vi "FPGA Beam Scanning V1.vi"(1 "Detectors":T1, 2 "Image Acquisition Parameters":T2={"Scan Type"=enum."Sample Scanning", "Scan Mode"=enum."XY", "Fast Axis Frequency (Hz)"=100.0, "Image Format"=128, "Line Accumulations"=1, "Frames Per Capture"=1, "Frames Accumulations"=1, "Image Dimension (um)"=[], "Number of Z Steps"=1, "Z Steps Size (um)"=1.0, "Pixel Size (nm)"=[]} {"Z Steps Size (um)" min=0.0; "Number of Z Steps" min=1; "Frames Accumulations" min=1; "Frames Per Capture" min=1; "Line Accumulations" min=1; "Image Format" items=["64 x 64"=64, "128 x 128"=128, "256 x 256"=256, "512 x 512"=512, "1024 x 1024"=1024, "2048 x 2048"=2048]}) -> ()   [LabVIEW 2016]
uses:
  <vilib>/rvi/interface/nirviReadWriteControl/nirviReadWriteControl.xnode
  <vilib>/rvi/interface/nirviMethod/nirviMethod.xnode
  <vilib>/rvi/errors/niLvFpgaMergeErrorWithErrorCode.vi
  <vilib>/rvi/interface/nirviOpenFPGA/nirviOpenFPGA.xnode
  <vilib>/vision/NI_Vision_Development_Module.lvlib
  <vilib>/rvi/interface/nirviCloseFPGA/nirviCloseFPGA.xnode
  <vilib>/vision/Image Controls.llb/IMAQ Image.ctl
  FPGA Bitfiles/MainSTEDFPGAProj_FPGATarget2_BeamScanningCamb_PyGckhW3v70.lvbitx
  FPGA Target VIs/FPGA-7852R/Beam Scanning Cambridge V1.vi
  <vilib>/FPGAPlugInAG/PCIe-7852R/niLvFpga_Open_PCIe-7852R.vi
  NiFpgaLv.dll
  <vilib>/Utility/error.llb/Error Cluster From Error Code.vi
  <vilib>/rvi/errors/niLvFpgaAdjustHostInterfaceError.vi
  <vilib>/FPGAPlugInAG/PCIe-7852R/niLvFpga_ConfigureFifo_PCIe-7852R.vi
  <vilib>/FPGAPlugInAG/PCIe-7852R/niLvFpga_StartFifo_PCIe-7852R.vi
  <vilib>/FPGAPlugInAG/PCIe-7852R/niLvFpga_ReadFifo_PCIe-7852R.vi
  <vilib>/FPGAPlugInAG/PCIe-7852R/niLvFpga_Run_PCIe-7852R.vi
  <vilib>/FPGAPlugInAG/PCIe-7852R/niLvFpga_Close_PCIe-7852R.vi
  Type Defs/Image Acquisition Parameters.ctl
  Detectors.ctl
panel:
  in  "Trigger Delay Manual (Ticks)":u16=3650
  in  "Adjust Trigger":u16=300
  # "Copyright (C) 2020 Edward S Allgeyer\n\nRedistribution and use in source and binary forms, with or without\nmodification, are permitted provided that the following conditions\nare met:\n\n1. Redistributions of source code must retain the above copyright\n   notice, this list of conditions and the following disclaimer.\n\n2. Redistributions in binary form must reproduce the above copyright\n   notice, this list of conditions and the following disclaimer in\n   the documentation and/or other materials provided with the\n   distribution.\n\n3. Neither the name of the copyright holder nor the names of its\n   contributors may be used to endorse or promote products derived\n   from this software without specific prior written permission.\n\nTHIS SOFTWARE IS PROVIDED BY THE COPYRIGHT HOLDERS AND CONTRIBUTORS\n\"AS IS\" AND ANY EXPRESS OR IMPLIED WARRANTIES, INCLUDING, BUT NOT\nLIMITED TO, THE IMPLIED WARRANTIES OF MERCHANTABILITY AND FITNESS\nFOR A PARTICULAR PURPOSE ARE DISCLAIMED. IN NO EVENT SHALL THE\nCOPYRIGHT HOLDER OR CONTRIBUTORS BE LIABLE FOR ANY DIRECT, INDIRECT,\nINCIDENTAL, SPECIAL, EXEMPLARY, OR CONSEQUENTIAL DAMAGES (INCLUDING,\nBUT NOT LIMITED TO, PROCUREMENT OF SUBSTITUTE GOODS OR SERVICES;\nLOSS OF USE, DATA, OR PROFITS; OR BUSINESS INTERRUPTION) HOWEVER\nCAUSED AND ON ANY THEORY OF LIABILITY, WHETHER IN CONTRACT, STRICT\nLIABILITY, OR TORT (INCLUDING NEGLIGENCE OR OTHERWISE) ARISING IN\nANY WAY OUT OF THE USE OF THIS SOFTWARE, EVEN IF ADVISED OF THE\nPOSSIBILITY OF SUCH DAMAGE."
  # "XY"
  # "Z"
  # "Length"
  # "Height"
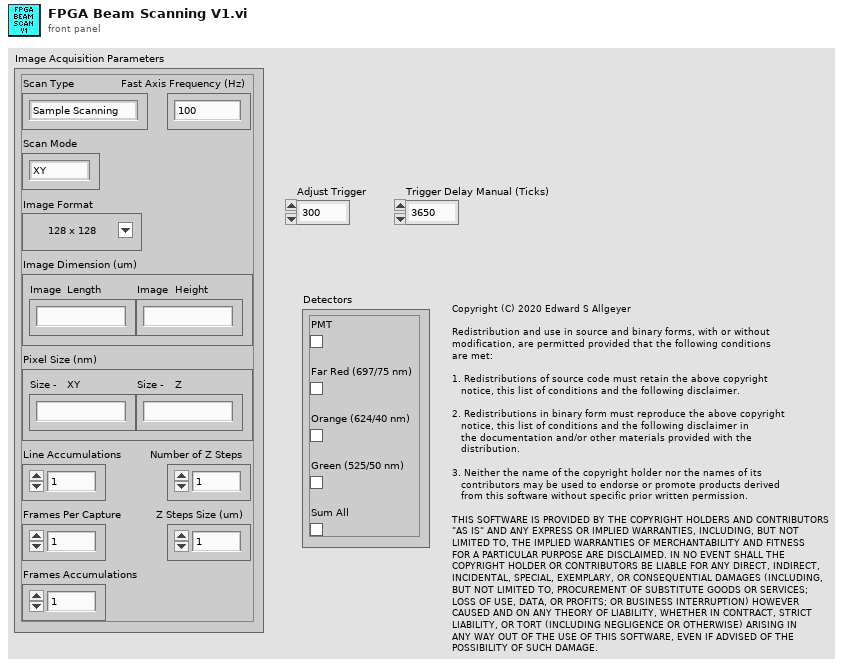
[diagram p1: front panel]
types:
  T1 = typedef "Detectors.ctl" = cluster{"PMT":bool, "Far Red (697/75 nm)":bool, "Orange (624/40 nm)":bool, "Green (525/50 nm)":bool, "Sum All":bool}
  T2 = typedef "Image Acquisition Parameters.ctl" = cluster{"Scan Type":enum16{"Sample Scanning", "Beam Scanning"}, "Scan Mode":enum16{"XY", "XZ", "YZ", "XYZ"}, "Fast Axis Frequency (Hz)":dbl, "Image Format":u16, "Line Accumulations":u16, "Frames Per Capture":u16, "Frames Accumulations":u16, "Image Dimension (um)":dbl[], "Number of Z Steps":u8, "Z Steps Size (um)":dbl, "Pixel Size (nm)":dbl[]}
  T3 = typedef "IMAQ Image.ctl" = refnum<image>
  T4 = enum16{"big-endian, network order", "native, host order", "little-endian"}
  T5 = cluster{"FPGA Sampling Period (ns)":dbl, "Counting Period (us)":dbl, "Samples Per Counting Period":i32, "Start Time (us)":dbl, "Stop Time (us)":dbl, "Normalized Scan End Position":dbl, "Normalized Scan Start Position":dbl}
  T6 = typedef "Scan Parameters.ctl" = cluster{"Fast_Ax_Amp_V":dbl, "Fast_Ax_Off_V":dbl, "Slow_Ax_Amp_V":dbl, "Slow_Ax_Off_V ":dbl, "Slow_Ax_Max_V_VperS":dbl, "Slow_Ax1_Del25ns":i32, "Slow_Ax2_Del25ns":i32, "Stage_X_Off_V":dbl, "Stage_Y_Off_V":dbl, "Stage_Z_Off_V":dbl, "Galvo1_Off_V":dbl, "Galvo2_Off_V":dbl, "Last_Scan_Mode":enum16{"XY", "XZ", "YZ", "XYZ"}, "Current_Scan_Mode":enum16{"XY", "XZ", "YZ", "XYZ"}, "Fly_Back_Lines":u16, "Linear_Ramp_End":u32, "Z_Step_I16":i16, "Z_Start_I16":i16, "Laser_States _U32":u32, "590_Voltage_I16":i16, "775_AOM_Volt_I16":i16, "Blanking OFF":bool, "Unused_Axis_I16":i16}
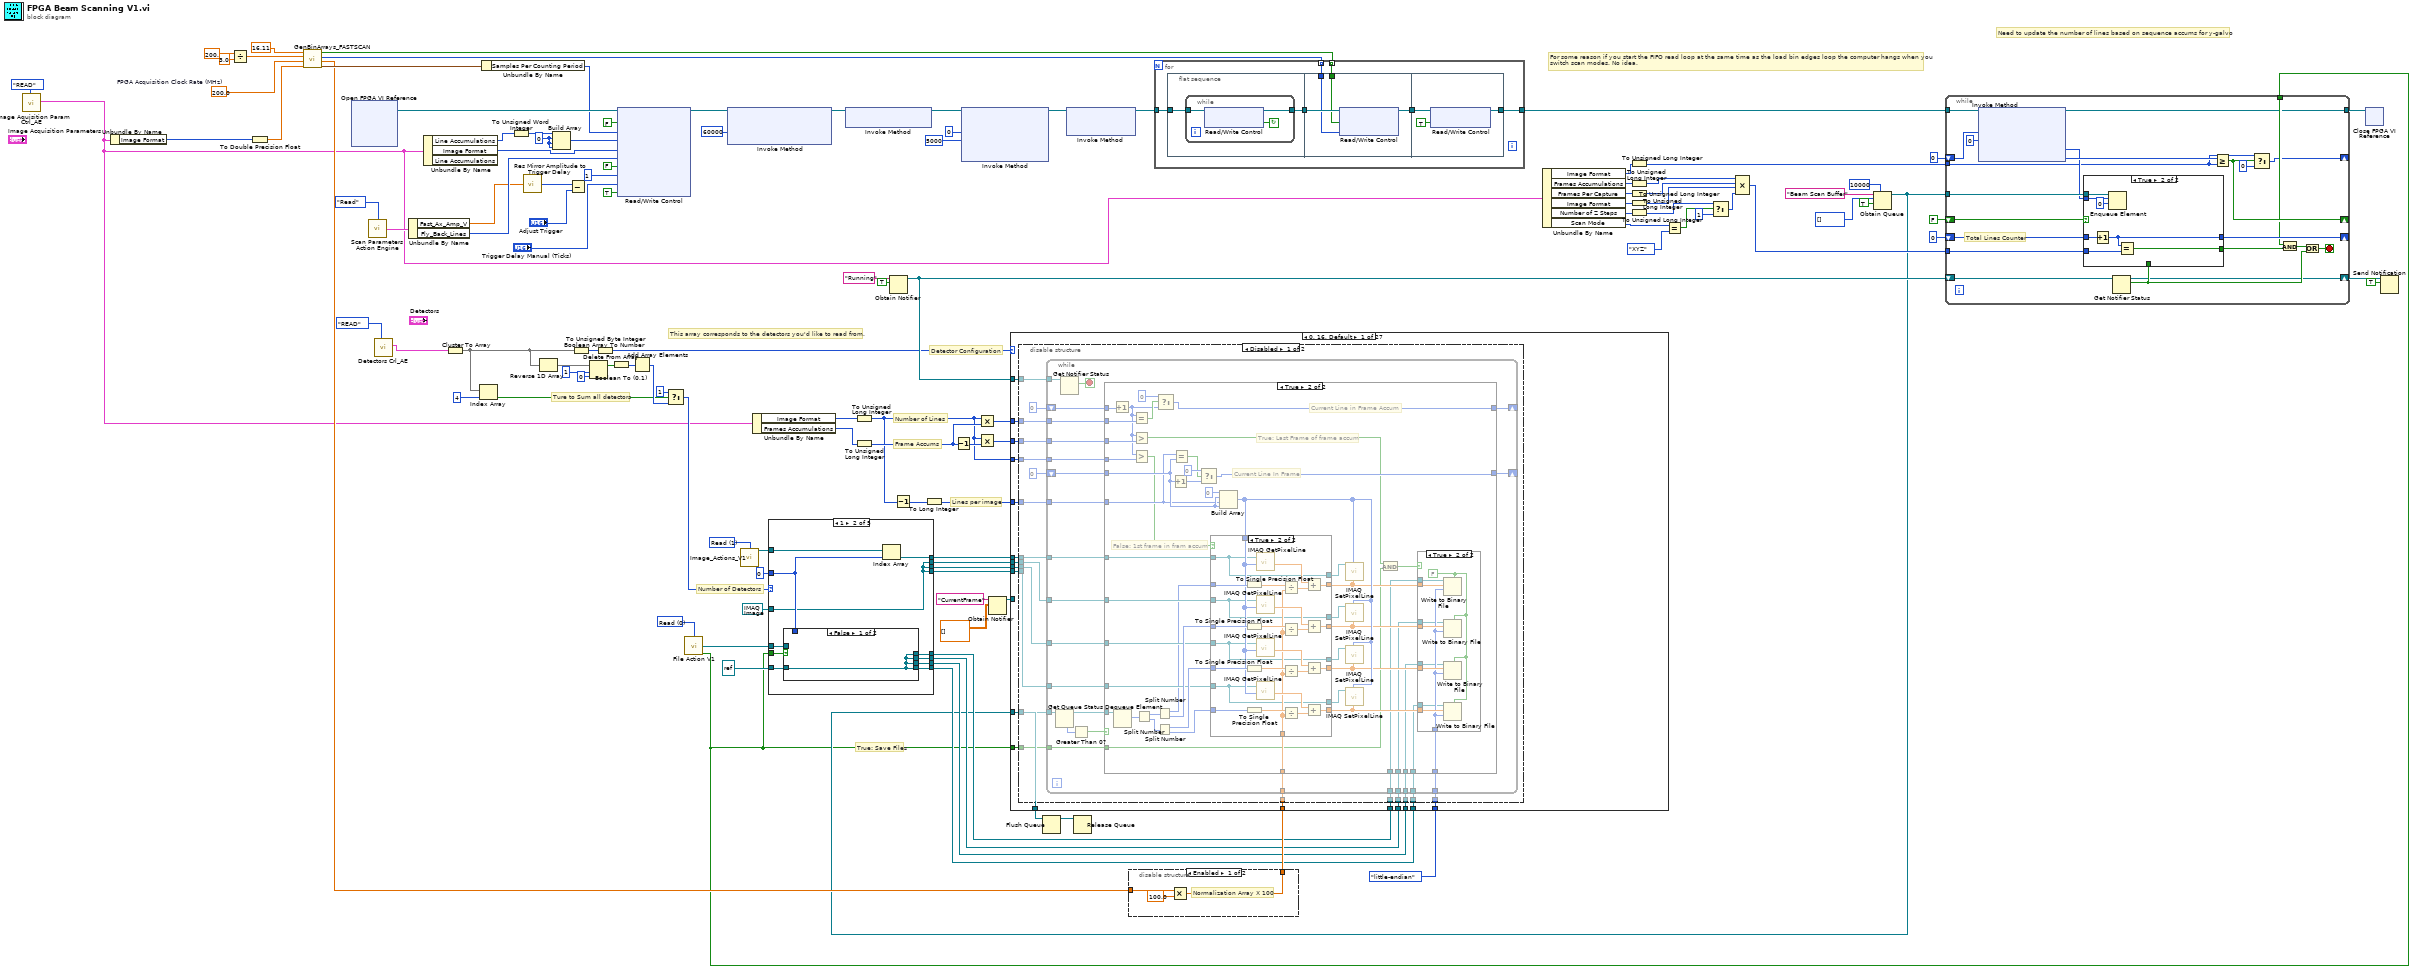
[diagram p0: block diagram]
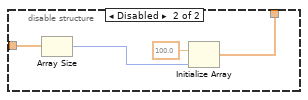
[diagram p2: hidden frame]
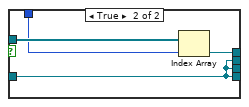
[diagram p4: hidden frame]
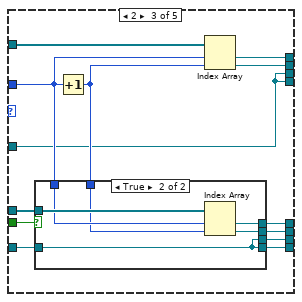
[diagram p5: hidden frame]
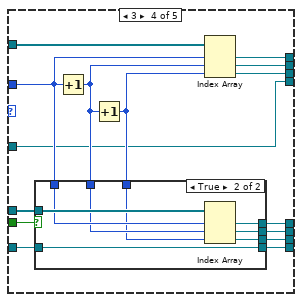
[diagram p7: hidden frame]
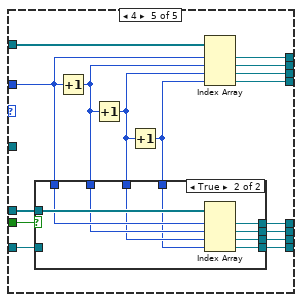
[diagram p9: hidden frame]
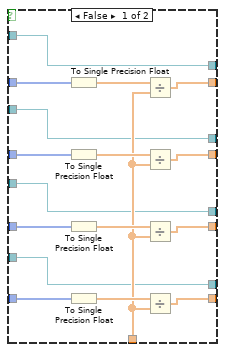
[diagram p13: hidden frame]
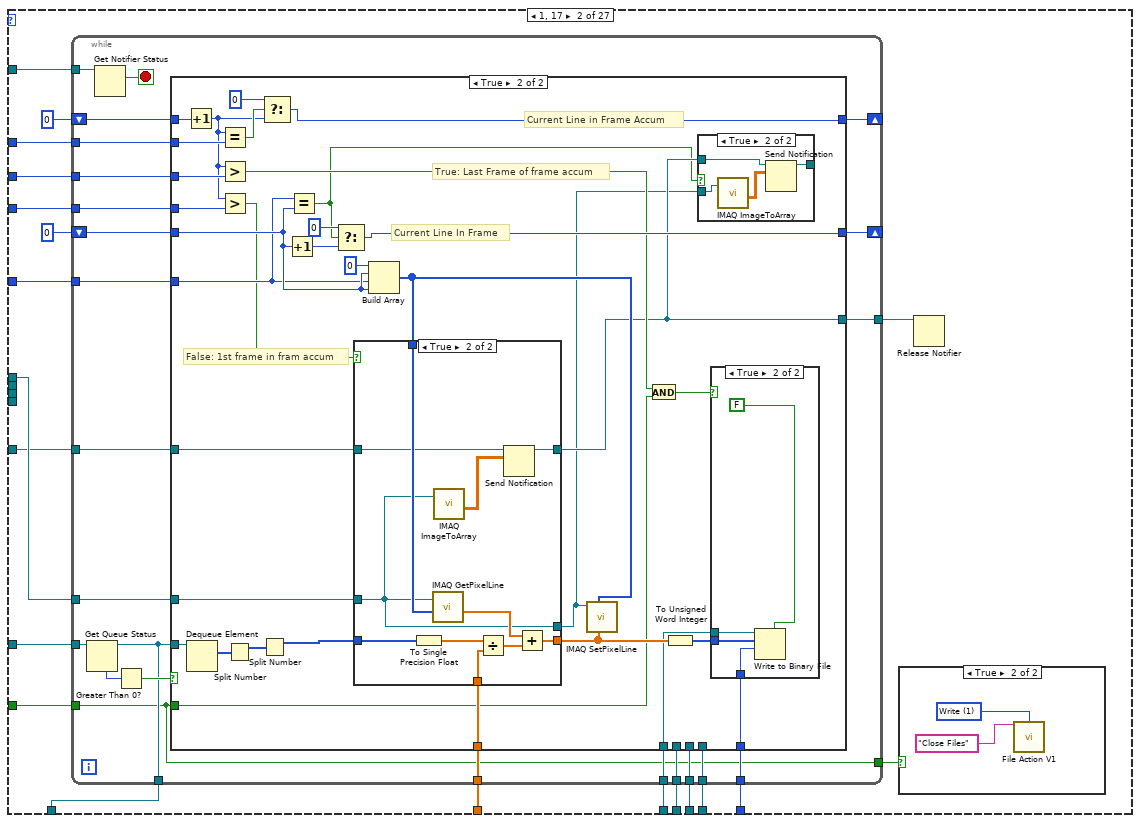
[diagram p15: hidden frame]
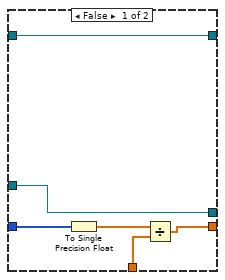
[diagram p20: hidden frame]
diagram:
  w21 = u16 0 items=["Read", "Write"] ("Mode")
  w22 = u16 0 ("element")
  w65 = u16 1 items=["Write", "Read"] ("Mode")
  w113 = 200.0  # FPGA Acquisition Clock Rate (MHz)
  # "This array corresponds to the detectors you'd like to read from."
  # "Ture to Sum all detectors"
  # "Number of Detectors"
  # "Detector Configuration"
  # "Frame Accums"
  # "Number of Lines"
  # "True: Save Files"
  # "Lines per image"
  # "For some reason if you start the FIFO read loop at the same time as the load bin edges loop the computer hangs when you\nswitch scan modes. No idea."
  # "Need to update the number of lines based on sequence accums for y-galvo"
  n1 = call "Image Aquisition Param Ctrl_AE.vi"("Action"=enum16{"READ", "WRITE"}."READ") -> ("Image Acquisition Parameters Out"=w7:T2)  [unwired: 10 in]
  n2 = Unbundle By Name(w7) -> ("Image Format"=w19:u16)
  n3 = Divide(x=200.0, y=3.0) -> (x/y=w110:dbl)
  n4 = To Double Precision Float(number=w19) -> (double precision float=w94:dbl)
  n5 = call "GenBinArrays_FASTSCAN.vi"("Pixels Per Line"=w94, "FPGA Acquisition Clock Rate (MHz)"=w113, "Collection Percent (%)"=w110, "Scan Rate (kHz)"=16.11) -> ("Reported Parameters"=w109:T5, "Normalization Array"=w43:sgl[], "Pre Binned Counts (x100)"=w16:u32[], "FPGA Bin Edges"=w17:bool[])
  n6 = xnode "Open FPGA VI Reference"() -> ("FPGA VI Reference Out"=w117:refnum<k20>)  [unwired: 2 in, 1 out]
  n7 = call "Scan Parameters Action Engine.vi"("Action"=enum16{"Read", "Write"}."Read") -> ("Scan Parameters OUT"=w27:T6)  [unwired: 14 in]
  n8 = call "Detectors Crl_AE.vi"("Action"=enum16{"READ", "WRITE"}."READ") -> ("Detectors Parameters Out"=w5:T1)  [unwired: 10 in]
  n9 = Unbundle By Name(w27) -> ("Fast_Ax_Amp_V"=w18:dbl, "Fly_Back_Lines"=w26:u16)
  n10 = Unbundle By Name(w7) -> ("Line Accumulations"=w32:u16, "Image Format"=w29:u16)  [unwired: 1 out]
  n11 = Cluster To Array(cluster=w5) -> (array=w11:bool[])
  n12 = Index Array(array=w11, index=4) -> (element=w9:bool)
  n13 = Unbundle By Name(w109) -> ("Samples Per Counting Period"=w76:i32)
  n14 = To Unsigned Word Integer(number=w32) -> (unsigned 16bit integer=w31:u16)
  n15 = call "Res Mirror Amplitude to Trigger Delay.vi"("Amplitude (V)"=w18) -> ("Trigger Delay (Ticks)"=w15:u16)
  n16 = Reverse 1D Array(array=w11) -> (reversed array=w48:bool[])
  n17 = Build Array(w31, w22, w22, w22) -> (w30:u16[])
  n18 = Subtract(x=w15, y="Adjust Trigger") -> ()  [unwired: 1 out]
  n19 = Boolean Array To Number(Boolean array=w11) -> (number=w13:u32)
  n20 = Delete From Array(array=w48, length=1, index=0) -> (array with subset deleted=w52:bool[])  [unwired: 1 out]
  n21 = To Unsigned Byte Integer(number=w13) -> (unsigned 8bit integer=w12:u8)
  n22 = Boolean To (0,1)(Boolean=w52) -> (0, 1=w51:i16[])
  n23 = xnode "Read/Write Control"("FPGA VI Reference In"=w117, "Ready For Write"=FALSE, "FPGA Samples"=w76, "Accums Per Line"=w30, "Lines Per Image"=w29, "Dead Lines"=w26, "Line Trigger"=FALSE, "Sequences"=u8 1, "Trigger Delay (Ticks)"="Trigger Delay Manual (Ticks)", "Stop Acquisition"=TRUE) -> ("FPGA VI Reference Out"=w116:refnum<k20>)  [unwired: 1 in, 1 out]
  n24 = Add Array Elements(numeric array=w51) -> (sum=w50:i16)
  n25 = Select(t=i16 1, s=w9, f=w50) -> (s? t:f=w45:i16)
  n26 = call "File Action V1.vi"("Mode"=w21) -> ("File REFs"=w62:refnum<file>[], "Files Open"=w20:bool)  [unwired: 12 in, 1 out]
  n27 = xnode "Invoke Method"("FPGA VI Reference In"=w116, "Requested Depth"=u32 60000) -> ("FPGA VI Reference Out"=w92:refnum<k20>)  [unwired: 1 in, 2 out]
  n28 = call "Image_Actions_V1.vi"("Mode"=w65) -> ("Image REFs OUT"=w64:T3[])  [unwired: 13 in, 1 out]
  n29 = Unbundle By Name(w7) -> ("Image Format"=w85:u16, "Frames Accumulations"=w84:u16)
  n30 = case shown="1" w45 {
    tunnel: [w119 w120 w136 w156 w195] -> w57
    tunnel: [w119 w120 w136 w170 w194] -> w58
    tunnel: [w119 w120 w148 w169 w193] -> w59
    tunnel: [w119 w130 w147 w168 w192] -> w60
    tunnel: 0 ("Offset") -> [_ w126 w143 w164 w188]
    tunnel: w64 -> [_ w129 w146 w167 w191]
    tunnel: T3 refnum ("New Image") -> [w119 w120 w136 w156 _]
    tunnel: w62 -> [_ w127 w144 w165 w189]
    tunnel: w20 -> [_ w128 w145 w166 w190]
    tunnel: [w118 w125 w141 w161 w184] -> w56
    tunnel: [w118 w124 w140 w160 w183] -> w55
    tunnel: [w118 w123 w139 w159 w182] -> w54
    tunnel: [w118 w122 w138 w158 w181] -> w53
    tunnel: refnum<file> refnum ("element") -> [w118 w121 w137 w157 w180]
    frame 0, Default {
    }
    frame 1 {
      n31 = case shown="False" w128 {
        tunnel: w127 -> [_ w135]
        tunnel: w126 -> [_ w134]
        tunnel: [w131 w133] -> w125
        tunnel: [w131 w132] -> w124
        tunnel: [w131 w132] -> w123
        tunnel: [w131 w132] -> w122
        tunnel: w121 -> [w131 w132]
        frame False {
        }
        frame True {
          n32 = Index Array(array=w135, index=w134) -> (element=w133:refnum<file>)
        }
      }
      n33 = Index Array(array=w129, index=w126) -> (element=w130:T3)
    }
    frame 2 {
      n34 = Increment(x=w143) -> (x+1=w142:i32)
      n35 = case shown="True" w145 {
        tunnel: w144 -> [_ w155]
        tunnel: w143 -> [_ w154]
        tunnel: w142 -> [_ w153]
        tunnel: [w149 w152] -> w141
        tunnel: [w149 w151] -> w140
        tunnel: [w149 w150] -> w139
        tunnel: [w149 w150] -> w138
        tunnel: w137 -> [w149 w150]
        frame False {
        }
        frame True {
          n36 = Index Array(array=w155, index #1=w154, index #2=w153) -> (element #1=w152:refnum<file>, element #2=w151:refnum<file>)
        }
      }
      n37 = Index Array(array=w146, index #1=w143, index #2=w142) -> (element #1=w147:T3, element #2=w148:T3)
    }
    frame 3 {
      n38 = Increment(x=w164) -> (x+1=w163:i32)
      n39 = Increment(x=w163) -> (x+1=w162:i32)
      n40 = case shown="True" w166 {
        tunnel: w165 -> [_ w179]
        tunnel: w164 -> [_ w178]
        tunnel: w163 -> [_ w177]
        tunnel: w162 -> [_ w176]
        tunnel: [w171 w175] -> w161
        tunnel: [w171 w174] -> w160
        tunnel: [w171 w173] -> w159
        tunnel: [w171 w172] -> w158
        tunnel: w157 -> [w171 w172]
        frame False {
        }
        frame True {
          n41 = Index Array(array=w179, index #1=w178, index #2=w177, index #3=w176) -> (element #1=w175:refnum<file>, element #2=w174:refnum<file>, element #3=w173:refnum<file>)
        }
      }
      n42 = Index Array(array=w167, index #1=w164, index #2=w163, index #3=w162) -> (element #1=w168:T3, element #2=w169:T3, element #3=w170:T3)
    }
    frame 4 {
      n43 = Increment(x=w188) -> (x+1=w187:i32)
      n44 = Increment(x=w187) -> (x+1=w186:i32)
      n45 = Increment(x=w186) -> (x+1=w185:i32)
      n46 = case shown="True" w190 {
        tunnel: w189 -> [_ w205]
        tunnel: w188 -> [_ w204]
        tunnel: w187 -> [_ w203]
        tunnel: w186 -> [_ w202]
        tunnel: w185 -> [_ w201]
        tunnel: [w196 w200] -> w184
        tunnel: [w196 w199] -> w183
        tunnel: [w196 w198] -> w182
        tunnel: [w196 w197] -> w181
        tunnel: w180 -> [w196 _]
        frame False {
        }
        frame True {
          n47 = Index Array(array=w205, index #1=w204, index #2=w203, index #3=w202, index #4=w201) -> (element #1=w200:refnum<file>, element #2=w199:refnum<file>, element #3=w198:refnum<file>, element #4=w197:refnum<file>)
        }
      }
      n48 = Index Array(array=w191, index #1=w188, index #2=w187, index #3=w186, index #4=w185) -> (element #1=w192:T3, element #2=w193:T3, element #3=w194:T3, element #4=w195:T3)
    }
  }
  n49 = xnode "Invoke Method"("FPGA VI Reference In"=w92) -> ("FPGA VI Reference Out"=w93:refnum<k20>)  [unwired: 1 in, 1 out]
  n50 = To Unsigned Long Integer(number=w85) -> (unsigned 32bit integer=w68:u32)
  n51 = To Unsigned Long Integer(number=w84) -> (unsigned 32bit integer=w69:u32)
  n52 = Obtain Notifier(name (unnamed)="Running", notification data type=TRUE) -> (notifier out=w42:refnum<notifier>)  [unwired: 2 in, 2 out]
  n53 = Decrement(x=w68) -> (x-1=w66:u32)
  n54 = To Long Integer(number=w66) -> (32bit integer=w74:i32)
  n55 = Decrement(x=w69) -> (x-1=w72:u32)
  n56 = xnode "Invoke Method"("FPGA VI Reference In"=w93, "Number of Elements"=u32 0, "Timeout (ms)"=5000) -> ("FPGA VI Reference Out"=w115:refnum<k20>)  [unwired: 1 in, 3 out]
  n57 = Multiply(x=w68, y=w69) -> (x*y=w70:u32)
  n58 = Multiply(x=w68, y=w72) -> (x*y=w71:u32)
  n59 = Obtain Notifier(name (unnamed)="CurrentFrame", notification data type=sgl[][] []) -> (notifier out=w2:refnum<notifier>)  [unwired: 2 in, 2 out]
  n60 = xnode "Invoke Method"("FPGA VI Reference In"=w115) -> ("FPGA VI Reference Out"=w108:refnum<k20>)  [unwired: 2 in, 1 out]
  n61 = disable-structure shown="Enabled" {
    disable-tunnel: [w208 w209] -> w83
    disable-tunnel: w43 -> [w206 w212]
    frame Enabled {
      # "Normalization Array X 100"
      n62 = Multiply(x=w206, y=sgl 100.0) -> (x*y=w208:sgl[])
    }
    frame Disabled {
      n63 = Array Size(array=w212) -> (size(s)=w211:i32)
      n64 = Initialize Array(sgl 100.0 ("element"), w211) -> (w209:sgl[])
    }
  }
  n65 = for {
    tunnel: [w216] -> w81
    tunnel: w108 -> [w215]
    tunnel: w17 -> [w214] mode=indexing
    tunnel: w16 -> [w213] mode=indexing
    n66 = flat-sequence {
      tunnel: [w220] -> w218
      tunnel: w215 -> [w219]
      tunnel: w218 -> [w227]
      tunnel: [w226] -> w217
      tunnel: w214 -> [w225]
      tunnel: w213 -> [w224]
      tunnel: w217 -> [w230]
      tunnel: [w229] -> w216
      frame #0 {
        n67 = while {
          tunnel: [w223] -> w220
          tunnel: w219 -> [w222]
          stop <- w221 continue-if-true
          n68 = xnode "Read/Write Control"("FPGA VI Reference In"=w222) -> ("FPGA VI Reference Out"=w223:refnum<k20>, "Ready For Write"=w221:bool)  [unwired: 1 in, 1 out]
        }
      }
      frame #1 {
        n69 = xnode "Read/Write Control"("FPGA VI Reference In"=w227, "BinEdge"=w225, "PreBinnedValue"=w224) -> ("FPGA VI Reference Out"=w226:refnum<k20>)  [unwired: 1 in, 1 out]
      }
      frame #2 {
        n70 = xnode "Read/Write Control"("FPGA VI Reference In"=w230, "Ready For Write"=TRUE) -> ("FPGA VI Reference Out"=w229:refnum<k20>)  [unwired: 1 in, 1 out]
      }
    }
  }
  n71 = Unbundle By Name(w7) -> ("Image Format"=w100:u16, "Frames Accumulations"=w40:u16, "Frames Per Capture"=w101:u16, "Image Format"=w41:u16, "Number of Z Steps"=w37:u8, "Scan Mode"=w38:enum16{"XY", "XZ", "YZ", "XYZ"})
  n72 = To Unsigned Long Integer(number=w100) -> (unsigned 32bit integer=w107:u32)
  n73 = To Unsigned Long Integer(number=w40) -> (unsigned 32bit integer=w36:u32)
  n74 = To Unsigned Long Integer(number=w101) -> (unsigned 32bit integer=w35:u32)
  n75 = To Unsigned Long Integer(number=w41) -> (unsigned 32bit integer=w34:u32)
  n76 = To Unsigned Long Integer(number=w37) -> (unsigned 32bit integer=w33:u32)
  n77 = Equal?(x=w38, y=enum16{"XY", "XZ", "YZ", "XYZ"}."XYZ") -> (x = y?=w88:bool)
  n78 = Select(t=w33, s=w88, f=u32 1) -> (s? t:f=w87:u32)
  n79 = Compound Arithmetic op=MULTIPLY(w36, w35, w34, w87) -> (w102:u32)
  n80 = Obtain Queue(max queue size (-1, unlimited)=10000, name (unnamed)="Beam Scan Buffer", element data type=u64[] [], create if not found? (T)=TRUE) -> (queue out=w24:refnum<queue>)  [unwired: 1 in, 2 out]
  n81 = case shown="0, 16, Default" w12 {
    tunnel: w74 -> [w247 w411 w517 w617 w726 w825 w934 w1044 w1173 w1272 w1381 w1491 w1619 w1728 w1857 w1987 w2133 w2223 w2314 w2405 w2498 w2589 w2680 w2773 w2863 w2956 w3049]
    tunnel: w20 -> [w244 w408 w514 w614 w723 w822 w931 w1041 w1170 w1269 w1378 w1488 w1616 w1725 w1854 w1984 w2130 w2220 w2311 w2402 w2495 w2586 w2677 w2770 w2860 w2953 w3046]
    tunnel: T4."little-endian" ("byte order (0:big-endian, network order)") -> [w246 w410 w516 w616 w725 w824 w933 w1043 w1172 w1271 w1380 w1490 w1618 w1727 w1856 w1986 w2132 w2222 w2313 w2404 w2497 w2588 w2679 w2772 w2862 w2955 w3048]
    tunnel: w83 -> [w245 w409 w515 w615 w724 w823 w932 w1042 w1171 w1270 w1379 w1489 w1617 w1726 w1855 w1985 w2131 w2221 w2312 w2403 w2496 w2587 w2678 w2771 w2861 w2954 w3047]
    tunnel: w42 -> [w243 w407 w513 w613 w722 w821 w930 w1040 w1169 w1268 w1377 w1487 w1615 w1724 w1853 w1983 w2129 w2219 w2310 w2401 w2494 w2585 w2676 w2769 w2859 w2952 w3045]
    tunnel: w71 -> [w242 w405 w511 w611 w720 w819 w928 w1038 w1167 w1266 w1375 w1485 w1613 w1722 w1851 w1981 w2127 w2217 w2308 w2399 w2492 w2583 w2674 w2767 w2857 w2950 w3043]
    tunnel: w70 -> [w241 w404 w510 w610 w719 w818 w927 w1037 w1166 w1265 w1374 w1484 w1612 w1721 w1850 w1980 w2126 w2216 w2307 w2398 w2491 w2582 w2673 w2766 w2856 w2949 w3042]
    tunnel: w68 -> [w240 w403 w509 w609 w718 w817 w926 w1036 w1165 w1264 w1373 w1483 w1611 w1720 w1849 w1979 w2125 w2215 w2306 w2397 w2490 w2581 w2672 w2765 w2855 w2948 w3041]
    tunnel: w24 -> [w239 w402 w508 w602 w717 w816 w925 w1035 w1164 w1263 w1372 w1482 w1610 w1719 w1848 w1978 w2124 w2214 w2305 w2396 w2489 w2580 w2671 w2764 w2854 w2947 w3040]
    tunnel: w60 -> [w234 w397 w503 w604 w712 w811 w920 w1030 w1159 w1258 w1367 w1477 w1605 w1714 w1843 w1973 w2119 w2209 w2300 w2391 w2484 w2575 w2666 w2759 w2849 w2942 w3035]
    tunnel: w59 -> [w233 _ _ w603 _ w810 w919 w1029 _ w1257 w1366 w1476 w1604 w1713 w1842 w1972 _ _ _ _ _ _ _ _ _ _ _]
    tunnel: w58 -> [w232 _ _ _ _ _ _ w1028 _ _ _ w1475 _ w1712 w1841 w1971 _ _ _ _ _ _ _ _ _ _ _]
    tunnel: w57 -> [w231 _ _ _ _ _ _ _ _ _ _ _ _ _ _ w1970 _ _ _ _ _ _ _ _ _ _ _]
    tunnel: [w239 w396 w508 w601 w717 w816 w925 w1035 w1164 w1263 w1372 w1482 w1610 w1719 w1848 w1978 w2124 w2214 w2305 w2396 w2489 w2580 w2671 w2764 w2854 w2947 w3040] -> w23
    tunnel: w56 -> [w238 w401 w507 w608 w716 w815 w924 w1034 w1163 w1262 w1371 w1481 w1609 w1718 w1847 w1977 w2123 w2213 w2304 w2395 w2488 w2579 w2670 w2763 w2853 w2946 w3039]
    tunnel: w55 -> [w237 w400 w506 w607 w715 w814 w923 w1033 w1162 w1261 w1370 w1480 w1608 w1717 w1846 w1976 w2122 w2212 w2303 w2394 w2487 w2578 w2669 w2762 w2852 w2945 w3038]
    tunnel: w54 -> [w236 w399 w505 w606 w714 w813 w922 w1032 w1161 w1260 w1369 w1479 w1607 w1716 w1845 w1975 w2121 w2211 w2302 w2393 w2486 w2577 w2668 w2761 w2851 w2944 w3037]
    tunnel: w53 -> [w235 w398 w504 w605 w713 w812 w921 w1031 w1160 w1259 w1368 w1478 w1606 w1715 w1844 w1974 w2120 w2210 w2301 w2392 w2485 w2576 w2667 w2760 w2850 w2943 w3036]
    tunnel: w2 -> [_ w394 w502 _ w711 _ _ _ w1158 _ _ _ _ _ _ _ _ _ _ _ _ _ _ _ _ _ _]
    frame 0, 16, Default {
      n82 = disable-structure shown="Disabled" {
        disable-tunnel: w247 -> [w265 _]
        disable-tunnel: w246 -> [w264 _]
        disable-tunnel: w245 -> [w263 _]
        disable-tunnel: w244 -> [w262 _]
        disable-tunnel: w243 -> [w261 _]
        disable-tunnel: w242 -> [w259 _]
        disable-tunnel: w241 -> [w258 _]
        disable-tunnel: w240 -> [w257 _]
        disable-tunnel: w239 -> [w256 _]
        disable-tunnel: w238 -> [w255 _]
        disable-tunnel: w237 -> [w254 _]
        disable-tunnel: w236 -> [w253 _]
        disable-tunnel: w235 -> [w252 _]
        disable-tunnel: w234 -> [w251 _]
        disable-tunnel: w233 -> [w250 _]
        disable-tunnel: w232 -> [w249 _]
        disable-tunnel: w231 -> [w248 _]
        frame Disabled {
          n83 = while {
            shift-right: [w289] -> _
            shift-left: 0 -> [w290]
            tunnel: w265 -> [w291]
            tunnel: w264 -> [w288]
            tunnel: w263 -> [w287]
            tunnel: w262 -> [w286]
            tunnel: w261 -> [w282]
            shift-right: [w279] -> _
            shift-left: u32 0 -> [w280]
            tunnel: w259 -> [w278]
            tunnel: w258 -> [w277]
            tunnel: w257 -> [w276]
            tunnel: w256 -> [w275]
            tunnel: w251 -> [w274]
            tunnel: w250 -> [w273]
            tunnel: w249 -> [w272]
            tunnel: w248 -> [w271]
            tunnel: w255 -> [w270]
            tunnel: w254 -> [w269]
            tunnel: w253 -> [w268]
            tunnel: w252 -> [w267]
            stop <- w281 stop-if-true
            n84 = Get Queue Status(queue=w275) -> (queue out=w283:refnum<queue>, # elements in queue=w285:i32)  [unwired: 2 in, 6 out]
            n85 = Get Notifier Status(notifier=w282) -> (current notification=w281:bool)  [unwired: 1 in, 4 out]
            n86 = Greater Than 0?(x=w285) -> (x > 0?=w284:bool)
            n87 = case shown="True" w284 {
              tunnel: w291 -> [_ w328]
              tunnel: w290 -> [w293 w329]
              tunnel: [w293 w327] -> w289
              tunnel: w288 -> [_ w321]
              tunnel: w287 -> [_ w320]
              tunnel: w286 -> [_ w310]
              tunnel: w283 -> [_ w319]
              tunnel: w280 -> [w292 w316]
              tunnel: [w292 w315] -> w279
              tunnel: w278 -> [_ w314]
              tunnel: w277 -> [_ w313]
              tunnel: w276 -> [_ w308]
              tunnel: w274 -> [_ w306]
              tunnel: w273 -> [_ w305]
              tunnel: w272 -> [_ w304]
              tunnel: w271 -> [_ w303]
              tunnel: w270 -> [_ w297]
              tunnel: w269 -> [_ w296]
              tunnel: w268 -> [_ w295]
              tunnel: w267 -> [_ w294]
              frame False {
              }
              frame True {
                # "False: 1st frame in fram accum"
                # "True: Last Frame of frame accum"
                # "Current Line in Frame Accum"
                # "Current Line In Frame"
                n88 = Increment(x=w316) -> (x+1=w309:u32)
                n89 = Dequeue Element(queue=w319) -> (element=w338:u64[])  [unwired: 2 in, 3 out]
                n90 = Equal?(x=w309, y=w313) -> (x = y?=w318:bool)
                n91 = Greater?(x=w309, y=w314) -> (0:w311:bool)
                n92 = Greater?(x=w309, y=w308) -> (0:w307:bool)
                n93 = Split Number(x=w338) -> (hi(x)=w339:u32[], lo(x)=w337:u32[])
                n94 = Split Number(x=w339) -> (hi(x)=w298:u16[], lo(x)=w336:u16[])
                n95 = Split Number(x=w337) -> (hi(x)=w335:u16[], lo(x)=w334:u16[])
                n96 = Select(t=u32 0, s=w318, f=w309) -> (s? t:f=w315:u32)
                n97 = Increment(x=w329) -> (x+1=w331:i32)
                n98 = Equal?(x=w328, y=w329) -> (x = y?=w330:bool)
                n99 = Select(t=0, s=w330, f=w331) -> (s? t:f=w327:i32)
                n100 = Build Array(0, w329, w328, w329) -> (w326:i32[])
                n101 = case shown="True" w307 {
                  tunnel: w298 -> [w365 w392]
                  tunnel: w336 -> [w360 w391]
                  tunnel: w335 -> [w359 w390]
                  tunnel: w334 -> [w358 w389]
                  tunnel: [w356 w381] -> w323
                  tunnel: [w357 w380] -> w324
                  tunnel: [w364 w379] -> w325
                  tunnel: [w355 w378] -> w322
                  tunnel: w326 -> [_ w373]
                  tunnel: w320 -> [w354 w371]
                  tunnel: w306 -> [w353 w368]
                  tunnel: w305 -> [w352 w369]
                  tunnel: w304 -> [w351 w370]
                  tunnel: w303 -> [w350 w367]
                  tunnel: [w351 w370] -> w300
                  tunnel: [w352 w369] -> w301
                  tunnel: [w353 w368] -> w302
                  tunnel: [w350 w367] -> w299
                  frame False {
                    n102 = To Single Precision Float(number=w365) -> (single precision float=w366:sgl[])
                    n103 = To Single Precision Float(number=w360) -> (single precision float=w363:sgl[])
                    n104 = To Single Precision Float(number=w359) -> (single precision float=w362:sgl[])
                    n105 = To Single Precision Float(number=w358) -> (single precision float=w361:sgl[])
                    n106 = Divide(x=w366, y=w354) -> (x/y=w364:sgl[])
                    n107 = Divide(x=w363, y=w354) -> (x/y=w357:sgl[])
                    n108 = Divide(x=w362, y=w354) -> (x/y=w356:sgl[])
                    n109 = Divide(x=w361, y=w354) -> (x/y=w355:sgl[])
                  }
                  frame True {
                    n110 = To Single Precision Float(number=w392) -> (single precision float=w372:sgl[])
                    n111 = To Single Precision Float(number=w391) -> (single precision float=w388:sgl[])
                    n112 = To Single Precision Float(number=w390) -> (single precision float=w387:sgl[])
                    n113 = To Single Precision Float(number=w389) -> (single precision float=w386:sgl[])
                    n114 = call "IMAQ GetPixelLine"("Line Coordinates"=w373, "Image"=w368) -> ("Pixels Line (Float)"=w377:sgl[])  [unwired: 2 in, 4 out]
                    n115 = call "IMAQ GetPixelLine"("Line Coordinates"=w373, "Image"=w369) -> ("Pixels Line (Float)"=w376:sgl[])  [unwired: 2 in, 4 out]
                    n116 = call "IMAQ GetPixelLine"("Line Coordinates"=w373, "Image"=w370) -> ("Pixels Line (Float)"=w375:sgl[])  [unwired: 2 in, 4 out]
                    n117 = call "IMAQ GetPixelLine"("Line Coordinates"=w373, "Image"=w367) -> ("Pixels Line (Float)"=w374:sgl[])  [unwired: 2 in, 4 out]
                    n118 = Divide(x=w372, y=w371) -> (x/y=w385:sgl[])
                    n119 = Divide(x=w388, y=w371) -> (x/y=w384:sgl[])
                    n120 = Divide(x=w387, y=w371) -> (x/y=w383:sgl[])
                    n121 = Divide(x=w386, y=w371) -> (x/y=w382:sgl[])
                    n122 = Add(x=w377, y=w385) -> (x+y=w379:sgl[])
                    n123 = Add(x=w376, y=w384) -> (x+y=w380:sgl[])
                    n124 = Add(x=w375, y=w383) -> (x+y=w381:sgl[])
                    n125 = Add(x=w374, y=w382) -> (x+y=w378:sgl[])
                  }
                }
                n126 = call "IMAQ SetPixelLine"("Pixels Line (Float)"=w325, "Line Coordinates"=w326, "Image"=w302) -> ()  [unwired: 7 in, 2 out]
                n127 = call "IMAQ SetPixelLine"("Pixels Line (Float)"=w324, "Line Coordinates"=w326, "Image"=w301) -> ()  [unwired: 7 in, 2 out]
                n128 = call "IMAQ SetPixelLine"("Pixels Line (Float)"=w323, "Line Coordinates"=w326, "Image"=w300) -> ()  [unwired: 7 in, 2 out]
                n129 = call "IMAQ SetPixelLine"("Pixels Line (Float)"=w322, "Line Coordinates"=w326, "Image"=w299) -> ()  [unwired: 7 in, 2 out]
                n130 = And(x=w311, y=w310) -> (x .and. y?=w312:bool)
                n131 = case shown="True" w312 {
                  tunnel: w325 -> [_ w349]
                  tunnel: w324 -> [_ w348]
                  tunnel: w323 -> [_ w347]
                  tunnel: w322 -> [_ w346]
                  tunnel: w321 -> [_ w344]
                  tunnel: w297 -> [_ w343]
                  tunnel: w296 -> [_ w342]
                  tunnel: w295 -> [_ w341]
                  tunnel: w294 -> [_ w340]
                  frame False {
                  }
                  frame True {
                    w345 = FALSE ("prepend array or string size? (T)")
                    n132 = Write to Binary File(file (use dialog)=w343, data=w349, 5:w345, 9:w344) -> ()  [unwired: 2 in, 3 out]
                    n133 = Write to Binary File(file (use dialog)=w342, data=w348, 5:w345, 9:w344) -> ()  [unwired: 2 in, 3 out]
                    n134 = Write to Binary File(file (use dialog)=w341, data=w347, 5:w345, 9:w344) -> ()  [unwired: 2 in, 3 out]
                    n135 = Write to Binary File(file (use dialog)=w340, data=w346, 5:w345, 9:w344) -> ()  [unwired: 2 in, 3 out]
                  }
                }
              }
            }
          }
        }
        frame Enabled {
        }
      }
    }
    frame 1, 17 {
      n136 = while {
        shift-right: [w436] -> _
        shift-left: 0 -> [w437]
        tunnel: w411 -> [w438]
        tunnel: w410 -> [w435]
        tunnel: w409 -> [w434]
        tunnel: w408 -> [w417]
        tunnel: w407 -> [w431]
        shift-right: [w428] -> _
        shift-left: u32 0 -> [w429]
        tunnel: w405 -> [w427]
        tunnel: w404 -> [w426]
        tunnel: w403 -> [w425]
        tunnel: w402 -> [w424]
        tunnel: w397 -> [w423]
        tunnel: w401 -> [w422]
        tunnel: w400 -> [w421]
        tunnel: w399 -> [w420]
        tunnel: w398 -> [w419]
        tunnel: [w418] -> w396
        tunnel: [w417] -> w395
        tunnel: w394 -> [w416]
        tunnel: [w415] -> w393
        stop <- w430 stop-if-true
        n137 = Get Queue Status(queue=w424) -> (queue out=w418:refnum<queue>, # elements in queue=w433:i32)  [unwired: 2 in, 6 out]
        n138 = Get Notifier Status(notifier=w431) -> (current notification=w430:bool)  [unwired: 1 in, 4 out]
        n139 = Greater Than 0?(x=w433) -> (x > 0?=w432:bool)
        n140 = case shown="True" w432 {
          tunnel: w438 -> [_ w468]
          tunnel: w437 -> [w441 w469]
          tunnel: [w441 w467] -> w436
          tunnel: w435 -> [_ w464]
          tunnel: w434 -> [_ w463]
          tunnel: w417 -> [_ w447]
          tunnel: w418 -> [_ w462]
          tunnel: w429 -> [w440 w459]
          tunnel: [w440 w458] -> w428
          tunnel: w427 -> [_ w457]
          tunnel: w426 -> [_ w456]
          tunnel: w425 -> [_ w452]
          tunnel: w423 -> [_ w450]
          tunnel: w422 -> [_ w449]
          tunnel: w421 -> [_ _]
          tunnel: w420 -> [_ _]
          tunnel: w419 -> [_ _]
          tunnel: w416 -> [w439 w446]
          tunnel: [w439 w445] -> w415
          frame False {
          }
          frame True {
            # "False: 1st frame in fram accum"
            # "True: Last Frame of frame accum"
            # "Current Line in Frame Accum"
            # "Current Line In Frame"
            n141 = Increment(x=w459) -> (x+1=w453:u32)
            n142 = Dequeue Element(queue=w462) -> (element=w473:u64[])  [unwired: 2 in, 3 out]
            n143 = Equal?(x=w453, y=w456) -> (x = y?=w461:bool)
            n144 = Greater?(x=w453, y=w457) -> (0:w454:bool)
            n145 = Greater?(x=w453, y=w452) -> (0:w451:bool)
            n146 = Split Number(x=w473) -> (hi(x)=w474:u32[])  [unwired: 1 out]
            n147 = Split Number(x=w474) -> (hi(x)=w448:u16[])  [unwired: 1 out]
            n148 = Select(t=u32 0, s=w461, f=w453) -> (s? t:f=w458:u32)
            n149 = Increment(x=w469) -> (x+1=w470:i32)
            n150 = Equal?(x=w468, y=w469) -> (x = y?=w443:bool)
            n151 = Select(t=0, s=w443, f=w470) -> (s? t:f=w467:i32)
            n152 = Build Array(0, w469, w468, w469) -> (w466:i32[])
            n153 = case shown="True" w451 {
              tunnel: w448 -> [w488 w500]
              tunnel: [w487 w497] -> w465
              tunnel: w466 -> [_ w495]
              tunnel: w463 -> [w486 w494]
              tunnel: w450 -> [w485 w493]
              tunnel: [w485 w493] -> w444
              tunnel: w446 -> [w484 w492]
              tunnel: [w484 w490] -> w445
              frame False {
                n154 = To Single Precision Float(number=w488) -> (single precision float=w489:sgl[])
                n155 = Divide(x=w489, y=w486) -> (x/y=w487:sgl[])
              }
              frame True {
                n156 = To Single Precision Float(number=w500) -> (single precision float=w499:sgl[])
                n157 = call "IMAQ GetPixelLine"("Line Coordinates"=w495, "Image"=w493) -> ("Pixels Line (Float)"=w496:sgl[])  [unwired: 2 in, 4 out]
                n158 = call "IMAQ ImageToArray"("Image"=w493) -> ("Image Pixels (Float)"=w491:sgl[][])  [unwired: 3 in, 4 out]
                n159 = Divide(x=w499, y=w494) -> (x/y=w498:sgl[])
                n160 = Send Notification(notification=w491, notifier=w492) -> (notifier out=w490:refnum<notifier>)  [unwired: 1 in, 1 out]
                n161 = Add(x=w496, y=w498) -> (x+y=w497:sgl[])
              }
            }
            n162 = call "IMAQ SetPixelLine"("Pixels Line (Float)"=w465, "Line Coordinates"=w466, "Image"=w444) -> ()  [unwired: 7 in, 2 out]
            n163 = And(x=w454, y=w447) -> (x .and. y?=w455:bool)
            n164 = To Unsigned Word Integer(number=w465) -> (unsigned 16bit integer=w442:u16[])
            n165 = case shown="True" w443 {
              tunnel: w444 -> [_ w478]
              tunnel: w445 -> [w475 w477]
              tunnel: [w475 w476] -> _
              frame False {
              }
              frame True {
                n166 = call "IMAQ ImageToArray"("Image"=w478) -> ("Image Pixels (Float)"=w479:sgl[][])  [unwired: 3 in, 4 out]
                n167 = Send Notification(notification=w479, notifier=w477) -> (notifier out=w476:refnum<notifier>)  [unwired: 1 in, 1 out]
              }
            }
            n168 = case shown="True" w455 {
              tunnel: w442 -> [_ w483]
              tunnel: w464 -> [_ w481]
              tunnel: w449 -> [_ w480]
              frame False {
              }
              frame True {
                n169 = Write to Binary File(file (use dialog)=w480, data=w483, 5:FALSE ("prepend array or string size? (T)"), 9:w481) -> ()  [unwired: 2 in, 3 out]
              }
            }
          }
        }
      }
      n170 = case shown="True" w395 {
        frame False {
        }
        frame True {
          w414 = u16 1 items=["Read", "Write"] ("Mode")
          n171 = call "File Action V1.vi"("Action"="Close Files", "Mode"=w414) -> ()  [unwired: 11 in, 3 out]
        }
      }
      n172 = Release Notifier(notifier=w393) -> ()  [unwired: 2 in, 3 out]
    }
    frame 2, 18 {
      n173 = while {
        shift-right: [w540] -> _
        shift-left: 0 -> [w541]
        tunnel: w517 -> [w542]
        tunnel: w516 -> [w539]
        tunnel: w515 -> [w538]
        tunnel: w514 -> [w537]
        tunnel: w513 -> [w533]
        shift-right: [w530] -> _
        shift-left: u32 0 -> [w531]
        tunnel: w511 -> [w529]
        tunnel: w510 -> [w528]
        tunnel: w509 -> [w527]
        tunnel: w508 -> [w526]
        tunnel: w503 -> [w525]
        tunnel: w507 -> [w524]
        tunnel: w506 -> [w523]
        tunnel: w505 -> [w522]
        tunnel: w504 -> [w521]
        tunnel: w502 -> [w520]
        tunnel: [w519] -> w501
        stop <- w532 stop-if-true
        n174 = Get Queue Status(queue=w526) -> (queue out=w534:refnum<queue>, # elements in queue=w536:i32)  [unwired: 2 in, 6 out]
        n175 = Get Notifier Status(notifier=w533) -> (current notification=w532:bool)  [unwired: 1 in, 4 out]
        n176 = Greater Than 0?(x=w536) -> (x > 0?=w535:bool)
        n177 = case shown="True" w535 {
          tunnel: w542 -> [_ w572]
          tunnel: w541 -> [w545 w573]
          tunnel: [w545 w571] -> w540
          tunnel: w539 -> [_ w568]
          tunnel: w538 -> [_ w567]
          tunnel: w537 -> [_ w557]
          tunnel: w534 -> [_ w566]
          tunnel: w531 -> [w544 w563]
          tunnel: [w544 w562] -> w530
          tunnel: w529 -> [_ w561]
          tunnel: w528 -> [_ w560]
          tunnel: w527 -> [_ w555]
          tunnel: w525 -> [_ w553]
          tunnel: w524 -> [_ w552]
          tunnel: w523 -> [_ _]
          tunnel: w522 -> [_ _]
          tunnel: w521 -> [_ _]
          tunnel: w520 -> [w543 w549]
          tunnel: [w543 w548] -> w519
          frame False {
          }
          frame True {
            # "False: 1st frame in fram accum"
            # "True: Last Frame of frame accum"
            # "Current Line in Frame Accum"
            # "Current Line In Frame"
            n178 = Increment(x=w563) -> (x+1=w556:u32)
            n179 = Dequeue Element(queue=w566) -> (element=w577:u64[])  [unwired: 2 in, 3 out]
            n180 = Equal?(x=w556, y=w560) -> (x = y?=w565:bool)
            n181 = Greater?(x=w556, y=w561) -> (0:w558:bool)
            n182 = Greater?(x=w556, y=w555) -> (0:w554:bool)
            n183 = Split Number(x=w577) -> (hi(x)=w578:u32[])  [unwired: 1 out]
            n184 = Split Number(x=w578) -> (lo(x)=w551:u16[])  [unwired: 1 out]
            n185 = Select(t=u32 0, s=w565, f=w556) -> (s? t:f=w562:u32)
            n186 = Increment(x=w573) -> (x+1=w574:i32)
            n187 = Equal?(x=w572, y=w573) -> (x = y?=w547:bool)
            n188 = Select(t=0, s=w547, f=w574) -> (s? t:f=w571:i32)
            n189 = Build Array(0, w573, w572, w573) -> (w570:i32[])
            n190 = case shown="False" w554 {
              tunnel: w551 -> [w591 w600]
              tunnel: [w590 w597] -> w569
              tunnel: w570 -> [_ w595]
              tunnel: w567 -> [w589 w594]
              tunnel: w553 -> [w588 w593]
              tunnel: [w588 w593] -> w550
              frame False {
                n191 = To Single Precision Float(number=w591) -> (single precision float=w592:sgl[])
                n192 = Divide(x=w592, y=w589) -> (x/y=w590:sgl[])
              }
              frame True {
                n193 = To Single Precision Float(number=w600) -> (single precision float=w599:sgl[])
                n194 = call "IMAQ GetPixelLine"("Line Coordinates"=w595, "Image"=w593) -> ("Pixels Line (Float)"=w596:sgl[])  [unwired: 2 in, 4 out]
                n195 = Divide(x=w599, y=w594) -> (x/y=w598:sgl[])
                n196 = Add(x=w596, y=w598) -> (x+y=w597:sgl[])
              }
            }
            n197 = call "IMAQ SetPixelLine"("Pixels Line (Float)"=w569, "Line Coordinates"=w570, "Image"=w550) -> ()  [unwired: 7 in, 2 out]
            n198 = And(x=w558, y=w557) -> (x .and. y?=w559:bool)
            n199 = To Unsigned Word Integer(number=w569) -> (unsigned 16bit integer=w546:u16[])
            n200 = case shown="True" w547 {
              tunnel: w550 -> [_ w582]
              tunnel: w549 -> [w579 w581]
              tunnel: [w579 w580] -> w548
              frame False {
              }
              frame True {
                n201 = call "IMAQ ImageToArray"("Image"=w582) -> ("Image Pixels (Float)"=w583:sgl[][])  [unwired: 3 in, 4 out]
                n202 = Send Notification(notification=w583, notifier=w581) -> (notifier out=w580:refnum<notifier>)  [unwired: 1 in, 1 out]
              }
            }
            n203 = case shown="True" w559 {
              tunnel: w546 -> [_ w587]
              tunnel: w568 -> [_ w585]
              tunnel: w552 -> [_ w584]
              frame False {
              }
              frame True {
                n204 = Write to Binary File(file (use dialog)=w584, data=w587, 5:FALSE ("prepend array or string size? (T)"), 9:w585) -> ()  [unwired: 2 in, 3 out]
              }
            }
          }
        }
      }
      n205 = Release Notifier(notifier=w501) -> ()  [unwired: 2 in, 3 out]
    }
    frame 3 {
      n206 = while {
        shift-right: [w639] -> _
        shift-left: 0 -> [w640]
        tunnel: w617 -> [w641]
        tunnel: w616 -> [w638]
        tunnel: w615 -> [w637]
        tunnel: w614 -> [w636]
        tunnel: w613 -> [w633]
        shift-right: [w630] -> _
        shift-left: u32 0 -> [w631]
        tunnel: w611 -> [w629]
        tunnel: w610 -> [w628]
        tunnel: w609 -> [w627]
        tunnel: w602 -> [w626]
        tunnel: w604 -> [w625]
        tunnel: w603 -> [w624]
        tunnel: w608 -> [w623]
        tunnel: w607 -> [w622]
        tunnel: w606 -> [w621]
        tunnel: w605 -> [w620]
        tunnel: [w619] -> w601
        stop <- w632 stop-if-true
        n207 = Get Queue Status(queue=w626) -> (queue out=w619:refnum<queue>, # elements in queue=w635:i32)  [unwired: 2 in, 6 out]
        n208 = Get Notifier Status(notifier=w633) -> (current notification=w632:bool)  [unwired: 1 in, 4 out]
        n209 = Greater Than 0?(x=w635) -> (x > 0?=w634:bool)
        n210 = case shown="True" w634 {
          tunnel: w641 -> [_ w673]
          tunnel: w640 -> [w643 w674]
          tunnel: [w643 w672] -> w639
          tunnel: w638 -> [_ w668]
          tunnel: w637 -> [_ w667]
          tunnel: w636 -> [_ w657]
          tunnel: w619 -> [_ w666]
          tunnel: w631 -> [w642 w663]
          tunnel: [w642 w662] -> w630
          tunnel: w629 -> [_ w661]
          tunnel: w628 -> [_ w660]
          tunnel: w627 -> [_ w655]
          tunnel: w625 -> [_ w653]
          tunnel: w624 -> [_ w652]
          tunnel: w623 -> [_ w649]
          tunnel: w622 -> [_ w648]
          tunnel: w621 -> [_ _]
          tunnel: w620 -> [_ _]
          frame False {
          }
          frame True {
            # "False: 1st frame in fram accum"
            # "True: Last Frame of frame accum"
            # "Current Line in Frame Accum"
            # "Current Line In Frame"
            n211 = Increment(x=w663) -> (x+1=w656:u32)
            n212 = Dequeue Element(queue=w666) -> (element=w679:u64[])  [unwired: 2 in, 3 out]
            n213 = Equal?(x=w656, y=w660) -> (x = y?=w665:bool)
            n214 = Greater?(x=w656, y=w661) -> (0:w658:bool)
            n215 = Greater?(x=w656, y=w655) -> (0:w654:bool)
            n216 = Split Number(x=w679) -> (hi(x)=w680:u32[])  [unwired: 1 out]
            n217 = Split Number(x=w680) -> (hi(x)=w647:u16[], lo(x)=w646:u16[])
            n218 = Select(t=u32 0, s=w665, f=w656) -> (s? t:f=w662:u32)
            n219 = Increment(x=w674) -> (x+1=w676:i32)
            n220 = Equal?(x=w673, y=w674) -> (x = y?=w675:bool)
            n221 = Select(t=0, s=w675, f=w676) -> (s? t:f=w672:i32)
            n222 = Build Array(0, w674, w673, w674) -> (w671:i32[])
            n223 = case shown="True" w654 {
              tunnel: w647 -> [w693 w709]
              tunnel: w646 -> [w692 w708]
              tunnel: [w690 w703] -> w669
              tunnel: [w691 w702] -> w670
              tunnel: w671 -> [_ w699]
              tunnel: w667 -> [w689 w698]
              tunnel: w653 -> [w688 w696]
              tunnel: w652 -> [w687 w697]
              tunnel: [w687 w697] -> w650
              tunnel: [w688 w696] -> w651
              frame False {
                n224 = To Single Precision Float(number=w693) -> (single precision float=w695:sgl[])
                n225 = To Single Precision Float(number=w692) -> (single precision float=w694:sgl[])
                n226 = Divide(x=w695, y=w689) -> (x/y=w691:sgl[])
                n227 = Divide(x=w694, y=w689) -> (x/y=w690:sgl[])
              }
              frame True {
                n228 = To Single Precision Float(number=w709) -> (single precision float=w707:sgl[])
                n229 = To Single Precision Float(number=w708) -> (single precision float=w706:sgl[])
                n230 = call "IMAQ GetPixelLine"("Line Coordinates"=w699, "Image"=w696) -> ("Pixels Line (Float)"=w701:sgl[])  [unwired: 2 in, 4 out]
                n231 = call "IMAQ GetPixelLine"("Line Coordinates"=w699, "Image"=w697) -> ("Pixels Line (Float)"=w700:sgl[])  [unwired: 2 in, 4 out]
                n232 = Divide(x=w707, y=w698) -> (x/y=w705:sgl[])
                n233 = Divide(x=w706, y=w698) -> (x/y=w704:sgl[])
                n234 = Add(x=w701, y=w705) -> (x+y=w702:sgl[])
                n235 = Add(x=w700, y=w704) -> (x+y=w703:sgl[])
              }
            }
            n236 = call "IMAQ SetPixelLine"("Pixels Line (Float)"=w670, "Line Coordinates"=w671, "Image"=w651) -> ()  [unwired: 7 in, 2 out]
            n237 = call "IMAQ SetPixelLine"("Pixels Line (Float)"=w669, "Line Coordinates"=w671, "Image"=w650) -> ()  [unwired: 7 in, 2 out]
            n238 = To Unsigned Word Integer(number=w669) -> (unsigned 16bit integer=w645:u16[])
            n239 = To Unsigned Word Integer(number=w670) -> (unsigned 16bit integer=w644:u16[])
            n240 = And(x=w658, y=w657) -> (x .and. y?=w659:bool)
            n241 = case shown="True" w659 {
              tunnel: w644 -> [_ w686]
              tunnel: w645 -> [_ w685]
              tunnel: w668 -> [_ w683]
              tunnel: w649 -> [_ w682]
              tunnel: w648 -> [_ w681]
              frame False {
              }
              frame True {
                w684 = FALSE ("prepend array or string size? (T)")
                n242 = Write to Binary File(file (use dialog)=w682, data=w686, 5:w684, 9:w683) -> ()  [unwired: 2 in, 3 out]
                n243 = Write to Binary File(file (use dialog)=w681, data=w685, 5:w684, 9:w683) -> ()  [unwired: 2 in, 3 out]
              }
            }
          }
        }
      }
    }
    frame 4, 20 {
      n244 = while {
        shift-right: [w749] -> _
        shift-left: 0 -> [w750]
        tunnel: w726 -> [w751]
        tunnel: w725 -> [w748]
        tunnel: w724 -> [w747]
        tunnel: w723 -> [w746]
        tunnel: w722 -> [w742]
        shift-right: [w739] -> _
        shift-left: u32 0 -> [w740]
        tunnel: w720 -> [w738]
        tunnel: w719 -> [w737]
        tunnel: w718 -> [w736]
        tunnel: w717 -> [w735]
        tunnel: w712 -> [w734]
        tunnel: w716 -> [w733]
        tunnel: w715 -> [w732]
        tunnel: w714 -> [w731]
        tunnel: w713 -> [w730]
        tunnel: w711 -> [w729]
        tunnel: [w728] -> w710
        stop <- w741 stop-if-true
        n245 = Get Queue Status(queue=w735) -> (queue out=w743:refnum<queue>, # elements in queue=w745:i32)  [unwired: 2 in, 6 out]
        n246 = Get Notifier Status(notifier=w742) -> (current notification=w741:bool)  [unwired: 1 in, 4 out]
        n247 = Greater Than 0?(x=w745) -> (x > 0?=w744:bool)
        n248 = case shown="True" w744 {
          tunnel: w751 -> [_ w781]
          tunnel: w750 -> [w754 w782]
          tunnel: [w754 w780] -> w749
          tunnel: w748 -> [_ w777]
          tunnel: w747 -> [_ w776]
          tunnel: w746 -> [_ w766]
          tunnel: w743 -> [_ w775]
          tunnel: w740 -> [w753 w772]
          tunnel: [w753 w771] -> w739
          tunnel: w738 -> [_ w770]
          tunnel: w737 -> [_ w769]
          tunnel: w736 -> [_ w764]
          tunnel: w734 -> [_ w762]
          tunnel: w733 -> [_ w761]
          tunnel: w732 -> [_ _]
          tunnel: w731 -> [_ _]
          tunnel: w730 -> [_ _]
          tunnel: w729 -> [w752 w757]
          tunnel: [w752 w756] -> w728
          frame False {
          }
          frame True {
            # "False: 1st frame in fram accum"
            # "True: Last Frame of frame accum"
            # "Current Line in Frame Accum"
            # "Current Line In Frame"
            n249 = Increment(x=w772) -> (x+1=w765:u32)
            n250 = Dequeue Element(queue=w775) -> (element=w787:u64[])  [unwired: 2 in, 3 out]
            n251 = Equal?(x=w765, y=w769) -> (x = y?=w774:bool)
            n252 = Greater?(x=w765, y=w770) -> (0:w767:bool)
            n253 = Greater?(x=w765, y=w764) -> (0:w763:bool)
            n254 = Split Number(x=w787) -> (lo(x)=w786:u32[])  [unwired: 1 out]
            n255 = Split Number(x=w786) -> (hi(x)=w760:u16[])  [unwired: 1 out]
            n256 = Select(t=u32 0, s=w774, f=w765) -> (s? t:f=w771:u32)
            n257 = Increment(x=w782) -> (x+1=w783:i32)
            n258 = Equal?(x=w781, y=w782) -> (x = y?=w758:bool)
            n259 = Select(t=0, s=w758, f=w783) -> (s? t:f=w780:i32)
            n260 = Build Array(0, w782, w781, w782) -> (w779:i32[])
            n261 = case shown="True" w763 {
              tunnel: w760 -> [w800 w809]
              tunnel: [w799 w806] -> w778
              tunnel: w779 -> [_ w804]
              tunnel: w776 -> [w798 w803]
              tunnel: w762 -> [w797 w802]
              tunnel: [w797 w802] -> w759
              frame False {
                n262 = To Single Precision Float(number=w800) -> (single precision float=w801:sgl[])
                n263 = Divide(x=w801, y=w798) -> (x/y=w799:sgl[])
              }
              frame True {
                n264 = To Single Precision Float(number=w809) -> (single precision float=w808:sgl[])
                n265 = call "IMAQ GetPixelLine"("Line Coordinates"=w804, "Image"=w802) -> ("Pixels Line (Float)"=w805:sgl[])  [unwired: 2 in, 4 out]
                n266 = Divide(x=w808, y=w803) -> (x/y=w807:sgl[])
                n267 = Add(x=w805, y=w807) -> (x+y=w806:sgl[])
              }
            }
            n268 = call "IMAQ SetPixelLine"("Pixels Line (Float)"=w778, "Line Coordinates"=w779, "Image"=w759) -> ()  [unwired: 7 in, 2 out]
            n269 = And(x=w767, y=w766) -> (x .and. y?=w768:bool)
            n270 = To Unsigned Word Integer(number=w778) -> (unsigned 16bit integer=w755:u16[])
            n271 = case shown="False" w758 {
              tunnel: w759 -> [_ w791]
              tunnel: w757 -> [w788 w790]
              tunnel: [w788 w789] -> w756
              frame False {
              }
              frame True {
                n272 = call "IMAQ ImageToArray"("Image"=w791) -> ("Image Pixels (Float)"=w792:sgl[][])  [unwired: 3 in, 4 out]
                n273 = Send Notification(notification=w792, notifier=w790) -> (notifier out=w789:refnum<notifier>)  [unwired: 1 in, 1 out]
              }
            }
            n274 = case shown="True" w768 {
              tunnel: w755 -> [_ w796]
              tunnel: w777 -> [_ w794]
              tunnel: w761 -> [_ w793]
              frame False {
              }
              frame True {
                n275 = Write to Binary File(file (use dialog)=w793, data=w796, 5:FALSE ("prepend array or string size? (T)"), 9:w794) -> ()  [unwired: 2 in, 3 out]
              }
            }
          }
        }
      }
      n276 = Release Notifier(notifier=w710) -> ()  [unwired: 2 in, 3 out]
    }
    frame 5 {
      n277 = while {
        shift-right: [w847] -> _
        shift-left: 0 -> [w848]
        tunnel: w825 -> [w849]
        tunnel: w824 -> [w846]
        tunnel: w823 -> [w845]
        tunnel: w822 -> [w844]
        tunnel: w821 -> [w840]
        shift-right: [w837] -> _
        shift-left: u32 0 -> [w838]
        tunnel: w819 -> [w836]
        tunnel: w818 -> [w835]
        tunnel: w817 -> [w834]
        tunnel: w816 -> [w833]
        tunnel: w811 -> [w832]
        tunnel: w810 -> [w831]
        tunnel: w815 -> [w830]
        tunnel: w814 -> [w829]
        tunnel: w813 -> [w828]
        tunnel: w812 -> [w827]
        stop <- w839 stop-if-true
        n278 = Get Queue Status(queue=w833) -> (queue out=w841:refnum<queue>, # elements in queue=w843:i32)  [unwired: 2 in, 6 out]
        n279 = Get Notifier Status(notifier=w840) -> (current notification=w839:bool)  [unwired: 1 in, 4 out]
        n280 = Greater Than 0?(x=w843) -> (x > 0?=w842:bool)
        n281 = case shown="True" w842 {
          tunnel: w849 -> [_ w880]
          tunnel: w848 -> [w851 w881]
          tunnel: [w851 w879] -> w847
          tunnel: w846 -> [_ w875]
          tunnel: w845 -> [_ w874]
          tunnel: w844 -> [_ w864]
          tunnel: w841 -> [_ w873]
          tunnel: w838 -> [w850 w870]
          tunnel: [w850 w869] -> w837
          tunnel: w836 -> [_ w868]
          tunnel: w835 -> [_ w867]
          tunnel: w834 -> [_ w862]
          tunnel: w832 -> [_ w860]
          tunnel: w831 -> [_ w859]
          tunnel: w830 -> [_ w855]
          tunnel: w829 -> [_ w854]
          tunnel: w828 -> [_ _]
          tunnel: w827 -> [_ _]
          frame False {
          }
          frame True {
            # "False: 1st frame in fram accum"
            # "True: Last Frame of frame accum"
            # "Current Line in Frame Accum"
            # "Current Line In Frame"
            n282 = Increment(x=w870) -> (x+1=w863:u32)
            n283 = Dequeue Element(queue=w873) -> (element=w888:u64[])  [unwired: 2 in, 3 out]
            n284 = Equal?(x=w863, y=w867) -> (x = y?=w872:bool)
            n285 = Greater?(x=w863, y=w868) -> (0:w865:bool)
            n286 = Greater?(x=w863, y=w862) -> (0:w861:bool)
            n287 = Split Number(x=w888) -> (hi(x)=w889:u32[], lo(x)=w887:u32[])
            n288 = Split Number(x=w889) -> (hi(x)=w856:u16[])  [unwired: 1 out]
            n289 = Split Number(x=w887) -> (hi(x)=w886:u16[])  [unwired: 1 out]
            n290 = Select(t=u32 0, s=w872, f=w863) -> (s? t:f=w869:u32)
            n291 = Increment(x=w881) -> (x+1=w883:i32)
            n292 = Equal?(x=w880, y=w881) -> (x = y?=w882:bool)
            n293 = Select(t=0, s=w882, f=w883) -> (s? t:f=w879:i32)
            n294 = Build Array(0, w881, w880, w881) -> (w878:i32[])
            n295 = case shown="False" w861 {
              tunnel: w856 -> [w903 w918]
              tunnel: w886 -> [w900 w917]
              tunnel: [w899 w913] -> w876
              tunnel: [w902 w912] -> w877
              tunnel: w878 -> [_ w909]
              tunnel: w874 -> [w898 w907]
              tunnel: w860 -> [w897 w905]
              tunnel: w859 -> [w896 w906]
              tunnel: [w896 w906] -> w857
              tunnel: [w897 w905] -> w858
              frame False {
                n296 = To Single Precision Float(number=w903) -> (single precision float=w904:sgl[])
                n297 = To Single Precision Float(number=w900) -> (single precision float=w901:sgl[])
                n298 = Divide(x=w904, y=w898) -> (x/y=w902:sgl[])
                n299 = Divide(x=w901, y=w898) -> (x/y=w899:sgl[])
              }
              frame True {
                n300 = To Single Precision Float(number=w918) -> (single precision float=w908:sgl[])
                n301 = To Single Precision Float(number=w917) -> (single precision float=w916:sgl[])
                n302 = call "IMAQ GetPixelLine"("Line Coordinates"=w909, "Image"=w905) -> ("Pixels Line (Float)"=w911:sgl[])  [unwired: 2 in, 4 out]
                n303 = call "IMAQ GetPixelLine"("Line Coordinates"=w909, "Image"=w906) -> ("Pixels Line (Float)"=w910:sgl[])  [unwired: 2 in, 4 out]
                n304 = Divide(x=w908, y=w907) -> (x/y=w915:sgl[])
                n305 = Divide(x=w916, y=w907) -> (x/y=w914:sgl[])
                n306 = Add(x=w911, y=w915) -> (x+y=w912:sgl[])
                n307 = Add(x=w910, y=w914) -> (x+y=w913:sgl[])
              }
            }
            n308 = call "IMAQ SetPixelLine"("Pixels Line (Float)"=w877, "Line Coordinates"=w878, "Image"=w858) -> ()  [unwired: 7 in, 2 out]
            n309 = call "IMAQ SetPixelLine"("Pixels Line (Float)"=w876, "Line Coordinates"=w878, "Image"=w857) -> ()  [unwired: 7 in, 2 out]
            n310 = To Unsigned Word Integer(number=w876) -> (unsigned 16bit integer=w852:u16[])
            n311 = And(x=w865, y=w864) -> (x .and. y?=w866:bool)
            n312 = To Unsigned Word Integer(number=w877) -> (unsigned 16bit integer=w853:u16[])
            n313 = case shown="True" w866 {
              tunnel: w853 -> [_ w895]
              tunnel: w852 -> [_ w894]
              tunnel: w875 -> [_ w892]
              tunnel: w855 -> [_ w891]
              tunnel: w854 -> [_ w890]
              frame False {
              }
              frame True {
                w893 = FALSE ("prepend array or string size? (T)")
                n314 = Write to Binary File(file (use dialog)=w891, data=w895, 5:w893, 9:w892) -> ()  [unwired: 2 in, 3 out]
                n315 = Write to Binary File(file (use dialog)=w890, data=w894, 5:w893, 9:w892) -> ()  [unwired: 2 in, 3 out]
              }
            }
          }
        }
      }
    }
    frame 6 {
      n316 = while {
        shift-right: [w956] -> _
        shift-left: 0 -> [w957]
        tunnel: w934 -> [w958]
        tunnel: w933 -> [w955]
        tunnel: w932 -> [w954]
        tunnel: w931 -> [w953]
        tunnel: w930 -> [w949]
        shift-right: [w946] -> _
        shift-left: u32 0 -> [w947]
        tunnel: w928 -> [w945]
        tunnel: w927 -> [w944]
        tunnel: w926 -> [w943]
        tunnel: w925 -> [w942]
        tunnel: w920 -> [w941]
        tunnel: w919 -> [w940]
        tunnel: w924 -> [w939]
        tunnel: w923 -> [w938]
        tunnel: w922 -> [w937]
        tunnel: w921 -> [w936]
        stop <- w948 stop-if-true
        n317 = Get Queue Status(queue=w942) -> (queue out=w950:refnum<queue>, # elements in queue=w952:i32)  [unwired: 2 in, 6 out]
        n318 = Get Notifier Status(notifier=w949) -> (current notification=w948:bool)  [unwired: 1 in, 4 out]
        n319 = Greater Than 0?(x=w952) -> (x > 0?=w951:bool)
        n320 = case shown="True" w951 {
          tunnel: w958 -> [_ w988]
          tunnel: w957 -> [w960 w989]
          tunnel: [w960 w987] -> w956
          tunnel: w955 -> [_ w984]
          tunnel: w954 -> [_ w983]
          tunnel: w953 -> [_ w973]
          tunnel: w950 -> [_ w982]
          tunnel: w947 -> [w959 w979]
          tunnel: [w959 w978] -> w946
          tunnel: w945 -> [_ w977]
          tunnel: w944 -> [_ w976]
          tunnel: w943 -> [_ w971]
          tunnel: w941 -> [_ w969]
          tunnel: w940 -> [_ w968]
          tunnel: w939 -> [_ w965]
          tunnel: w938 -> [_ w964]
          tunnel: w937 -> [_ _]
          tunnel: w936 -> [_ _]
          frame False {
          }
          frame True {
            # "False: 1st frame in fram accum"
            # "True: Last Frame of frame accum"
            # "Current Line in Frame Accum"
            # "Current Line In Frame"
            n321 = Increment(x=w979) -> (x+1=w972:u32)
            n322 = Dequeue Element(queue=w982) -> (element=w997:u64[])  [unwired: 2 in, 3 out]
            n323 = Equal?(x=w972, y=w976) -> (x = y?=w981:bool)
            n324 = Greater?(x=w972, y=w977) -> (0:w974:bool)
            n325 = Greater?(x=w972, y=w971) -> (0:w970:bool)
            n326 = Split Number(x=w997) -> (hi(x)=w998:u32[], lo(x)=w996:u32[])
            n327 = Split Number(x=w998) -> (lo(x)=w995:u16[])  [unwired: 1 out]
            n328 = Split Number(x=w996) -> (hi(x)=w994:u16[])  [unwired: 1 out]
            n329 = Select(t=u32 0, s=w981, f=w972) -> (s? t:f=w978:u32)
            n330 = Increment(x=w989) -> (x+1=w991:i32)
            n331 = Equal?(x=w988, y=w989) -> (x = y?=w990:bool)
            n332 = Select(t=0, s=w990, f=w991) -> (s? t:f=w987:i32)
            n333 = Build Array(0, w989, w988, w989) -> (w986:i32[])
            n334 = case shown="False" w970 {
              tunnel: w995 -> [w1011 w1027]
              tunnel: w994 -> [w1010 w1026]
              tunnel: [w1008 w1021] -> w962
              tunnel: [w1009 w1020] -> w985
              tunnel: w986 -> [_ w1017]
              tunnel: w983 -> [w1007 w1016]
              tunnel: w969 -> [w1006 w1014]
              tunnel: w968 -> [w1005 w1015]
              tunnel: [w1005 w1015] -> w966
              tunnel: [w1006 w1014] -> w967
              frame False {
                n335 = To Single Precision Float(number=w1011) -> (single precision float=w1013:sgl[])
                n336 = To Single Precision Float(number=w1010) -> (single precision float=w1012:sgl[])
                n337 = Divide(x=w1013, y=w1007) -> (x/y=w1009:sgl[])
                n338 = Divide(x=w1012, y=w1007) -> (x/y=w1008:sgl[])
              }
              frame True {
                n339 = To Single Precision Float(number=w1027) -> (single precision float=w1025:sgl[])
                n340 = To Single Precision Float(number=w1026) -> (single precision float=w1024:sgl[])
                n341 = call "IMAQ GetPixelLine"("Line Coordinates"=w1017, "Image"=w1014) -> ("Pixels Line (Float)"=w1019:sgl[])  [unwired: 2 in, 4 out]
                n342 = call "IMAQ GetPixelLine"("Line Coordinates"=w1017, "Image"=w1015) -> ("Pixels Line (Float)"=w1018:sgl[])  [unwired: 2 in, 4 out]
                n343 = Divide(x=w1025, y=w1016) -> (x/y=w1023:sgl[])
                n344 = Divide(x=w1024, y=w1016) -> (x/y=w1022:sgl[])
                n345 = Add(x=w1019, y=w1023) -> (x+y=w1020:sgl[])
                n346 = Add(x=w1018, y=w1022) -> (x+y=w1021:sgl[])
              }
            }
            n347 = call "IMAQ SetPixelLine"("Pixels Line (Float)"=w985, "Line Coordinates"=w986, "Image"=w967) -> ()  [unwired: 7 in, 2 out]
            n348 = call "IMAQ SetPixelLine"("Pixels Line (Float)"=w962, "Line Coordinates"=w986, "Image"=w966) -> ()  [unwired: 7 in, 2 out]
            n349 = To Unsigned Word Integer(number=w962) -> (unsigned 16bit integer=w961:u16[])
            n350 = And(x=w974, y=w973) -> (x .and. y?=w975:bool)
            n351 = To Unsigned Word Integer(number=w985) -> (unsigned 16bit integer=w963:u16[])
            n352 = case shown="True" w975 {
              tunnel: w963 -> [_ w1004]
              tunnel: w961 -> [_ w1003]
              tunnel: w984 -> [_ w1001]
              tunnel: w965 -> [_ w1000]
              tunnel: w964 -> [_ w999]
              frame False {
              }
              frame True {
                w1002 = FALSE ("prepend array or string size? (T)")
                n353 = Write to Binary File(file (use dialog)=w1000, data=w1004, 5:w1002, 9:w1001) -> ()  [unwired: 2 in, 3 out]
                n354 = Write to Binary File(file (use dialog)=w999, data=w1003, 5:w1002, 9:w1001) -> ()  [unwired: 2 in, 3 out]
              }
            }
          }
        }
      }
    }
    frame 7 {
      n355 = while {
        shift-right: [w1067] -> _
        shift-left: 0 -> [w1068]
        tunnel: w1044 -> [w1069]
        tunnel: w1043 -> [w1066]
        tunnel: w1042 -> [w1065]
        tunnel: w1041 -> [w1064]
        tunnel: w1040 -> [w1060]
        shift-right: [w1057] -> _
        shift-left: u32 0 -> [w1058]
        tunnel: w1038 -> [w1056]
        tunnel: w1037 -> [w1055]
        tunnel: w1036 -> [w1054]
        tunnel: w1035 -> [w1053]
        tunnel: w1030 -> [w1052]
        tunnel: w1029 -> [w1051]
        tunnel: w1028 -> [w1050]
        tunnel: w1034 -> [w1049]
        tunnel: w1033 -> [w1048]
        tunnel: w1032 -> [w1047]
        tunnel: w1031 -> [w1046]
        stop <- w1059 stop-if-true
        n356 = Get Queue Status(queue=w1053) -> (queue out=w1061:refnum<queue>, # elements in queue=w1063:i32)  [unwired: 2 in, 6 out]
        n357 = Get Notifier Status(notifier=w1060) -> (current notification=w1059:bool)  [unwired: 1 in, 4 out]
        n358 = Greater Than 0?(x=w1063) -> (x > 0?=w1062:bool)
        n359 = case shown="True" w1062 {
          tunnel: w1069 -> [_ w1105]
          tunnel: w1068 -> [w1071 w1106]
          tunnel: [w1071 w1104] -> w1067
          tunnel: w1066 -> [_ w1099]
          tunnel: w1065 -> [_ w1098]
          tunnel: w1064 -> [_ w1088]
          tunnel: w1061 -> [_ w1097]
          tunnel: w1058 -> [w1070 w1094]
          tunnel: [w1070 w1093] -> w1057
          tunnel: w1056 -> [_ w1092]
          tunnel: w1055 -> [_ w1091]
          tunnel: w1054 -> [_ w1086]
          tunnel: w1052 -> [_ w1084]
          tunnel: w1051 -> [_ w1083]
          tunnel: w1050 -> [_ w1082]
          tunnel: w1049 -> [_ w1077]
          tunnel: w1048 -> [_ w1076]
          tunnel: w1047 -> [_ w1075]
          tunnel: w1046 -> [_ _]
          frame False {
          }
          frame True {
            # "False: 1st frame in fram accum"
            # "True: Last Frame of frame accum"
            # "Current Line in Frame Accum"
            # "Current Line In Frame"
            n360 = Increment(x=w1094) -> (x+1=w1087:u32)
            n361 = Dequeue Element(queue=w1097) -> (element=w1114:u64[])  [unwired: 2 in, 3 out]
            n362 = Equal?(x=w1087, y=w1091) -> (x = y?=w1096:bool)
            n363 = Greater?(x=w1087, y=w1092) -> (0:w1089:bool)
            n364 = Greater?(x=w1087, y=w1086) -> (0:w1085:bool)
            n365 = Split Number(x=w1114) -> (hi(x)=w1115:u32[], lo(x)=w1113:u32[])
            n366 = Split Number(x=w1115) -> (hi(x)=w1078:u16[], lo(x)=w1112:u16[])
            n367 = Split Number(x=w1113) -> (hi(x)=w1111:u16[])  [unwired: 1 out]
            n368 = Select(t=u32 0, s=w1096, f=w1087) -> (s? t:f=w1093:u32)
            n369 = Increment(x=w1106) -> (x+1=w1108:i32)
            n370 = Equal?(x=w1105, y=w1106) -> (x = y?=w1107:bool)
            n371 = Select(t=0, s=w1107, f=w1108) -> (s? t:f=w1104:i32)
            n372 = Build Array(0, w1106, w1105, w1106) -> (w1103:i32[])
            n373 = case shown="False" w1085 {
              tunnel: w1078 -> [w1135 w1156]
              tunnel: w1112 -> [w1131 w1155]
              tunnel: w1111 -> [w1130 w1154]
              tunnel: [w1128 w1148] -> w1100
              tunnel: [w1129 w1147] -> w1101
              tunnel: [w1134 w1146] -> w1102
              tunnel: w1103 -> [_ w1142]
              tunnel: w1098 -> [w1127 w1140]
              tunnel: w1084 -> [w1126 w1137]
              tunnel: w1083 -> [w1125 w1138]
              tunnel: w1082 -> [w1124 w1139]
              tunnel: [w1124 w1139] -> w1079
              tunnel: [w1125 w1138] -> w1080
              tunnel: [w1126 w1137] -> w1081
              frame False {
                n374 = To Single Precision Float(number=w1135) -> (single precision float=w1136:sgl[])
                n375 = To Single Precision Float(number=w1131) -> (single precision float=w1133:sgl[])
                n376 = To Single Precision Float(number=w1130) -> (single precision float=w1132:sgl[])
                n377 = Divide(x=w1136, y=w1127) -> (x/y=w1134:sgl[])
                n378 = Divide(x=w1133, y=w1127) -> (x/y=w1129:sgl[])
                n379 = Divide(x=w1132, y=w1127) -> (x/y=w1128:sgl[])
              }
              frame True {
                n380 = To Single Precision Float(number=w1156) -> (single precision float=w1141:sgl[])
                n381 = To Single Precision Float(number=w1155) -> (single precision float=w1153:sgl[])
                n382 = To Single Precision Float(number=w1154) -> (single precision float=w1152:sgl[])
                n383 = call "IMAQ GetPixelLine"("Line Coordinates"=w1142, "Image"=w1137) -> ("Pixels Line (Float)"=w1145:sgl[])  [unwired: 2 in, 4 out]
                n384 = call "IMAQ GetPixelLine"("Line Coordinates"=w1142, "Image"=w1138) -> ("Pixels Line (Float)"=w1144:sgl[])  [unwired: 2 in, 4 out]
                n385 = call "IMAQ GetPixelLine"("Line Coordinates"=w1142, "Image"=w1139) -> ("Pixels Line (Float)"=w1143:sgl[])  [unwired: 2 in, 4 out]
                n386 = Divide(x=w1141, y=w1140) -> (x/y=w1151:sgl[])
                n387 = Divide(x=w1153, y=w1140) -> (x/y=w1150:sgl[])
                n388 = Divide(x=w1152, y=w1140) -> (x/y=w1149:sgl[])
                n389 = Add(x=w1145, y=w1151) -> (x+y=w1146:sgl[])
                n390 = Add(x=w1144, y=w1150) -> (x+y=w1147:sgl[])
                n391 = Add(x=w1143, y=w1149) -> (x+y=w1148:sgl[])
              }
            }
            n392 = call "IMAQ SetPixelLine"("Pixels Line (Float)"=w1102, "Line Coordinates"=w1103, "Image"=w1081) -> ()  [unwired: 7 in, 2 out]
            n393 = call "IMAQ SetPixelLine"("Pixels Line (Float)"=w1101, "Line Coordinates"=w1103, "Image"=w1080) -> ()  [unwired: 7 in, 2 out]
            n394 = call "IMAQ SetPixelLine"("Pixels Line (Float)"=w1100, "Line Coordinates"=w1103, "Image"=w1079) -> ()  [unwired: 7 in, 2 out]
            n395 = To Unsigned Word Integer(number=w1100) -> (unsigned 16bit integer=w1072:u16[])
            n396 = And(x=w1089, y=w1088) -> (x .and. y?=w1090:bool)
            n397 = To Unsigned Word Integer(number=w1102) -> (unsigned 16bit integer=w1074:u16[])
            n398 = To Unsigned Word Integer(number=w1101) -> (unsigned 16bit integer=w1073:u16[])
            n399 = case shown="True" w1090 {
              tunnel: w1074 -> [_ w1123]
              tunnel: w1073 -> [_ w1122]
              tunnel: w1072 -> [_ w1121]
              tunnel: w1099 -> [_ w1119]
              tunnel: w1077 -> [_ w1118]
              tunnel: w1076 -> [_ w1117]
              tunnel: w1075 -> [_ w1116]
              frame False {
              }
              frame True {
                w1120 = FALSE ("prepend array or string size? (T)")
                n400 = Write to Binary File(file (use dialog)=w1118, data=w1123, 5:w1120, 9:w1119) -> ()  [unwired: 2 in, 3 out]
                n401 = Write to Binary File(file (use dialog)=w1117, data=w1122, 5:w1120, 9:w1119) -> ()  [unwired: 2 in, 3 out]
                n402 = Write to Binary File(file (use dialog)=w1116, data=w1121, 5:w1120, 9:w1119) -> ()  [unwired: 2 in, 3 out]
              }
            }
          }
        }
      }
    }
    frame 8, 24 {
      n403 = while {
        shift-right: [w1196] -> _
        shift-left: 0 -> [w1197]
        tunnel: w1173 -> [w1198]
        tunnel: w1172 -> [w1195]
        tunnel: w1171 -> [w1194]
        tunnel: w1170 -> [w1193]
        tunnel: w1169 -> [w1189]
        shift-right: [w1186] -> _
        shift-left: u32 0 -> [w1187]
        tunnel: w1167 -> [w1185]
        tunnel: w1166 -> [w1184]
        tunnel: w1165 -> [w1183]
        tunnel: w1164 -> [w1182]
        tunnel: w1159 -> [w1181]
        tunnel: w1163 -> [w1180]
        tunnel: w1162 -> [w1179]
        tunnel: w1161 -> [w1178]
        tunnel: w1160 -> [w1177]
        tunnel: w1158 -> [w1176]
        tunnel: [w1175] -> w1157
        stop <- w1188 stop-if-true
        n404 = Get Queue Status(queue=w1182) -> (queue out=w1190:refnum<queue>, # elements in queue=w1192:i32)  [unwired: 2 in, 6 out]
        n405 = Get Notifier Status(notifier=w1189) -> (current notification=w1188:bool)  [unwired: 1 in, 4 out]
        n406 = Greater Than 0?(x=w1192) -> (x > 0?=w1191:bool)
        n407 = case shown="True" w1191 {
          tunnel: w1198 -> [_ w1227]
          tunnel: w1197 -> [w1201 w1228]
          tunnel: [w1201 w1226] -> w1196
          tunnel: w1195 -> [_ w1223]
          tunnel: w1194 -> [_ w1222]
          tunnel: w1193 -> [_ w1212]
          tunnel: w1190 -> [_ w1221]
          tunnel: w1187 -> [w1200 w1218]
          tunnel: [w1200 w1217] -> w1186
          tunnel: w1185 -> [_ w1216]
          tunnel: w1184 -> [_ w1215]
          tunnel: w1183 -> [_ w1210]
          tunnel: w1181 -> [_ w1208]
          tunnel: w1180 -> [_ w1207]
          tunnel: w1179 -> [_ _]
          tunnel: w1178 -> [_ _]
          tunnel: w1177 -> [_ _]
          tunnel: w1176 -> [w1199 w1204]
          tunnel: [w1199 w1203] -> w1175
          frame False {
          }
          frame True {
            # "False: 1st frame in fram accum"
            # "True: Last Frame of frame accum"
            # "Current Line in Frame Accum"
            # "Current Line In Frame"
            n408 = Increment(x=w1218) -> (x+1=w1211:u32)
            n409 = Dequeue Element(queue=w1221) -> (element=w1234:u64[])  [unwired: 2 in, 3 out]
            n410 = Equal?(x=w1211, y=w1215) -> (x = y?=w1220:bool)
            n411 = Greater?(x=w1211, y=w1216) -> (0:w1213:bool)
            n412 = Greater?(x=w1211, y=w1210) -> (0:w1209:bool)
            n413 = Split Number(x=w1234) -> (lo(x)=w1233:u32[])  [unwired: 1 out]
            n414 = Split Number(x=w1233) -> (lo(x)=w1232:u16[])  [unwired: 1 out]
            n415 = Select(t=u32 0, s=w1220, f=w1211) -> (s? t:f=w1217:u32)
            n416 = Increment(x=w1228) -> (x+1=w1229:i32)
            n417 = Equal?(x=w1227, y=w1228) -> (x = y?=w1205:bool)
            n418 = Select(t=0, s=w1205, f=w1229) -> (s? t:f=w1226:i32)
            n419 = Build Array(0, w1228, w1227, w1228) -> (w1225:i32[])
            n420 = case shown="False" w1209 {
              tunnel: w1232 -> [w1247 w1256]
              tunnel: [w1246 w1253] -> w1224
              tunnel: w1225 -> [_ w1251]
              tunnel: w1222 -> [w1245 w1250]
              tunnel: w1208 -> [w1244 w1249]
              tunnel: [w1244 w1249] -> w1206
              frame False {
                n421 = To Single Precision Float(number=w1247) -> (single precision float=w1248:sgl[])
                n422 = Divide(x=w1248, y=w1245) -> (x/y=w1246:sgl[])
              }
              frame True {
                n423 = To Single Precision Float(number=w1256) -> (single precision float=w1255:sgl[])
                n424 = call "IMAQ GetPixelLine"("Line Coordinates"=w1251, "Image"=w1249) -> ("Pixels Line (Float)"=w1252:sgl[])  [unwired: 2 in, 4 out]
                n425 = Divide(x=w1255, y=w1250) -> (x/y=w1254:sgl[])
                n426 = Add(x=w1252, y=w1254) -> (x+y=w1253:sgl[])
              }
            }
            n427 = call "IMAQ SetPixelLine"("Pixels Line (Float)"=w1224, "Line Coordinates"=w1225, "Image"=w1206) -> ()  [unwired: 7 in, 2 out]
            n428 = To Unsigned Word Integer(number=w1224) -> (unsigned 16bit integer=w1202:u16[])
            n429 = And(x=w1213, y=w1212) -> (x .and. y?=w1214:bool)
            n430 = case shown="False" w1205 {
              tunnel: w1206 -> [_ w1238]
              tunnel: w1204 -> [w1235 w1237]
              tunnel: [w1235 w1236] -> w1203
              frame False {
              }
              frame True {
                n431 = call "IMAQ ImageToArray"("Image"=w1238) -> ("Image Pixels (Float)"=w1239:sgl[][])  [unwired: 3 in, 4 out]
                n432 = Send Notification(notification=w1239, notifier=w1237) -> (notifier out=w1236:refnum<notifier>)  [unwired: 1 in, 1 out]
              }
            }
            n433 = case shown="True" w1214 {
              tunnel: w1202 -> [_ w1243]
              tunnel: w1223 -> [_ w1241]
              tunnel: w1207 -> [_ w1240]
              frame False {
              }
              frame True {
                n434 = Write to Binary File(file (use dialog)=w1240, data=w1243, 5:FALSE ("prepend array or string size? (T)"), 9:w1241) -> ()  [unwired: 2 in, 3 out]
              }
            }
          }
        }
      }
      n435 = Release Notifier(notifier=w1157) -> ()  [unwired: 2 in, 3 out]
    }
    frame 9 {
      n436 = while {
        shift-right: [w1294] -> _
        shift-left: 0 -> [w1295]
        tunnel: w1272 -> [w1296]
        tunnel: w1271 -> [w1293]
        tunnel: w1270 -> [w1292]
        tunnel: w1269 -> [w1291]
        tunnel: w1268 -> [w1287]
        shift-right: [w1284] -> _
        shift-left: u32 0 -> [w1285]
        tunnel: w1266 -> [w1283]
        tunnel: w1265 -> [w1282]
        tunnel: w1264 -> [w1281]
        tunnel: w1263 -> [w1280]
        tunnel: w1258 -> [w1279]
        tunnel: w1257 -> [w1278]
        tunnel: w1262 -> [w1277]
        tunnel: w1261 -> [w1276]
        tunnel: w1260 -> [w1275]
        tunnel: w1259 -> [w1274]
        stop <- w1286 stop-if-true
        n437 = Get Queue Status(queue=w1280) -> (queue out=w1288:refnum<queue>, # elements in queue=w1290:i32)  [unwired: 2 in, 6 out]
        n438 = Get Notifier Status(notifier=w1287) -> (current notification=w1286:bool)  [unwired: 1 in, 4 out]
        n439 = Greater Than 0?(x=w1290) -> (x > 0?=w1289:bool)
        n440 = case shown="True" w1289 {
          tunnel: w1296 -> [_ w1327]
          tunnel: w1295 -> [w1298 w1328]
          tunnel: [w1298 w1326] -> w1294
          tunnel: w1293 -> [_ w1324]
          tunnel: w1292 -> [_ w1323]
          tunnel: w1291 -> [_ w1313]
          tunnel: w1288 -> [_ w1322]
          tunnel: w1285 -> [w1297 w1319]
          tunnel: [w1297 w1318] -> w1284
          tunnel: w1283 -> [_ w1317]
          tunnel: w1282 -> [_ w1316]
          tunnel: w1281 -> [_ w1311]
          tunnel: w1279 -> [_ w1309]
          tunnel: w1278 -> [_ w1308]
          tunnel: w1277 -> [_ w1304]
          tunnel: w1276 -> [_ w1303]
          tunnel: w1275 -> [_ _]
          tunnel: w1274 -> [_ _]
          frame False {
          }
          frame True {
            # "False: 1st frame in fram accum"
            # "True: Last Frame of frame accum"
            # "Current Line in Frame Accum"
            # "Current Line In Frame"
            n441 = Increment(x=w1319) -> (x+1=w1312:u32)
            n442 = Dequeue Element(queue=w1322) -> (element=w1335:u64[])  [unwired: 2 in, 3 out]
            n443 = Equal?(x=w1312, y=w1316) -> (x = y?=w1321:bool)
            n444 = Greater?(x=w1312, y=w1317) -> (0:w1314:bool)
            n445 = Greater?(x=w1312, y=w1311) -> (0:w1310:bool)
            n446 = Split Number(x=w1335) -> (hi(x)=w1336:u32[], lo(x)=w1334:u32[])
            n447 = Split Number(x=w1336) -> (hi(x)=w1305:u16[])  [unwired: 1 out]
            n448 = Split Number(x=w1334) -> (lo(x)=w1333:u16[])  [unwired: 1 out]
            n449 = Select(t=u32 0, s=w1321, f=w1312) -> (s? t:f=w1318:u32)
            n450 = Increment(x=w1328) -> (x+1=w1330:i32)
            n451 = Equal?(x=w1327, y=w1328) -> (x = y?=w1329:bool)
            n452 = Select(t=0, s=w1329, f=w1330) -> (s? t:f=w1326:i32)
            n453 = Build Array(0, w1328, w1327, w1328) -> (w1325:i32[])
            n454 = case shown="True" w1310 {
              tunnel: w1305 -> [w1350 w1365]
              tunnel: w1333 -> [w1347 w1364]
              tunnel: [w1349 w1360] -> w1302
              tunnel: [w1346 w1359] -> w1301
              tunnel: w1325 -> [_ w1356]
              tunnel: w1323 -> [w1345 w1354]
              tunnel: w1309 -> [w1344 w1353]
              tunnel: w1308 -> [w1343 w1352]
              tunnel: [w1344 w1353] -> w1307
              tunnel: [w1343 w1352] -> w1306
              frame False {
                n455 = To Single Precision Float(number=w1350) -> (single precision float=w1351:sgl[])
                n456 = To Single Precision Float(number=w1347) -> (single precision float=w1348:sgl[])
                n457 = Divide(x=w1351, y=w1345) -> (x/y=w1349:sgl[])
                n458 = Divide(x=w1348, y=w1345) -> (x/y=w1346:sgl[])
              }
              frame True {
                n459 = To Single Precision Float(number=w1365) -> (single precision float=w1355:sgl[])
                n460 = To Single Precision Float(number=w1364) -> (single precision float=w1363:sgl[])
                n461 = call "IMAQ GetPixelLine"("Line Coordinates"=w1356, "Image"=w1353) -> ("Pixels Line (Float)"=w1358:sgl[])  [unwired: 2 in, 4 out]
                n462 = call "IMAQ GetPixelLine"("Line Coordinates"=w1356, "Image"=w1352) -> ("Pixels Line (Float)"=w1357:sgl[])  [unwired: 2 in, 4 out]
                n463 = Divide(x=w1355, y=w1354) -> (x/y=w1362:sgl[])
                n464 = Divide(x=w1363, y=w1354) -> (x/y=w1361:sgl[])
                n465 = Add(x=w1358, y=w1362) -> (x+y=w1360:sgl[])
                n466 = Add(x=w1357, y=w1361) -> (x+y=w1359:sgl[])
              }
            }
            n467 = call "IMAQ SetPixelLine"("Pixels Line (Float)"=w1302, "Line Coordinates"=w1325, "Image"=w1307) -> ()  [unwired: 7 in, 2 out]
            n468 = call "IMAQ SetPixelLine"("Pixels Line (Float)"=w1301, "Line Coordinates"=w1325, "Image"=w1306) -> ()  [unwired: 7 in, 2 out]
            n469 = To Unsigned Word Integer(number=w1301) -> (unsigned 16bit integer=w1300:u16[])
            n470 = And(x=w1314, y=w1313) -> (x .and. y?=w1315:bool)
            n471 = To Unsigned Word Integer(number=w1302) -> (unsigned 16bit integer=w1299:u16[])
            n472 = case shown="True" w1315 {
              tunnel: w1299 -> [_ w1342]
              tunnel: w1300 -> [_ w1341]
              tunnel: w1324 -> [_ w1339]
              tunnel: w1304 -> [_ w1338]
              tunnel: w1303 -> [_ w1337]
              frame False {
              }
              frame True {
                w1340 = FALSE ("prepend array or string size? (T)")
                n473 = Write to Binary File(file (use dialog)=w1338, data=w1342, 5:w1340, 9:w1339) -> ()  [unwired: 2 in, 3 out]
                n474 = Write to Binary File(file (use dialog)=w1337, data=w1341, 5:w1340, 9:w1339) -> ()  [unwired: 2 in, 3 out]
              }
            }
          }
        }
      }
    }
    frame 10 {
      n475 = while {
        shift-right: [w1403] -> _
        shift-left: 0 -> [w1404]
        tunnel: w1381 -> [w1405]
        tunnel: w1380 -> [w1402]
        tunnel: w1379 -> [w1401]
        tunnel: w1378 -> [w1400]
        tunnel: w1377 -> [w1396]
        shift-right: [w1393] -> _
        shift-left: u32 0 -> [w1394]
        tunnel: w1375 -> [w1392]
        tunnel: w1374 -> [w1391]
        tunnel: w1373 -> [w1390]
        tunnel: w1372 -> [w1389]
        tunnel: w1367 -> [w1388]
        tunnel: w1366 -> [w1387]
        tunnel: w1371 -> [w1386]
        tunnel: w1370 -> [w1385]
        tunnel: w1369 -> [w1384]
        tunnel: w1368 -> [w1383]
        stop <- w1395 stop-if-true
        n476 = Get Queue Status(queue=w1389) -> (queue out=w1397:refnum<queue>, # elements in queue=w1399:i32)  [unwired: 2 in, 6 out]
        n477 = Get Notifier Status(notifier=w1396) -> (current notification=w1395:bool)  [unwired: 1 in, 4 out]
        n478 = Greater Than 0?(x=w1399) -> (x > 0?=w1398:bool)
        n479 = case shown="True" w1398 {
          tunnel: w1405 -> [_ w1435]
          tunnel: w1404 -> [w1407 w1436]
          tunnel: [w1407 w1434] -> w1403
          tunnel: w1402 -> [_ w1432]
          tunnel: w1401 -> [_ w1431]
          tunnel: w1400 -> [_ w1421]
          tunnel: w1397 -> [_ w1430]
          tunnel: w1394 -> [w1406 w1427]
          tunnel: [w1406 w1426] -> w1393
          tunnel: w1392 -> [_ w1425]
          tunnel: w1391 -> [_ w1424]
          tunnel: w1390 -> [_ w1419]
          tunnel: w1388 -> [_ w1417]
          tunnel: w1387 -> [_ w1416]
          tunnel: w1386 -> [_ w1413]
          tunnel: w1385 -> [_ w1412]
          tunnel: w1384 -> [_ _]
          tunnel: w1383 -> [_ _]
          frame False {
          }
          frame True {
            # "False: 1st frame in fram accum"
            # "True: Last Frame of frame accum"
            # "Current Line in Frame Accum"
            # "Current Line In Frame"
            n480 = Increment(x=w1427) -> (x+1=w1420:u32)
            n481 = Dequeue Element(queue=w1430) -> (element=w1444:u64[])  [unwired: 2 in, 3 out]
            n482 = Equal?(x=w1420, y=w1424) -> (x = y?=w1429:bool)
            n483 = Greater?(x=w1420, y=w1425) -> (0:w1422:bool)
            n484 = Greater?(x=w1420, y=w1419) -> (0:w1418:bool)
            n485 = Split Number(x=w1444) -> (hi(x)=w1445:u32[], lo(x)=w1443:u32[])
            n486 = Split Number(x=w1445) -> (lo(x)=w1442:u16[])  [unwired: 1 out]
            n487 = Split Number(x=w1443) -> (lo(x)=w1441:u16[])  [unwired: 1 out]
            n488 = Select(t=u32 0, s=w1429, f=w1420) -> (s? t:f=w1426:u32)
            n489 = Increment(x=w1436) -> (x+1=w1438:i32)
            n490 = Equal?(x=w1435, y=w1436) -> (x = y?=w1437:bool)
            n491 = Select(t=0, s=w1437, f=w1438) -> (s? t:f=w1434:i32)
            n492 = Build Array(0, w1436, w1435, w1436) -> (w1433:i32[])
            n493 = case shown="True" w1418 {
              tunnel: w1442 -> [w1458 w1474]
              tunnel: w1441 -> [w1457 w1473]
              tunnel: [w1456 w1468] -> w1409
              tunnel: [w1455 w1467] -> w1411
              tunnel: w1433 -> [_ w1464]
              tunnel: w1431 -> [w1454 w1463]
              tunnel: w1417 -> [w1453 w1462]
              tunnel: w1416 -> [w1452 w1461]
              tunnel: [w1453 w1462] -> w1415
              tunnel: [w1452 w1461] -> w1414
              frame False {
                n494 = To Single Precision Float(number=w1458) -> (single precision float=w1460:sgl[])
                n495 = To Single Precision Float(number=w1457) -> (single precision float=w1459:sgl[])
                n496 = Divide(x=w1460, y=w1454) -> (x/y=w1456:sgl[])
                n497 = Divide(x=w1459, y=w1454) -> (x/y=w1455:sgl[])
              }
              frame True {
                n498 = To Single Precision Float(number=w1474) -> (single precision float=w1472:sgl[])
                n499 = To Single Precision Float(number=w1473) -> (single precision float=w1471:sgl[])
                n500 = call "IMAQ GetPixelLine"("Line Coordinates"=w1464, "Image"=w1462) -> ("Pixels Line (Float)"=w1466:sgl[])  [unwired: 2 in, 4 out]
                n501 = call "IMAQ GetPixelLine"("Line Coordinates"=w1464, "Image"=w1461) -> ("Pixels Line (Float)"=w1465:sgl[])  [unwired: 2 in, 4 out]
                n502 = Divide(x=w1472, y=w1463) -> (x/y=w1470:sgl[])
                n503 = Divide(x=w1471, y=w1463) -> (x/y=w1469:sgl[])
                n504 = Add(x=w1466, y=w1470) -> (x+y=w1468:sgl[])
                n505 = Add(x=w1465, y=w1469) -> (x+y=w1467:sgl[])
              }
            }
            n506 = call "IMAQ SetPixelLine"("Pixels Line (Float)"=w1409, "Line Coordinates"=w1433, "Image"=w1415) -> ()  [unwired: 7 in, 2 out]
            n507 = call "IMAQ SetPixelLine"("Pixels Line (Float)"=w1411, "Line Coordinates"=w1433, "Image"=w1414) -> ()  [unwired: 7 in, 2 out]
            n508 = To Unsigned Word Integer(number=w1411) -> (unsigned 16bit integer=w1410:u16[])
            n509 = And(x=w1422, y=w1421) -> (x .and. y?=w1423:bool)
            n510 = To Unsigned Word Integer(number=w1409) -> (unsigned 16bit integer=w1408:u16[])
            n511 = case shown="True" w1423 {
              tunnel: w1408 -> [_ w1451]
              tunnel: w1410 -> [_ w1450]
              tunnel: w1432 -> [_ w1448]
              tunnel: w1413 -> [_ w1447]
              tunnel: w1412 -> [_ w1446]
              frame False {
              }
              frame True {
                w1449 = FALSE ("prepend array or string size? (T)")
                n512 = Write to Binary File(file (use dialog)=w1447, data=w1451, 5:w1449, 9:w1448) -> ()  [unwired: 2 in, 3 out]
                n513 = Write to Binary File(file (use dialog)=w1446, data=w1450, 5:w1449, 9:w1448) -> ()  [unwired: 2 in, 3 out]
              }
            }
          }
        }
      }
    }
    frame 11 {
      n514 = while {
        shift-right: [w1514] -> _
        shift-left: 0 -> [w1515]
        tunnel: w1491 -> [w1516]
        tunnel: w1490 -> [w1513]
        tunnel: w1489 -> [w1512]
        tunnel: w1488 -> [w1511]
        tunnel: w1487 -> [w1507]
        shift-right: [w1504] -> _
        shift-left: u32 0 -> [w1505]
        tunnel: w1485 -> [w1503]
        tunnel: w1484 -> [w1502]
        tunnel: w1483 -> [w1501]
        tunnel: w1482 -> [w1500]
        tunnel: w1477 -> [w1499]
        tunnel: w1476 -> [w1498]
        tunnel: w1475 -> [w1497]
        tunnel: w1481 -> [w1496]
        tunnel: w1480 -> [w1495]
        tunnel: w1479 -> [w1494]
        tunnel: w1478 -> [w1493]
        stop <- w1506 stop-if-true
        n515 = Get Queue Status(queue=w1500) -> (queue out=w1508:refnum<queue>, # elements in queue=w1510:i32)  [unwired: 2 in, 6 out]
        n516 = Get Notifier Status(notifier=w1507) -> (current notification=w1506:bool)  [unwired: 1 in, 4 out]
        n517 = Greater Than 0?(x=w1510) -> (x > 0?=w1509:bool)
        n518 = case shown="True" w1509 {
          tunnel: w1516 -> [_ w1552]
          tunnel: w1515 -> [w1518 w1553]
          tunnel: [w1518 w1551] -> w1514
          tunnel: w1513 -> [_ w1546]
          tunnel: w1512 -> [_ w1545]
          tunnel: w1511 -> [_ w1535]
          tunnel: w1508 -> [_ w1544]
          tunnel: w1505 -> [w1517 w1541]
          tunnel: [w1517 w1540] -> w1504
          tunnel: w1503 -> [_ w1539]
          tunnel: w1502 -> [_ w1538]
          tunnel: w1501 -> [_ w1533]
          tunnel: w1499 -> [_ w1531]
          tunnel: w1498 -> [_ w1530]
          tunnel: w1497 -> [_ w1529]
          tunnel: w1496 -> [_ w1524]
          tunnel: w1495 -> [_ w1523]
          tunnel: w1494 -> [_ w1522]
          tunnel: w1493 -> [_ _]
          frame False {
          }
          frame True {
            # "False: 1st frame in fram accum"
            # "True: Last Frame of frame accum"
            # "Current Line in Frame Accum"
            # "Current Line In Frame"
            n519 = Increment(x=w1541) -> (x+1=w1534:u32)
            n520 = Dequeue Element(queue=w1544) -> (element=w1561:u64[])  [unwired: 2 in, 3 out]
            n521 = Equal?(x=w1534, y=w1538) -> (x = y?=w1543:bool)
            n522 = Greater?(x=w1534, y=w1539) -> (0:w1536:bool)
            n523 = Greater?(x=w1534, y=w1533) -> (0:w1532:bool)
            n524 = Split Number(x=w1561) -> (hi(x)=w1562:u32[], lo(x)=w1560:u32[])
            n525 = Split Number(x=w1562) -> (hi(x)=w1525:u16[], lo(x)=w1559:u16[])
            n526 = Split Number(x=w1560) -> (lo(x)=w1558:u16[])  [unwired: 1 out]
            n527 = Select(t=u32 0, s=w1543, f=w1534) -> (s? t:f=w1540:u32)
            n528 = Increment(x=w1553) -> (x+1=w1555:i32)
            n529 = Equal?(x=w1552, y=w1553) -> (x = y?=w1554:bool)
            n530 = Select(t=0, s=w1554, f=w1555) -> (s? t:f=w1551:i32)
            n531 = Build Array(0, w1553, w1552, w1553) -> (w1550:i32[])
            n532 = case shown="False" w1532 {
              tunnel: w1525 -> [w1582 w1603]
              tunnel: w1559 -> [w1578 w1602]
              tunnel: w1558 -> [w1577 w1601]
              tunnel: [w1576 w1595] -> w1548
              tunnel: [w1581 w1594] -> w1549
              tunnel: [w1575 w1593] -> w1547
              tunnel: w1550 -> [_ w1589]
              tunnel: w1545 -> [w1574 w1587]
              tunnel: w1531 -> [w1573 w1585]
              tunnel: w1530 -> [w1572 w1586]
              tunnel: w1529 -> [w1571 w1584]
              tunnel: [w1572 w1586] -> w1527
              tunnel: [w1573 w1585] -> w1528
              tunnel: [w1571 w1584] -> w1526
              frame False {
                n533 = To Single Precision Float(number=w1582) -> (single precision float=w1583:sgl[])
                n534 = To Single Precision Float(number=w1578) -> (single precision float=w1580:sgl[])
                n535 = To Single Precision Float(number=w1577) -> (single precision float=w1579:sgl[])
                n536 = Divide(x=w1583, y=w1574) -> (x/y=w1581:sgl[])
                n537 = Divide(x=w1580, y=w1574) -> (x/y=w1576:sgl[])
                n538 = Divide(x=w1579, y=w1574) -> (x/y=w1575:sgl[])
              }
              frame True {
                n539 = To Single Precision Float(number=w1603) -> (single precision float=w1588:sgl[])
                n540 = To Single Precision Float(number=w1602) -> (single precision float=w1600:sgl[])
                n541 = To Single Precision Float(number=w1601) -> (single precision float=w1599:sgl[])
                n542 = call "IMAQ GetPixelLine"("Line Coordinates"=w1589, "Image"=w1585) -> ("Pixels Line (Float)"=w1592:sgl[])  [unwired: 2 in, 4 out]
                n543 = call "IMAQ GetPixelLine"("Line Coordinates"=w1589, "Image"=w1586) -> ("Pixels Line (Float)"=w1591:sgl[])  [unwired: 2 in, 4 out]
                n544 = call "IMAQ GetPixelLine"("Line Coordinates"=w1589, "Image"=w1584) -> ("Pixels Line (Float)"=w1590:sgl[])  [unwired: 2 in, 4 out]
                n545 = Divide(x=w1588, y=w1587) -> (x/y=w1598:sgl[])
                n546 = Divide(x=w1600, y=w1587) -> (x/y=w1597:sgl[])
                n547 = Divide(x=w1599, y=w1587) -> (x/y=w1596:sgl[])
                n548 = Add(x=w1592, y=w1598) -> (x+y=w1594:sgl[])
                n549 = Add(x=w1591, y=w1597) -> (x+y=w1595:sgl[])
                n550 = Add(x=w1590, y=w1596) -> (x+y=w1593:sgl[])
              }
            }
            n551 = call "IMAQ SetPixelLine"("Pixels Line (Float)"=w1549, "Line Coordinates"=w1550, "Image"=w1528) -> ()  [unwired: 7 in, 2 out]
            n552 = call "IMAQ SetPixelLine"("Pixels Line (Float)"=w1548, "Line Coordinates"=w1550, "Image"=w1527) -> ()  [unwired: 7 in, 2 out]
            n553 = call "IMAQ SetPixelLine"("Pixels Line (Float)"=w1547, "Line Coordinates"=w1550, "Image"=w1526) -> ()  [unwired: 7 in, 2 out]
            n554 = To Unsigned Word Integer(number=w1548) -> (unsigned 16bit integer=w1520:u16[])
            n555 = To Unsigned Word Integer(number=w1547) -> (unsigned 16bit integer=w1519:u16[])
            n556 = And(x=w1536, y=w1535) -> (x .and. y?=w1537:bool)
            n557 = To Unsigned Word Integer(number=w1549) -> (unsigned 16bit integer=w1521:u16[])
            n558 = case shown="True" w1537 {
              tunnel: w1521 -> [_ w1570]
              tunnel: w1520 -> [_ w1569]
              tunnel: w1519 -> [_ w1568]
              tunnel: w1546 -> [_ w1566]
              tunnel: w1524 -> [_ w1565]
              tunnel: w1523 -> [_ w1564]
              tunnel: w1522 -> [_ w1563]
              frame False {
              }
              frame True {
                w1567 = FALSE ("prepend array or string size? (T)")
                n559 = Write to Binary File(file (use dialog)=w1565, data=w1570, 5:w1567, 9:w1566) -> ()  [unwired: 2 in, 3 out]
                n560 = Write to Binary File(file (use dialog)=w1564, data=w1569, 5:w1567, 9:w1566) -> ()  [unwired: 2 in, 3 out]
                n561 = Write to Binary File(file (use dialog)=w1563, data=w1568, 5:w1567, 9:w1566) -> ()  [unwired: 2 in, 3 out]
              }
            }
          }
        }
      }
    }
    frame 12 {
      n562 = while {
        shift-right: [w1641] -> _
        shift-left: 0 -> [w1642]
        tunnel: w1619 -> [w1643]
        tunnel: w1618 -> [w1640]
        tunnel: w1617 -> [w1639]
        tunnel: w1616 -> [w1638]
        tunnel: w1615 -> [w1634]
        shift-right: [w1631] -> _
        shift-left: u32 0 -> [w1632]
        tunnel: w1613 -> [w1630]
        tunnel: w1612 -> [w1629]
        tunnel: w1611 -> [w1628]
        tunnel: w1610 -> [w1627]
        tunnel: w1605 -> [w1626]
        tunnel: w1604 -> [w1625]
        tunnel: w1609 -> [w1624]
        tunnel: w1608 -> [w1623]
        tunnel: w1607 -> [w1622]
        tunnel: w1606 -> [w1621]
        stop <- w1633 stop-if-true
        n563 = Get Queue Status(queue=w1627) -> (queue out=w1635:refnum<queue>, # elements in queue=w1637:i32)  [unwired: 2 in, 6 out]
        n564 = Get Notifier Status(notifier=w1634) -> (current notification=w1633:bool)  [unwired: 1 in, 4 out]
        n565 = Greater Than 0?(x=w1637) -> (x > 0?=w1636:bool)
        n566 = case shown="True" w1636 {
          tunnel: w1643 -> [_ w1674]
          tunnel: w1642 -> [w1645 w1675]
          tunnel: [w1645 w1673] -> w1641
          tunnel: w1640 -> [_ w1669]
          tunnel: w1639 -> [_ w1668]
          tunnel: w1638 -> [_ w1658]
          tunnel: w1635 -> [_ w1667]
          tunnel: w1632 -> [w1644 w1664]
          tunnel: [w1644 w1663] -> w1631
          tunnel: w1630 -> [_ w1662]
          tunnel: w1629 -> [_ w1661]
          tunnel: w1628 -> [_ w1656]
          tunnel: w1626 -> [_ w1654]
          tunnel: w1625 -> [_ w1653]
          tunnel: w1624 -> [_ w1650]
          tunnel: w1623 -> [_ w1649]
          tunnel: w1622 -> [_ _]
          tunnel: w1621 -> [_ _]
          frame False {
          }
          frame True {
            # "False: 1st frame in fram accum"
            # "True: Last Frame of frame accum"
            # "Current Line in Frame Accum"
            # "Current Line In Frame"
            n567 = Increment(x=w1664) -> (x+1=w1657:u32)
            n568 = Dequeue Element(queue=w1667) -> (element=w1682:u64[])  [unwired: 2 in, 3 out]
            n569 = Equal?(x=w1657, y=w1661) -> (x = y?=w1666:bool)
            n570 = Greater?(x=w1657, y=w1662) -> (0:w1659:bool)
            n571 = Greater?(x=w1657, y=w1656) -> (0:w1655:bool)
            n572 = Split Number(x=w1682) -> (lo(x)=w1681:u32[])  [unwired: 1 out]
            n573 = Split Number(x=w1681) -> (hi(x)=w1648:u16[], lo(x)=w1680:u16[])
            n574 = Select(t=u32 0, s=w1666, f=w1657) -> (s? t:f=w1663:u32)
            n575 = Increment(x=w1675) -> (x+1=w1677:i32)
            n576 = Equal?(x=w1674, y=w1675) -> (x = y?=w1676:bool)
            n577 = Select(t=0, s=w1676, f=w1677) -> (s? t:f=w1673:i32)
            n578 = Build Array(0, w1675, w1674, w1675) -> (w1672:i32[])
            n579 = case shown="True" w1655 {
              tunnel: w1648 -> [w1696 w1711]
              tunnel: w1680 -> [w1693 w1710]
              tunnel: [w1695 w1706] -> w1671
              tunnel: [w1692 w1705] -> w1670
              tunnel: w1672 -> [_ w1702]
              tunnel: w1668 -> [w1691 w1700]
              tunnel: w1654 -> [w1690 w1699]
              tunnel: w1653 -> [w1689 w1698]
              tunnel: [w1690 w1699] -> w1652
              tunnel: [w1689 w1698] -> w1651
              frame False {
                n580 = To Single Precision Float(number=w1696) -> (single precision float=w1697:sgl[])
                n581 = To Single Precision Float(number=w1693) -> (single precision float=w1694:sgl[])
                n582 = Divide(x=w1697, y=w1691) -> (x/y=w1695:sgl[])
                n583 = Divide(x=w1694, y=w1691) -> (x/y=w1692:sgl[])
              }
              frame True {
                n584 = To Single Precision Float(number=w1711) -> (single precision float=w1701:sgl[])
                n585 = To Single Precision Float(number=w1710) -> (single precision float=w1709:sgl[])
                n586 = call "IMAQ GetPixelLine"("Line Coordinates"=w1702, "Image"=w1699) -> ("Pixels Line (Float)"=w1704:sgl[])  [unwired: 2 in, 4 out]
                n587 = call "IMAQ GetPixelLine"("Line Coordinates"=w1702, "Image"=w1698) -> ("Pixels Line (Float)"=w1703:sgl[])  [unwired: 2 in, 4 out]
                n588 = Divide(x=w1701, y=w1700) -> (x/y=w1708:sgl[])
                n589 = Divide(x=w1709, y=w1700) -> (x/y=w1707:sgl[])
                n590 = Add(x=w1704, y=w1708) -> (x+y=w1706:sgl[])
                n591 = Add(x=w1703, y=w1707) -> (x+y=w1705:sgl[])
              }
            }
            n592 = call "IMAQ SetPixelLine"("Pixels Line (Float)"=w1671, "Line Coordinates"=w1672, "Image"=w1652) -> ()  [unwired: 7 in, 2 out]
            n593 = call "IMAQ SetPixelLine"("Pixels Line (Float)"=w1670, "Line Coordinates"=w1672, "Image"=w1651) -> ()  [unwired: 7 in, 2 out]
            n594 = To Unsigned Word Integer(number=w1670) -> (unsigned 16bit integer=w1646:u16[])
            n595 = And(x=w1659, y=w1658) -> (x .and. y?=w1660:bool)
            n596 = To Unsigned Word Integer(number=w1671) -> (unsigned 16bit integer=w1647:u16[])
            n597 = case shown="True" w1660 {
              tunnel: w1647 -> [_ w1688]
              tunnel: w1646 -> [_ w1687]
              tunnel: w1669 -> [_ w1685]
              tunnel: w1650 -> [_ w1684]
              tunnel: w1649 -> [_ w1683]
              frame False {
              }
              frame True {
                w1686 = FALSE ("prepend array or string size? (T)")
                n598 = Write to Binary File(file (use dialog)=w1684, data=w1688, 5:w1686, 9:w1685) -> ()  [unwired: 2 in, 3 out]
                n599 = Write to Binary File(file (use dialog)=w1683, data=w1687, 5:w1686, 9:w1685) -> ()  [unwired: 2 in, 3 out]
              }
            }
          }
        }
      }
    }
    frame 13 {
      n600 = while {
        shift-right: [w1751] -> _
        shift-left: 0 -> [w1752]
        tunnel: w1728 -> [w1753]
        tunnel: w1727 -> [w1750]
        tunnel: w1726 -> [w1749]
        tunnel: w1725 -> [w1748]
        tunnel: w1724 -> [w1744]
        shift-right: [w1741] -> _
        shift-left: u32 0 -> [w1742]
        tunnel: w1722 -> [w1740]
        tunnel: w1721 -> [w1739]
        tunnel: w1720 -> [w1738]
        tunnel: w1719 -> [w1737]
        tunnel: w1714 -> [w1736]
        tunnel: w1713 -> [w1735]
        tunnel: w1712 -> [w1734]
        tunnel: w1718 -> [w1733]
        tunnel: w1717 -> [w1732]
        tunnel: w1716 -> [w1731]
        tunnel: w1715 -> [w1730]
        stop <- w1743 stop-if-true
        n601 = Get Queue Status(queue=w1737) -> (queue out=w1745:refnum<queue>, # elements in queue=w1747:i32)  [unwired: 2 in, 6 out]
        n602 = Get Notifier Status(notifier=w1744) -> (current notification=w1743:bool)  [unwired: 1 in, 4 out]
        n603 = Greater Than 0?(x=w1747) -> (x > 0?=w1746:bool)
        n604 = case shown="True" w1746 {
          tunnel: w1753 -> [_ w1789]
          tunnel: w1752 -> [w1755 w1790]
          tunnel: [w1755 w1788] -> w1751
          tunnel: w1750 -> [_ w1783]
          tunnel: w1749 -> [_ w1782]
          tunnel: w1748 -> [_ w1772]
          tunnel: w1745 -> [_ w1781]
          tunnel: w1742 -> [w1754 w1778]
          tunnel: [w1754 w1777] -> w1741
          tunnel: w1740 -> [_ w1776]
          tunnel: w1739 -> [_ w1775]
          tunnel: w1738 -> [_ w1770]
          tunnel: w1736 -> [_ w1768]
          tunnel: w1735 -> [_ w1767]
          tunnel: w1734 -> [_ w1766]
          tunnel: w1733 -> [_ w1761]
          tunnel: w1732 -> [_ w1760]
          tunnel: w1731 -> [_ w1759]
          tunnel: w1730 -> [_ _]
          frame False {
          }
          frame True {
            # "False: 1st frame in fram accum"
            # "True: Last Frame of frame accum"
            # "Current Line in Frame Accum"
            # "Current Line In Frame"
            n605 = Increment(x=w1778) -> (x+1=w1771:u32)
            n606 = Dequeue Element(queue=w1781) -> (element=w1798:u64[])  [unwired: 2 in, 3 out]
            n607 = Equal?(x=w1771, y=w1775) -> (x = y?=w1780:bool)
            n608 = Greater?(x=w1771, y=w1776) -> (0:w1773:bool)
            n609 = Greater?(x=w1771, y=w1770) -> (0:w1769:bool)
            n610 = Split Number(x=w1798) -> (hi(x)=w1799:u32[], lo(x)=w1797:u32[])
            n611 = Split Number(x=w1799) -> (hi(x)=w1762:u16[])  [unwired: 1 out]
            n612 = Split Number(x=w1797) -> (hi(x)=w1796:u16[], lo(x)=w1795:u16[])
            n613 = Select(t=u32 0, s=w1780, f=w1771) -> (s? t:f=w1777:u32)
            n614 = Increment(x=w1790) -> (x+1=w1792:i32)
            n615 = Equal?(x=w1789, y=w1790) -> (x = y?=w1791:bool)
            n616 = Select(t=0, s=w1791, f=w1792) -> (s? t:f=w1788:i32)
            n617 = Build Array(0, w1790, w1789, w1790) -> (w1787:i32[])
            n618 = case shown="True" w1769 {
              tunnel: w1762 -> [w1819 w1840]
              tunnel: w1796 -> [w1815 w1839]
              tunnel: w1795 -> [w1814 w1838]
              tunnel: [w1813 w1832] -> w1785
              tunnel: [w1818 w1831] -> w1786
              tunnel: [w1812 w1830] -> w1784
              tunnel: w1787 -> [_ w1826]
              tunnel: w1782 -> [w1811 w1824]
              tunnel: w1768 -> [w1810 w1822]
              tunnel: w1767 -> [w1809 w1823]
              tunnel: w1766 -> [w1808 w1821]
              tunnel: [w1809 w1823] -> w1764
              tunnel: [w1810 w1822] -> w1765
              tunnel: [w1808 w1821] -> w1763
              frame False {
                n619 = To Single Precision Float(number=w1819) -> (single precision float=w1820:sgl[])
                n620 = To Single Precision Float(number=w1815) -> (single precision float=w1817:sgl[])
                n621 = To Single Precision Float(number=w1814) -> (single precision float=w1816:sgl[])
                n622 = Divide(x=w1820, y=w1811) -> (x/y=w1818:sgl[])
                n623 = Divide(x=w1817, y=w1811) -> (x/y=w1813:sgl[])
                n624 = Divide(x=w1816, y=w1811) -> (x/y=w1812:sgl[])
              }
              frame True {
                n625 = To Single Precision Float(number=w1840) -> (single precision float=w1825:sgl[])
                n626 = To Single Precision Float(number=w1839) -> (single precision float=w1837:sgl[])
                n627 = To Single Precision Float(number=w1838) -> (single precision float=w1836:sgl[])
                n628 = call "IMAQ GetPixelLine"("Line Coordinates"=w1826, "Image"=w1822) -> ("Pixels Line (Float)"=w1829:sgl[])  [unwired: 2 in, 4 out]
                n629 = call "IMAQ GetPixelLine"("Line Coordinates"=w1826, "Image"=w1823) -> ("Pixels Line (Float)"=w1828:sgl[])  [unwired: 2 in, 4 out]
                n630 = call "IMAQ GetPixelLine"("Line Coordinates"=w1826, "Image"=w1821) -> ("Pixels Line (Float)"=w1827:sgl[])  [unwired: 2 in, 4 out]
                n631 = Divide(x=w1825, y=w1824) -> (x/y=w1835:sgl[])
                n632 = Divide(x=w1837, y=w1824) -> (x/y=w1834:sgl[])
                n633 = Divide(x=w1836, y=w1824) -> (x/y=w1833:sgl[])
                n634 = Add(x=w1829, y=w1835) -> (x+y=w1831:sgl[])
                n635 = Add(x=w1828, y=w1834) -> (x+y=w1832:sgl[])
                n636 = Add(x=w1827, y=w1833) -> (x+y=w1830:sgl[])
              }
            }
            n637 = call "IMAQ SetPixelLine"("Pixels Line (Float)"=w1786, "Line Coordinates"=w1787, "Image"=w1765) -> ()  [unwired: 7 in, 2 out]
            n638 = call "IMAQ SetPixelLine"("Pixels Line (Float)"=w1785, "Line Coordinates"=w1787, "Image"=w1764) -> ()  [unwired: 7 in, 2 out]
            n639 = call "IMAQ SetPixelLine"("Pixels Line (Float)"=w1784, "Line Coordinates"=w1787, "Image"=w1763) -> ()  [unwired: 7 in, 2 out]
            n640 = To Unsigned Word Integer(number=w1784) -> (unsigned 16bit integer=w1756:u16[])
            n641 = To Unsigned Word Integer(number=w1785) -> (unsigned 16bit integer=w1757:u16[])
            n642 = And(x=w1773, y=w1772) -> (x .and. y?=w1774:bool)
            n643 = To Unsigned Word Integer(number=w1786) -> (unsigned 16bit integer=w1758:u16[])
            n644 = case shown="True" w1774 {
              tunnel: w1758 -> [_ w1807]
              tunnel: w1757 -> [_ w1806]
              tunnel: w1756 -> [_ w1805]
              tunnel: w1783 -> [_ w1803]
              tunnel: w1761 -> [_ w1802]
              tunnel: w1760 -> [_ w1801]
              tunnel: w1759 -> [_ w1800]
              frame False {
              }
              frame True {
                w1804 = FALSE ("prepend array or string size? (T)")
                n645 = Write to Binary File(file (use dialog)=w1802, data=w1807, 5:w1804, 9:w1803) -> ()  [unwired: 2 in, 3 out]
                n646 = Write to Binary File(file (use dialog)=w1801, data=w1806, 5:w1804, 9:w1803) -> ()  [unwired: 2 in, 3 out]
                n647 = Write to Binary File(file (use dialog)=w1800, data=w1805, 5:w1804, 9:w1803) -> ()  [unwired: 2 in, 3 out]
              }
            }
          }
        }
      }
    }
    frame 14 {
      n648 = while {
        shift-right: [w1880] -> _
        shift-left: 0 -> [w1881]
        tunnel: w1857 -> [w1882]
        tunnel: w1856 -> [w1879]
        tunnel: w1855 -> [w1878]
        tunnel: w1854 -> [w1877]
        tunnel: w1853 -> [w1873]
        shift-right: [w1870] -> _
        shift-left: u32 0 -> [w1871]
        tunnel: w1851 -> [w1869]
        tunnel: w1850 -> [w1868]
        tunnel: w1849 -> [w1867]
        tunnel: w1848 -> [w1866]
        tunnel: w1843 -> [w1861]
        tunnel: w1842 -> [w1860]
        tunnel: w1841 -> [w1859]
        tunnel: w1847 -> [w1865]
        tunnel: w1846 -> [w1864]
        tunnel: w1845 -> [w1863]
        tunnel: w1844 -> [w1862]
        stop <- w1872 stop-if-true
        n649 = Get Queue Status(queue=w1866) -> (queue out=w1874:refnum<queue>, # elements in queue=w1876:i32)  [unwired: 2 in, 6 out]
        n650 = Get Notifier Status(notifier=w1873) -> (current notification=w1872:bool)  [unwired: 1 in, 4 out]
        n651 = Greater Than 0?(x=w1876) -> (x > 0?=w1875:bool)
        n652 = case shown="True" w1875 {
          tunnel: w1882 -> [_ w1917]
          tunnel: w1881 -> [w1884 w1918]
          tunnel: [w1884 w1916] -> w1880
          tunnel: w1879 -> [_ w1911]
          tunnel: w1878 -> [_ w1910]
          tunnel: w1877 -> [_ w1900]
          tunnel: w1874 -> [_ w1909]
          tunnel: w1871 -> [w1883 w1906]
          tunnel: [w1883 w1905] -> w1870
          tunnel: w1869 -> [_ w1904]
          tunnel: w1868 -> [_ w1903]
          tunnel: w1867 -> [_ w1898]
          tunnel: w1861 -> [_ w1896]
          tunnel: w1860 -> [_ w1895]
          tunnel: w1859 -> [_ w1894]
          tunnel: w1865 -> [_ w1890]
          tunnel: w1864 -> [_ w1889]
          tunnel: w1863 -> [_ w1888]
          tunnel: w1862 -> [_ _]
          frame False {
          }
          frame True {
            # "False: 1st frame in fram accum"
            # "True: Last Frame of frame accum"
            # "Current Line in Frame Accum"
            # "Current Line In Frame"
            n653 = Increment(x=w1906) -> (x+1=w1899:u32)
            n654 = Dequeue Element(queue=w1909) -> (element=w1927:u64[])  [unwired: 2 in, 3 out]
            n655 = Equal?(x=w1899, y=w1903) -> (x = y?=w1908:bool)
            n656 = Greater?(x=w1899, y=w1904) -> (0:w1901:bool)
            n657 = Greater?(x=w1899, y=w1898) -> (0:w1897:bool)
            n658 = Split Number(x=w1927) -> (hi(x)=w1928:u32[], lo(x)=w1926:u32[])
            n659 = Split Number(x=w1928) -> (lo(x)=w1925:u16[])  [unwired: 1 out]
            n660 = Split Number(x=w1926) -> (hi(x)=w1924:u16[], lo(x)=w1923:u16[])
            n661 = Select(t=u32 0, s=w1908, f=w1899) -> (s? t:f=w1905:u32)
            n662 = Increment(x=w1918) -> (x+1=w1920:i32)
            n663 = Equal?(x=w1917, y=w1918) -> (x = y?=w1919:bool)
            n664 = Select(t=0, s=w1919, f=w1920) -> (s? t:f=w1916:i32)
            n665 = Build Array(0, w1918, w1917, w1918) -> (w1915:i32[])
            n666 = case shown="True" w1897 {
              tunnel: w1925 -> [w1946 w1969]
              tunnel: w1924 -> [w1945 w1968]
              tunnel: w1923 -> [w1944 w1967]
              tunnel: [w1942 w1960] -> w1913
              tunnel: [w1943 w1959] -> w1914
              tunnel: [w1941 w1958] -> w1912
              tunnel: w1915 -> [_ w1954]
              tunnel: w1910 -> [w1940 w1953]
              tunnel: w1896 -> [w1939 w1951]
              tunnel: w1895 -> [w1938 w1952]
              tunnel: w1894 -> [w1937 w1950]
              tunnel: [w1938 w1952] -> w1892
              tunnel: [w1939 w1951] -> w1893
              tunnel: [w1937 w1950] -> w1891
              frame False {
                n667 = To Single Precision Float(number=w1946) -> (single precision float=w1949:sgl[])
                n668 = To Single Precision Float(number=w1945) -> (single precision float=w1948:sgl[])
                n669 = To Single Precision Float(number=w1944) -> (single precision float=w1947:sgl[])
                n670 = Divide(x=w1949, y=w1940) -> (x/y=w1943:sgl[])
                n671 = Divide(x=w1948, y=w1940) -> (x/y=w1942:sgl[])
                n672 = Divide(x=w1947, y=w1940) -> (x/y=w1941:sgl[])
              }
              frame True {
                n673 = To Single Precision Float(number=w1969) -> (single precision float=w1966:sgl[])
                n674 = To Single Precision Float(number=w1968) -> (single precision float=w1965:sgl[])
                n675 = To Single Precision Float(number=w1967) -> (single precision float=w1964:sgl[])
                n676 = call "IMAQ GetPixelLine"("Line Coordinates"=w1954, "Image"=w1951) -> ("Pixels Line (Float)"=w1957:sgl[])  [unwired: 2 in, 4 out]
                n677 = call "IMAQ GetPixelLine"("Line Coordinates"=w1954, "Image"=w1952) -> ("Pixels Line (Float)"=w1956:sgl[])  [unwired: 2 in, 4 out]
                n678 = call "IMAQ GetPixelLine"("Line Coordinates"=w1954, "Image"=w1950) -> ("Pixels Line (Float)"=w1955:sgl[])  [unwired: 2 in, 4 out]
                n679 = Divide(x=w1966, y=w1953) -> (x/y=w1963:sgl[])
                n680 = Divide(x=w1965, y=w1953) -> (x/y=w1962:sgl[])
                n681 = Divide(x=w1964, y=w1953) -> (x/y=w1961:sgl[])
                n682 = Add(x=w1957, y=w1963) -> (x+y=w1959:sgl[])
                n683 = Add(x=w1956, y=w1962) -> (x+y=w1960:sgl[])
                n684 = Add(x=w1955, y=w1961) -> (x+y=w1958:sgl[])
              }
            }
            n685 = call "IMAQ SetPixelLine"("Pixels Line (Float)"=w1914, "Line Coordinates"=w1915, "Image"=w1893) -> ()  [unwired: 7 in, 2 out]
            n686 = call "IMAQ SetPixelLine"("Pixels Line (Float)"=w1913, "Line Coordinates"=w1915, "Image"=w1892) -> ()  [unwired: 7 in, 2 out]
            n687 = call "IMAQ SetPixelLine"("Pixels Line (Float)"=w1912, "Line Coordinates"=w1915, "Image"=w1891) -> ()  [unwired: 7 in, 2 out]
            n688 = To Unsigned Word Integer(number=w1912) -> (unsigned 16bit integer=w1885:u16[])
            n689 = To Unsigned Word Integer(number=w1913) -> (unsigned 16bit integer=w1886:u16[])
            n690 = To Unsigned Word Integer(number=w1914) -> (unsigned 16bit integer=w1887:u16[])
            n691 = And(x=w1901, y=w1900) -> (x .and. y?=w1902:bool)
            n692 = case shown="True" w1902 {
              tunnel: w1887 -> [_ w1936]
              tunnel: w1886 -> [_ w1935]
              tunnel: w1885 -> [_ w1934]
              tunnel: w1911 -> [_ w1932]
              tunnel: w1890 -> [_ w1931]
              tunnel: w1889 -> [_ w1930]
              tunnel: w1888 -> [_ w1929]
              frame False {
              }
              frame True {
                w1933 = FALSE ("prepend array or string size? (T)")
                n693 = Write to Binary File(file (use dialog)=w1931, data=w1936, 5:w1933, 9:w1932) -> ()  [unwired: 2 in, 3 out]
                n694 = Write to Binary File(file (use dialog)=w1930, data=w1935, 5:w1933, 9:w1932) -> ()  [unwired: 2 in, 3 out]
                n695 = Write to Binary File(file (use dialog)=w1929, data=w1934, 5:w1933, 9:w1932) -> ()  [unwired: 2 in, 3 out]
              }
            }
          }
        }
      }
    }
    frame 15 {
      n696 = while {
        shift-right: [w2011] -> _
        shift-left: 0 -> [w2012]
        tunnel: w1987 -> [w2013]
        tunnel: w1986 -> [w2010]
        tunnel: w1985 -> [w2009]
        tunnel: w1984 -> [w2008]
        tunnel: w1983 -> [w2004]
        shift-right: [w2001] -> _
        shift-left: u32 0 -> [w2002]
        tunnel: w1981 -> [w2000]
        tunnel: w1980 -> [w1999]
        tunnel: w1979 -> [w1998]
        tunnel: w1978 -> [w1997]
        tunnel: w1973 -> [w1996]
        tunnel: w1972 -> [w1995]
        tunnel: w1971 -> [w1994]
        tunnel: w1970 -> [w1993]
        tunnel: w1977 -> [w1992]
        tunnel: w1976 -> [w1991]
        tunnel: w1975 -> [w1990]
        tunnel: w1974 -> [w1989]
        stop <- w2003 stop-if-true
        n697 = Get Queue Status(queue=w1997) -> (queue out=w2005:refnum<queue>, # elements in queue=w2007:i32)  [unwired: 2 in, 6 out]
        n698 = Get Notifier Status(notifier=w2004) -> (current notification=w2003:bool)  [unwired: 1 in, 4 out]
        n699 = Greater Than 0?(x=w2007) -> (x > 0?=w2006:bool)
        n700 = case shown="True" w2006 {
          tunnel: w2013 -> [_ w2054]
          tunnel: w2012 -> [w2015 w2055]
          tunnel: [w2015 w2053] -> w2011
          tunnel: w2010 -> [_ w2047]
          tunnel: w2009 -> [_ w2046]
          tunnel: w2008 -> [_ w2036]
          tunnel: w2005 -> [_ w2045]
          tunnel: w2002 -> [w2014 w2042]
          tunnel: [w2014 w2041] -> w2001
          tunnel: w2000 -> [_ w2040]
          tunnel: w1999 -> [_ w2039]
          tunnel: w1998 -> [_ w2034]
          tunnel: w1996 -> [_ w2032]
          tunnel: w1995 -> [_ w2031]
          tunnel: w1994 -> [_ w2030]
          tunnel: w1993 -> [_ w2029]
          tunnel: w1992 -> [_ w2023]
          tunnel: w1991 -> [_ w2022]
          tunnel: w1990 -> [_ w2021]
          tunnel: w1989 -> [_ w2020]
          frame False {
          }
          frame True {
            # "False: 1st frame in fram accum"
            # "True: Last Frame of frame accum"
            # "Current Line in Frame Accum"
            # "Current Line In Frame"
            n701 = Increment(x=w2042) -> (x+1=w2035:u32)
            n702 = Dequeue Element(queue=w2045) -> (element=w2064:u64[])  [unwired: 2 in, 3 out]
            n703 = Equal?(x=w2035, y=w2039) -> (x = y?=w2044:bool)
            n704 = Greater?(x=w2035, y=w2040) -> (0:w2037:bool)
            n705 = Greater?(x=w2035, y=w2034) -> (0:w2033:bool)
            n706 = Split Number(x=w2064) -> (hi(x)=w2065:u32[], lo(x)=w2063:u32[])
            n707 = Split Number(x=w2065) -> (hi(x)=w2024:u16[], lo(x)=w2062:u16[])
            n708 = Split Number(x=w2063) -> (hi(x)=w2061:u16[], lo(x)=w2060:u16[])
            n709 = Select(t=u32 0, s=w2044, f=w2035) -> (s? t:f=w2041:u32)
            n710 = Increment(x=w2055) -> (x+1=w2057:i32)
            n711 = Equal?(x=w2054, y=w2055) -> (x = y?=w2056:bool)
            n712 = Select(t=0, s=w2056, f=w2057) -> (s? t:f=w2053:i32)
            n713 = Build Array(0, w2055, w2054, w2055) -> (w2052:i32[])
            n714 = case shown="True" w2033 {
              tunnel: w2024 -> [w2091 w2118]
              tunnel: w2062 -> [w2086 w2117]
              tunnel: w2061 -> [w2085 w2116]
              tunnel: w2060 -> [w2084 w2115]
              tunnel: [w2082 w2107] -> w2049
              tunnel: [w2083 w2106] -> w2050
              tunnel: [w2090 w2105] -> w2051
              tunnel: [w2081 w2104] -> w2048
              tunnel: w2052 -> [_ w2099]
              tunnel: w2046 -> [w2080 w2097]
              tunnel: w2032 -> [w2079 w2094]
              tunnel: w2031 -> [w2078 w2095]
              tunnel: w2030 -> [w2077 w2096]
              tunnel: w2029 -> [w2076 w2093]
              tunnel: [w2077 w2096] -> w2026
              tunnel: [w2078 w2095] -> w2027
              tunnel: [w2079 w2094] -> w2028
              tunnel: [w2076 w2093] -> w2025
              frame False {
                n715 = To Single Precision Float(number=w2091) -> (single precision float=w2092:sgl[])
                n716 = To Single Precision Float(number=w2086) -> (single precision float=w2089:sgl[])
                n717 = To Single Precision Float(number=w2085) -> (single precision float=w2088:sgl[])
                n718 = To Single Precision Float(number=w2084) -> (single precision float=w2087:sgl[])
                n719 = Divide(x=w2092, y=w2080) -> (x/y=w2090:sgl[])
                n720 = Divide(x=w2089, y=w2080) -> (x/y=w2083:sgl[])
                n721 = Divide(x=w2088, y=w2080) -> (x/y=w2082:sgl[])
                n722 = Divide(x=w2087, y=w2080) -> (x/y=w2081:sgl[])
              }
              frame True {
                n723 = To Single Precision Float(number=w2118) -> (single precision float=w2098:sgl[])
                n724 = To Single Precision Float(number=w2117) -> (single precision float=w2114:sgl[])
                n725 = To Single Precision Float(number=w2116) -> (single precision float=w2113:sgl[])
                n726 = To Single Precision Float(number=w2115) -> (single precision float=w2112:sgl[])
                n727 = call "IMAQ GetPixelLine"("Line Coordinates"=w2099, "Image"=w2094) -> ("Pixels Line (Float)"=w2103:sgl[])  [unwired: 2 in, 4 out]
                n728 = call "IMAQ GetPixelLine"("Line Coordinates"=w2099, "Image"=w2095) -> ("Pixels Line (Float)"=w2102:sgl[])  [unwired: 2 in, 4 out]
                n729 = call "IMAQ GetPixelLine"("Line Coordinates"=w2099, "Image"=w2096) -> ("Pixels Line (Float)"=w2101:sgl[])  [unwired: 2 in, 4 out]
                n730 = call "IMAQ GetPixelLine"("Line Coordinates"=w2099, "Image"=w2093) -> ("Pixels Line (Float)"=w2100:sgl[])  [unwired: 2 in, 4 out]
                n731 = Divide(x=w2098, y=w2097) -> (x/y=w2111:sgl[])
                n732 = Divide(x=w2114, y=w2097) -> (x/y=w2110:sgl[])
                n733 = Divide(x=w2113, y=w2097) -> (x/y=w2109:sgl[])
                n734 = Divide(x=w2112, y=w2097) -> (x/y=w2108:sgl[])
                n735 = Add(x=w2103, y=w2111) -> (x+y=w2105:sgl[])
                n736 = Add(x=w2102, y=w2110) -> (x+y=w2106:sgl[])
                n737 = Add(x=w2101, y=w2109) -> (x+y=w2107:sgl[])
                n738 = Add(x=w2100, y=w2108) -> (x+y=w2104:sgl[])
              }
            }
            n739 = call "IMAQ SetPixelLine"("Pixels Line (Float)"=w2051, "Line Coordinates"=w2052, "Image"=w2028) -> ()  [unwired: 7 in, 2 out]
            n740 = call "IMAQ SetPixelLine"("Pixels Line (Float)"=w2050, "Line Coordinates"=w2052, "Image"=w2027) -> ()  [unwired: 7 in, 2 out]
            n741 = call "IMAQ SetPixelLine"("Pixels Line (Float)"=w2049, "Line Coordinates"=w2052, "Image"=w2026) -> ()  [unwired: 7 in, 2 out]
            n742 = call "IMAQ SetPixelLine"("Pixels Line (Float)"=w2048, "Line Coordinates"=w2052, "Image"=w2025) -> ()  [unwired: 7 in, 2 out]
            n743 = To Unsigned Word Integer(number=w2048) -> (unsigned 16bit integer=w2016:u16[])
            n744 = To Unsigned Word Integer(number=w2049) -> (unsigned 16bit integer=w2017:u16[])
            n745 = And(x=w2037, y=w2036) -> (x .and. y?=w2038:bool)
            n746 = To Unsigned Word Integer(number=w2051) -> (unsigned 16bit integer=w2019:u16[])
            n747 = To Unsigned Word Integer(number=w2050) -> (unsigned 16bit integer=w2018:u16[])
            n748 = case shown="True" w2038 {
              tunnel: w2019 -> [_ w2075]
              tunnel: w2018 -> [_ w2074]
              tunnel: w2017 -> [_ w2073]
              tunnel: w2016 -> [_ w2072]
              tunnel: w2047 -> [_ w2070]
              tunnel: w2023 -> [_ w2069]
              tunnel: w2022 -> [_ w2068]
              tunnel: w2021 -> [_ w2067]
              tunnel: w2020 -> [_ w2066]
              frame False {
              }
              frame True {
                w2071 = FALSE ("prepend array or string size? (T)")
                n749 = Write to Binary File(file (use dialog)=w2069, data=w2075, 5:w2071, 9:w2070) -> ()  [unwired: 2 in, 3 out]
                n750 = Write to Binary File(file (use dialog)=w2068, data=w2074, 5:w2071, 9:w2070) -> ()  [unwired: 2 in, 3 out]
                n751 = Write to Binary File(file (use dialog)=w2067, data=w2073, 5:w2071, 9:w2070) -> ()  [unwired: 2 in, 3 out]
                n752 = Write to Binary File(file (use dialog)=w2066, data=w2072, 5:w2071, 9:w2070) -> ()  [unwired: 2 in, 3 out]
              }
            }
          }
        }
      }
    }
    frame 19 {
      n753 = while {
        shift-right: [w2154] -> _
        shift-left: 0 -> [w2155]
        tunnel: w2133 -> [w2156]
        tunnel: w2132 -> [w2153]
        tunnel: w2131 -> [w2152]
        tunnel: w2130 -> [w2151]
        tunnel: w2129 -> [w2147]
        shift-right: [w2144] -> _
        shift-left: u32 0 -> [w2145]
        tunnel: w2127 -> [w2143]
        tunnel: w2126 -> [w2142]
        tunnel: w2125 -> [w2141]
        tunnel: w2124 -> [w2140]
        tunnel: w2119 -> [w2139]
        tunnel: w2123 -> [w2138]
        tunnel: w2122 -> [w2137]
        tunnel: w2121 -> [w2136]
        tunnel: w2120 -> [w2135]
        stop <- w2146 stop-if-true
        n754 = Get Queue Status(queue=w2140) -> (queue out=w2148:refnum<queue>, # elements in queue=w2150:i32)  [unwired: 2 in, 6 out]
        n755 = Get Notifier Status(notifier=w2147) -> (current notification=w2146:bool)  [unwired: 1 in, 4 out]
        n756 = Greater Than 0?(x=w2150) -> (x > 0?=w2149:bool)
        n757 = case shown="True" w2149 {
          tunnel: w2156 -> [_ w2186]
          tunnel: w2155 -> [w2158 w2187]
          tunnel: [w2158 w2185] -> w2154
          tunnel: w2153 -> [_ w2182]
          tunnel: w2152 -> [_ w2181]
          tunnel: w2151 -> [_ w2171]
          tunnel: w2148 -> [_ w2180]
          tunnel: w2145 -> [w2157 w2177]
          tunnel: [w2157 w2176] -> w2144
          tunnel: w2143 -> [_ w2175]
          tunnel: w2142 -> [_ w2174]
          tunnel: w2141 -> [_ w2169]
          tunnel: w2139 -> [_ w2167]
          tunnel: w2138 -> [_ w2165]
          tunnel: w2137 -> [_ _]
          tunnel: w2136 -> [_ _]
          tunnel: w2135 -> [_ _]
          frame False {
          }
          frame True {
            # "True: Last Frame of frame accum"
            # "Current Line in Frame Accum"
            # "Current Line In Frame"
            n758 = Increment(x=w2177) -> (x+1=w2170:u32)
            n759 = Dequeue Element(queue=w2180) -> (element=w2192:u64[])  [unwired: 2 in, 3 out]
            n760 = Equal?(x=w2170, y=w2174) -> (x = y?=w2179:bool)
            n761 = Greater?(x=w2170, y=w2175) -> (0:w2172:bool)
            n762 = Greater?(x=w2170, y=w2169) -> (0:w2168:bool)
            n763 = Split Number(x=w2192) -> (hi(x)=w2193:u32[])  [unwired: 1 out]
            n764 = Split Number(x=w2193) -> (hi(x)=w2164:u16[], lo(x)=w2163:u16[])
            n765 = Select(t=u32 0, s=w2179, f=w2170) -> (s? t:f=w2176:u32)
            n766 = Increment(x=w2187) -> (x+1=w2189:i32)
            n767 = Equal?(x=w2186, y=w2187) -> (x = y?=w2188:bool)
            n768 = To Single Precision Float(number=w2164) -> (single precision float=w2162:sgl[])
            n769 = To Single Precision Float(number=w2163) -> (single precision float=w2161:sgl[])
            n770 = Select(t=0, s=w2188, f=w2189) -> (s? t:f=w2185:i32)
            n771 = Add(x=w2162, y=w2161) -> (x+y=w2160:sgl[])
            n772 = Build Array(0, w2187, w2186, w2187) -> (w2184:i32[])
            n773 = case shown="False" w2168 {
              tunnel: [w2201 w2207] -> w2183
              tunnel: w2184 -> [_ w2205]
              tunnel: w2181 -> [w2200 w2204]
              tunnel: w2167 -> [w2199 w2203]
              tunnel: [w2199 w2203] -> w2166
              tunnel: w2160 -> [w2198 w2202]
              frame False {
                n774 = Divide(x=w2198, y=w2200) -> (x/y=w2201:sgl[])
              }
              frame True {
                n775 = call "IMAQ GetPixelLine"("Line Coordinates"=w2205, "Image"=w2203) -> ("Pixels Line (Float)"=w2206:sgl[])  [unwired: 2 in, 4 out]
                n776 = Divide(x=w2202, y=w2204) -> (x/y=w2208:sgl[])
                n777 = Add(x=w2206, y=w2208) -> (x+y=w2207:sgl[])
              }
            }
            n778 = call "IMAQ SetPixelLine"("Pixels Line (Float)"=w2183, "Line Coordinates"=w2184, "Image"=w2166) -> ()  [unwired: 7 in, 2 out]
            n779 = To Unsigned Word Integer(number=w2183) -> (unsigned 16bit integer=w2159:u16[])
            n780 = And(x=w2172, y=w2171) -> (x .and. y?=w2173:bool)
            n781 = case shown="True" w2173 {
              tunnel: w2159 -> [_ w2197]
              tunnel: w2182 -> [_ w2195]
              tunnel: w2165 -> [_ w2194]
              frame False {
              }
              frame True {
                n782 = Write to Binary File(file (use dialog)=w2194, data=w2197, 5:FALSE ("prepend array or string size? (T)"), 9:w2195) -> ()  [unwired: 2 in, 3 out]
              }
            }
          }
        }
      }
    }
    frame 21 {
      n783 = while {
        shift-right: [w2244] -> _
        shift-left: 0 -> [w2245]
        tunnel: w2223 -> [w2246]
        tunnel: w2222 -> [w2243]
        tunnel: w2221 -> [w2242]
        tunnel: w2220 -> [w2241]
        tunnel: w2219 -> [w2237]
        shift-right: [w2234] -> _
        shift-left: u32 0 -> [w2235]
        tunnel: w2217 -> [w2233]
        tunnel: w2216 -> [w2232]
        tunnel: w2215 -> [w2231]
        tunnel: w2214 -> [w2230]
        tunnel: w2209 -> [w2229]
        tunnel: w2213 -> [w2228]
        tunnel: w2212 -> [w2227]
        tunnel: w2211 -> [w2226]
        tunnel: w2210 -> [w2225]
        stop <- w2236 stop-if-true
        n784 = Get Queue Status(queue=w2230) -> (queue out=w2238:refnum<queue>, # elements in queue=w2240:i32)  [unwired: 2 in, 6 out]
        n785 = Get Notifier Status(notifier=w2237) -> (current notification=w2236:bool)  [unwired: 1 in, 4 out]
        n786 = Greater Than 0?(x=w2240) -> (x > 0?=w2239:bool)
        n787 = case shown="True" w2239 {
          tunnel: w2246 -> [_ w2276]
          tunnel: w2245 -> [w2248 w2277]
          tunnel: [w2248 w2275] -> w2244
          tunnel: w2243 -> [_ w2272]
          tunnel: w2242 -> [_ w2271]
          tunnel: w2241 -> [_ w2261]
          tunnel: w2238 -> [_ w2270]
          tunnel: w2235 -> [w2247 w2267]
          tunnel: [w2247 w2266] -> w2234
          tunnel: w2233 -> [_ w2265]
          tunnel: w2232 -> [_ w2264]
          tunnel: w2231 -> [_ w2259]
          tunnel: w2229 -> [_ w2257]
          tunnel: w2228 -> [_ w2255]
          tunnel: w2227 -> [_ _]
          tunnel: w2226 -> [_ _]
          tunnel: w2225 -> [_ _]
          frame False {
          }
          frame True {
            # "True: Last Frame of frame accum"
            # "Current Line in Frame Accum"
            # "Current Line In Frame"
            n788 = Increment(x=w2267) -> (x+1=w2260:u32)
            n789 = Dequeue Element(queue=w2270) -> (element=w2283:u64[])  [unwired: 2 in, 3 out]
            n790 = Equal?(x=w2260, y=w2264) -> (x = y?=w2269:bool)
            n791 = Greater?(x=w2260, y=w2265) -> (0:w2262:bool)
            n792 = Greater?(x=w2260, y=w2259) -> (0:w2258:bool)
            n793 = Split Number(x=w2283) -> (hi(x)=w2284:u32[], lo(x)=w2282:u32[])
            n794 = Split Number(x=w2284) -> (hi(x)=w2254:u16[])  [unwired: 1 out]
            n795 = Split Number(x=w2282) -> (hi(x)=w2250:u16[])  [unwired: 1 out]
            n796 = Select(t=u32 0, s=w2269, f=w2260) -> (s? t:f=w2266:u32)
            n797 = Increment(x=w2277) -> (x+1=w2279:i32)
            n798 = Equal?(x=w2276, y=w2277) -> (x = y?=w2278:bool)
            n799 = To Single Precision Float(number=w2254) -> (single precision float=w2253:sgl[])
            n800 = To Single Precision Float(number=w2250) -> (single precision float=w2252:sgl[])
            n801 = Select(t=0, s=w2278, f=w2279) -> (s? t:f=w2275:i32)
            n802 = Add(x=w2253, y=w2252) -> (x+y=w2251:sgl[])
            n803 = Build Array(0, w2277, w2276, w2277) -> (w2274:i32[])
            n804 = case shown="False" w2258 {
              tunnel: [w2292 w2298] -> w2273
              tunnel: w2274 -> [_ w2296]
              tunnel: w2271 -> [w2291 w2295]
              tunnel: w2257 -> [w2290 w2294]
              tunnel: [w2290 w2294] -> w2256
              tunnel: w2251 -> [w2289 w2293]
              frame False {
                n805 = Divide(x=w2289, y=w2291) -> (x/y=w2292:sgl[])
              }
              frame True {
                n806 = call "IMAQ GetPixelLine"("Line Coordinates"=w2296, "Image"=w2294) -> ("Pixels Line (Float)"=w2297:sgl[])  [unwired: 2 in, 4 out]
                n807 = Divide(x=w2293, y=w2295) -> (x/y=w2299:sgl[])
                n808 = Add(x=w2297, y=w2299) -> (x+y=w2298:sgl[])
              }
            }
            n809 = call "IMAQ SetPixelLine"("Pixels Line (Float)"=w2273, "Line Coordinates"=w2274, "Image"=w2256) -> ()  [unwired: 7 in, 2 out]
            n810 = To Unsigned Word Integer(number=w2273) -> (unsigned 16bit integer=w2249:u16[])
            n811 = And(x=w2262, y=w2261) -> (x .and. y?=w2263:bool)
            n812 = case shown="True" w2263 {
              tunnel: w2249 -> [_ w2288]
              tunnel: w2272 -> [_ w2286]
              tunnel: w2255 -> [_ w2285]
              frame False {
              }
              frame True {
                n813 = Write to Binary File(file (use dialog)=w2285, data=w2288, 5:FALSE ("prepend array or string size? (T)"), 9:w2286) -> ()  [unwired: 2 in, 3 out]
              }
            }
          }
        }
      }
    }
    frame 22 {
      n814 = while {
        shift-right: [w2335] -> _
        shift-left: 0 -> [w2336]
        tunnel: w2314 -> [w2337]
        tunnel: w2313 -> [w2334]
        tunnel: w2312 -> [w2333]
        tunnel: w2311 -> [w2332]
        tunnel: w2310 -> [w2328]
        shift-right: [w2325] -> _
        shift-left: u32 0 -> [w2326]
        tunnel: w2308 -> [w2324]
        tunnel: w2307 -> [w2323]
        tunnel: w2306 -> [w2322]
        tunnel: w2305 -> [w2321]
        tunnel: w2300 -> [w2320]
        tunnel: w2304 -> [w2319]
        tunnel: w2303 -> [w2318]
        tunnel: w2302 -> [w2317]
        tunnel: w2301 -> [w2316]
        stop <- w2327 stop-if-true
        n815 = Get Queue Status(queue=w2321) -> (queue out=w2329:refnum<queue>, # elements in queue=w2331:i32)  [unwired: 2 in, 6 out]
        n816 = Get Notifier Status(notifier=w2328) -> (current notification=w2327:bool)  [unwired: 1 in, 4 out]
        n817 = Greater Than 0?(x=w2331) -> (x > 0?=w2330:bool)
        n818 = case shown="True" w2330 {
          tunnel: w2337 -> [_ w2367]
          tunnel: w2336 -> [w2339 w2368]
          tunnel: [w2339 w2366] -> w2335
          tunnel: w2334 -> [_ w2363]
          tunnel: w2333 -> [_ w2362]
          tunnel: w2332 -> [_ w2352]
          tunnel: w2329 -> [_ w2361]
          tunnel: w2326 -> [w2338 w2358]
          tunnel: [w2338 w2357] -> w2325
          tunnel: w2324 -> [_ w2356]
          tunnel: w2323 -> [_ w2355]
          tunnel: w2322 -> [_ w2350]
          tunnel: w2320 -> [_ w2348]
          tunnel: w2319 -> [_ w2346]
          tunnel: w2318 -> [_ _]
          tunnel: w2317 -> [_ _]
          tunnel: w2316 -> [_ _]
          frame False {
          }
          frame True {
            # "True: Last Frame of frame accum"
            # "Current Line in Frame Accum"
            # "Current Line In Frame"
            n819 = Increment(x=w2358) -> (x+1=w2351:u32)
            n820 = Dequeue Element(queue=w2361) -> (element=w2374:u64[])  [unwired: 2 in, 3 out]
            n821 = Equal?(x=w2351, y=w2355) -> (x = y?=w2360:bool)
            n822 = Greater?(x=w2351, y=w2356) -> (0:w2353:bool)
            n823 = Greater?(x=w2351, y=w2350) -> (0:w2349:bool)
            n824 = Split Number(x=w2374) -> (hi(x)=w2375:u32[], lo(x)=w2373:u32[])
            n825 = Split Number(x=w2375) -> (lo(x)=w2341:u16[])  [unwired: 1 out]
            n826 = Split Number(x=w2373) -> (hi(x)=w2342:u16[])  [unwired: 1 out]
            n827 = Select(t=u32 0, s=w2360, f=w2351) -> (s? t:f=w2357:u32)
            n828 = Increment(x=w2368) -> (x+1=w2370:i32)
            n829 = Equal?(x=w2367, y=w2368) -> (x = y?=w2369:bool)
            n830 = To Single Precision Float(number=w2341) -> (single precision float=w2345:sgl[])
            n831 = To Single Precision Float(number=w2342) -> (single precision float=w2344:sgl[])
            n832 = Select(t=0, s=w2369, f=w2370) -> (s? t:f=w2366:i32)
            n833 = Add(x=w2345, y=w2344) -> (x+y=w2343:sgl[])
            n834 = Build Array(0, w2368, w2367, w2368) -> (w2365:i32[])
            n835 = case shown="False" w2349 {
              tunnel: [w2383 w2389] -> w2364
              tunnel: w2365 -> [_ w2387]
              tunnel: w2362 -> [w2382 w2386]
              tunnel: w2348 -> [w2381 w2385]
              tunnel: [w2381 w2385] -> w2347
              tunnel: w2343 -> [w2380 w2384]
              frame False {
                n836 = Divide(x=w2380, y=w2382) -> (x/y=w2383:sgl[])
              }
              frame True {
                n837 = call "IMAQ GetPixelLine"("Line Coordinates"=w2387, "Image"=w2385) -> ("Pixels Line (Float)"=w2388:sgl[])  [unwired: 2 in, 4 out]
                n838 = Divide(x=w2384, y=w2386) -> (x/y=w2390:sgl[])
                n839 = Add(x=w2388, y=w2390) -> (x+y=w2389:sgl[])
              }
            }
            n840 = call "IMAQ SetPixelLine"("Pixels Line (Float)"=w2364, "Line Coordinates"=w2365, "Image"=w2347) -> ()  [unwired: 7 in, 2 out]
            n841 = To Unsigned Word Integer(number=w2364) -> (unsigned 16bit integer=w2340:u16[])
            n842 = And(x=w2353, y=w2352) -> (x .and. y?=w2354:bool)
            n843 = case shown="True" w2354 {
              tunnel: w2340 -> [_ w2379]
              tunnel: w2363 -> [_ w2377]
              tunnel: w2346 -> [_ w2376]
              frame False {
              }
              frame True {
                n844 = Write to Binary File(file (use dialog)=w2376, data=w2379, 5:FALSE ("prepend array or string size? (T)"), 9:w2377) -> ()  [unwired: 2 in, 3 out]
              }
            }
          }
        }
      }
    }
    frame 23 {
      n845 = while {
        shift-right: [w2426] -> _
        shift-left: 0 -> [w2427]
        tunnel: w2405 -> [w2428]
        tunnel: w2404 -> [w2425]
        tunnel: w2403 -> [w2424]
        tunnel: w2402 -> [w2423]
        tunnel: w2401 -> [w2419]
        shift-right: [w2416] -> _
        shift-left: u32 0 -> [w2417]
        tunnel: w2399 -> [w2415]
        tunnel: w2398 -> [w2414]
        tunnel: w2397 -> [w2413]
        tunnel: w2396 -> [w2412]
        tunnel: w2391 -> [w2411]
        tunnel: w2395 -> [w2410]
        tunnel: w2394 -> [w2409]
        tunnel: w2393 -> [w2408]
        tunnel: w2392 -> [w2407]
        stop <- w2418 stop-if-true
        n846 = Get Queue Status(queue=w2412) -> (queue out=w2420:refnum<queue>, # elements in queue=w2422:i32)  [unwired: 2 in, 6 out]
        n847 = Get Notifier Status(notifier=w2419) -> (current notification=w2418:bool)  [unwired: 1 in, 4 out]
        n848 = Greater Than 0?(x=w2422) -> (x > 0?=w2421:bool)
        n849 = case shown="True" w2421 {
          tunnel: w2428 -> [_ w2460]
          tunnel: w2427 -> [w2430 w2461]
          tunnel: [w2430 w2459] -> w2426
          tunnel: w2425 -> [_ w2456]
          tunnel: w2424 -> [_ w2455]
          tunnel: w2423 -> [_ w2445]
          tunnel: w2420 -> [_ w2454]
          tunnel: w2417 -> [w2429 w2451]
          tunnel: [w2429 w2450] -> w2416
          tunnel: w2415 -> [_ w2449]
          tunnel: w2414 -> [_ w2448]
          tunnel: w2413 -> [_ w2443]
          tunnel: w2411 -> [_ w2441]
          tunnel: w2410 -> [_ w2439]
          tunnel: w2409 -> [_ _]
          tunnel: w2408 -> [_ _]
          tunnel: w2407 -> [_ _]
          frame False {
          }
          frame True {
            # "True: Last Frame of frame accum"
            # "Current Line in Frame Accum"
            # "Current Line In Frame"
            n850 = Increment(x=w2451) -> (x+1=w2444:u32)
            n851 = Dequeue Element(queue=w2454) -> (element=w2467:u64[])  [unwired: 2 in, 3 out]
            n852 = Equal?(x=w2444, y=w2448) -> (x = y?=w2453:bool)
            n853 = Greater?(x=w2444, y=w2449) -> (0:w2446:bool)
            n854 = Greater?(x=w2444, y=w2443) -> (0:w2442:bool)
            n855 = Split Number(x=w2467) -> (hi(x)=w2468:u32[], lo(x)=w2466:u32[])
            n856 = Split Number(x=w2468) -> (hi(x)=w2437:u16[], lo(x)=w2436:u16[])
            n857 = Split Number(x=w2466) -> (hi(x)=w2438:u16[])  [unwired: 1 out]
            n858 = Select(t=u32 0, s=w2453, f=w2444) -> (s? t:f=w2450:u32)
            n859 = Increment(x=w2461) -> (x+1=w2463:i32)
            n860 = Equal?(x=w2460, y=w2461) -> (x = y?=w2462:bool)
            n861 = To Single Precision Float(number=w2437) -> (single precision float=w2435:sgl[])
            n862 = To Single Precision Float(number=w2436) -> (single precision float=w2433:sgl[])
            n863 = To Single Precision Float(number=w2438) -> (single precision float=w2434:sgl[])
            n864 = Select(t=0, s=w2462, f=w2463) -> (s? t:f=w2459:i32)
            n865 = Compound Arithmetic op=ADD(w2435, w2433, w2434) -> (w2432:sgl[])
            n866 = Build Array(0, w2461, w2460, w2461) -> (w2458:i32[])
            n867 = case shown="False" w2442 {
              tunnel: [w2476 w2482] -> w2457
              tunnel: w2458 -> [_ w2480]
              tunnel: w2455 -> [w2475 w2479]
              tunnel: w2441 -> [w2474 w2478]
              tunnel: [w2474 w2478] -> w2440
              tunnel: w2432 -> [w2473 w2477]
              frame False {
                n868 = Divide(x=w2473, y=w2475) -> (x/y=w2476:sgl[])
              }
              frame True {
                n869 = call "IMAQ GetPixelLine"("Line Coordinates"=w2480, "Image"=w2478) -> ("Pixels Line (Float)"=w2481:sgl[])  [unwired: 2 in, 4 out]
                n870 = Divide(x=w2477, y=w2479) -> (x/y=w2483:sgl[])
                n871 = Add(x=w2481, y=w2483) -> (x+y=w2482:sgl[])
              }
            }
            n872 = call "IMAQ SetPixelLine"("Pixels Line (Float)"=w2457, "Line Coordinates"=w2458, "Image"=w2440) -> ()  [unwired: 7 in, 2 out]
            n873 = To Unsigned Word Integer(number=w2457) -> (unsigned 16bit integer=w2431:u16[])
            n874 = And(x=w2446, y=w2445) -> (x .and. y?=w2447:bool)
            n875 = case shown="True" w2447 {
              tunnel: w2431 -> [_ w2472]
              tunnel: w2456 -> [_ w2470]
              tunnel: w2439 -> [_ w2469]
              frame False {
              }
              frame True {
                n876 = Write to Binary File(file (use dialog)=w2469, data=w2472, 5:FALSE ("prepend array or string size? (T)"), 9:w2470) -> ()  [unwired: 2 in, 3 out]
              }
            }
          }
        }
      }
    }
    frame 25 {
      n877 = while {
        shift-right: [w2519] -> _
        shift-left: 0 -> [w2520]
        tunnel: w2498 -> [w2521]
        tunnel: w2497 -> [w2518]
        tunnel: w2496 -> [w2517]
        tunnel: w2495 -> [w2516]
        tunnel: w2494 -> [w2512]
        shift-right: [w2509] -> _
        shift-left: u32 0 -> [w2510]
        tunnel: w2492 -> [w2508]
        tunnel: w2491 -> [w2507]
        tunnel: w2490 -> [w2506]
        tunnel: w2489 -> [w2505]
        tunnel: w2484 -> [w2504]
        tunnel: w2488 -> [w2503]
        tunnel: w2487 -> [w2502]
        tunnel: w2486 -> [w2501]
        tunnel: w2485 -> [w2500]
        stop <- w2511 stop-if-true
        n878 = Get Queue Status(queue=w2505) -> (queue out=w2513:refnum<queue>, # elements in queue=w2515:i32)  [unwired: 2 in, 6 out]
        n879 = Get Notifier Status(notifier=w2512) -> (current notification=w2511:bool)  [unwired: 1 in, 4 out]
        n880 = Greater Than 0?(x=w2515) -> (x > 0?=w2514:bool)
        n881 = case shown="True" w2514 {
          tunnel: w2521 -> [_ w2551]
          tunnel: w2520 -> [w2523 w2552]
          tunnel: [w2523 w2550] -> w2519
          tunnel: w2518 -> [_ w2547]
          tunnel: w2517 -> [_ w2546]
          tunnel: w2516 -> [_ w2536]
          tunnel: w2513 -> [_ w2545]
          tunnel: w2510 -> [w2522 w2542]
          tunnel: [w2522 w2541] -> w2509
          tunnel: w2508 -> [_ w2540]
          tunnel: w2507 -> [_ w2539]
          tunnel: w2506 -> [_ w2534]
          tunnel: w2504 -> [_ w2532]
          tunnel: w2503 -> [_ w2530]
          tunnel: w2502 -> [_ _]
          tunnel: w2501 -> [_ _]
          tunnel: w2500 -> [_ _]
          frame False {
          }
          frame True {
            # "True: Last Frame of frame accum"
            # "Current Line in Frame Accum"
            # "Current Line In Frame"
            n882 = Increment(x=w2542) -> (x+1=w2535:u32)
            n883 = Dequeue Element(queue=w2545) -> (element=w2558:u64[])  [unwired: 2 in, 3 out]
            n884 = Equal?(x=w2535, y=w2539) -> (x = y?=w2544:bool)
            n885 = Greater?(x=w2535, y=w2540) -> (0:w2537:bool)
            n886 = Greater?(x=w2535, y=w2534) -> (0:w2533:bool)
            n887 = Split Number(x=w2558) -> (hi(x)=w2559:u32[], lo(x)=w2557:u32[])
            n888 = Split Number(x=w2559) -> (hi(x)=w2525:u16[])  [unwired: 1 out]
            n889 = Split Number(x=w2557) -> (lo(x)=w2526:u16[])  [unwired: 1 out]
            n890 = Select(t=u32 0, s=w2544, f=w2535) -> (s? t:f=w2541:u32)
            n891 = Increment(x=w2552) -> (x+1=w2554:i32)
            n892 = Equal?(x=w2551, y=w2552) -> (x = y?=w2553:bool)
            n893 = To Single Precision Float(number=w2525) -> (single precision float=w2529:sgl[])
            n894 = To Single Precision Float(number=w2526) -> (single precision float=w2528:sgl[])
            n895 = Select(t=0, s=w2553, f=w2554) -> (s? t:f=w2550:i32)
            n896 = Add(x=w2529, y=w2528) -> (x+y=w2527:sgl[])
            n897 = Build Array(0, w2552, w2551, w2552) -> (w2549:i32[])
            n898 = case shown="False" w2533 {
              tunnel: [w2567 w2573] -> w2548
              tunnel: w2549 -> [_ w2571]
              tunnel: w2546 -> [w2566 w2570]
              tunnel: w2532 -> [w2565 w2569]
              tunnel: [w2565 w2569] -> w2531
              tunnel: w2527 -> [w2564 w2568]
              frame False {
                n899 = Divide(x=w2564, y=w2566) -> (x/y=w2567:sgl[])
              }
              frame True {
                n900 = call "IMAQ GetPixelLine"("Line Coordinates"=w2571, "Image"=w2569) -> ("Pixels Line (Float)"=w2572:sgl[])  [unwired: 2 in, 4 out]
                n901 = Divide(x=w2568, y=w2570) -> (x/y=w2574:sgl[])
                n902 = Add(x=w2572, y=w2574) -> (x+y=w2573:sgl[])
              }
            }
            n903 = call "IMAQ SetPixelLine"("Pixels Line (Float)"=w2548, "Line Coordinates"=w2549, "Image"=w2531) -> ()  [unwired: 7 in, 2 out]
            n904 = To Unsigned Word Integer(number=w2548) -> (unsigned 16bit integer=w2524:u16[])
            n905 = And(x=w2537, y=w2536) -> (x .and. y?=w2538:bool)
            n906 = case shown="True" w2538 {
              tunnel: w2524 -> [_ w2563]
              tunnel: w2547 -> [_ w2561]
              tunnel: w2530 -> [_ w2560]
              frame False {
              }
              frame True {
                n907 = Write to Binary File(file (use dialog)=w2560, data=w2563, 5:FALSE ("prepend array or string size? (T)"), 9:w2561) -> ()  [unwired: 2 in, 3 out]
              }
            }
          }
        }
      }
    }
    frame 26 {
      n908 = while {
        shift-right: [w2610] -> _
        shift-left: 0 -> [w2611]
        tunnel: w2589 -> [w2612]
        tunnel: w2588 -> [w2609]
        tunnel: w2587 -> [w2608]
        tunnel: w2586 -> [w2607]
        tunnel: w2585 -> [w2603]
        shift-right: [w2600] -> _
        shift-left: u32 0 -> [w2601]
        tunnel: w2583 -> [w2599]
        tunnel: w2582 -> [w2598]
        tunnel: w2581 -> [w2597]
        tunnel: w2580 -> [w2596]
        tunnel: w2575 -> [w2595]
        tunnel: w2579 -> [w2594]
        tunnel: w2578 -> [w2593]
        tunnel: w2577 -> [w2592]
        tunnel: w2576 -> [w2591]
        stop <- w2602 stop-if-true
        n909 = Get Queue Status(queue=w2596) -> (queue out=w2604:refnum<queue>, # elements in queue=w2606:i32)  [unwired: 2 in, 6 out]
        n910 = Get Notifier Status(notifier=w2603) -> (current notification=w2602:bool)  [unwired: 1 in, 4 out]
        n911 = Greater Than 0?(x=w2606) -> (x > 0?=w2605:bool)
        n912 = case shown="True" w2605 {
          tunnel: w2612 -> [_ w2642]
          tunnel: w2611 -> [w2614 w2643]
          tunnel: [w2614 w2641] -> w2610
          tunnel: w2609 -> [_ w2638]
          tunnel: w2608 -> [_ w2637]
          tunnel: w2607 -> [_ w2627]
          tunnel: w2604 -> [_ w2636]
          tunnel: w2601 -> [w2613 w2633]
          tunnel: [w2613 w2632] -> w2600
          tunnel: w2599 -> [_ w2631]
          tunnel: w2598 -> [_ w2630]
          tunnel: w2597 -> [_ w2625]
          tunnel: w2595 -> [_ w2623]
          tunnel: w2594 -> [_ w2621]
          tunnel: w2593 -> [_ _]
          tunnel: w2592 -> [_ _]
          tunnel: w2591 -> [_ _]
          frame False {
          }
          frame True {
            # "True: Last Frame of frame accum"
            # "Current Line in Frame Accum"
            # "Current Line In Frame"
            n913 = Increment(x=w2633) -> (x+1=w2626:u32)
            n914 = Dequeue Element(queue=w2636) -> (element=w2649:u64[])  [unwired: 2 in, 3 out]
            n915 = Equal?(x=w2626, y=w2630) -> (x = y?=w2635:bool)
            n916 = Greater?(x=w2626, y=w2631) -> (0:w2628:bool)
            n917 = Greater?(x=w2626, y=w2625) -> (0:w2624:bool)
            n918 = Split Number(x=w2649) -> (hi(x)=w2650:u32[], lo(x)=w2648:u32[])
            n919 = Split Number(x=w2650) -> (lo(x)=w2617:u16[])  [unwired: 1 out]
            n920 = Split Number(x=w2648) -> (lo(x)=w2616:u16[])  [unwired: 1 out]
            n921 = Select(t=u32 0, s=w2635, f=w2626) -> (s? t:f=w2632:u32)
            n922 = Increment(x=w2643) -> (x+1=w2645:i32)
            n923 = Equal?(x=w2642, y=w2643) -> (x = y?=w2644:bool)
            n924 = To Single Precision Float(number=w2617) -> (single precision float=w2620:sgl[])
            n925 = To Single Precision Float(number=w2616) -> (single precision float=w2619:sgl[])
            n926 = Select(t=0, s=w2644, f=w2645) -> (s? t:f=w2641:i32)
            n927 = Add(x=w2620, y=w2619) -> (x+y=w2618:sgl[])
            n928 = Build Array(0, w2643, w2642, w2643) -> (w2640:i32[])
            n929 = case shown="False" w2624 {
              tunnel: [w2658 w2664] -> w2639
              tunnel: w2640 -> [_ w2662]
              tunnel: w2637 -> [w2657 w2661]
              tunnel: w2623 -> [w2656 w2660]
              tunnel: [w2656 w2660] -> w2622
              tunnel: w2618 -> [w2655 w2659]
              frame False {
                n930 = Divide(x=w2655, y=w2657) -> (x/y=w2658:sgl[])
              }
              frame True {
                n931 = call "IMAQ GetPixelLine"("Line Coordinates"=w2662, "Image"=w2660) -> ("Pixels Line (Float)"=w2663:sgl[])  [unwired: 2 in, 4 out]
                n932 = Divide(x=w2659, y=w2661) -> (x/y=w2665:sgl[])
                n933 = Add(x=w2663, y=w2665) -> (x+y=w2664:sgl[])
              }
            }
            n934 = call "IMAQ SetPixelLine"("Pixels Line (Float)"=w2639, "Line Coordinates"=w2640, "Image"=w2622) -> ()  [unwired: 7 in, 2 out]
            n935 = To Unsigned Word Integer(number=w2639) -> (unsigned 16bit integer=w2615:u16[])
            n936 = And(x=w2628, y=w2627) -> (x .and. y?=w2629:bool)
            n937 = case shown="True" w2629 {
              tunnel: w2615 -> [_ w2654]
              tunnel: w2638 -> [_ w2652]
              tunnel: w2621 -> [_ w2651]
              frame False {
              }
              frame True {
                n938 = Write to Binary File(file (use dialog)=w2651, data=w2654, 5:FALSE ("prepend array or string size? (T)"), 9:w2652) -> ()  [unwired: 2 in, 3 out]
              }
            }
          }
        }
      }
    }
    frame 27 {
      n939 = while {
        shift-right: [w2701] -> _
        shift-left: 0 -> [w2702]
        tunnel: w2680 -> [w2703]
        tunnel: w2679 -> [w2700]
        tunnel: w2678 -> [w2699]
        tunnel: w2677 -> [w2698]
        tunnel: w2676 -> [w2694]
        shift-right: [w2691] -> _
        shift-left: u32 0 -> [w2692]
        tunnel: w2674 -> [w2690]
        tunnel: w2673 -> [w2689]
        tunnel: w2672 -> [w2688]
        tunnel: w2671 -> [w2687]
        tunnel: w2666 -> [w2686]
        tunnel: w2670 -> [w2685]
        tunnel: w2669 -> [w2684]
        tunnel: w2668 -> [w2683]
        tunnel: w2667 -> [w2682]
        stop <- w2693 stop-if-true
        n940 = Get Queue Status(queue=w2687) -> (queue out=w2695:refnum<queue>, # elements in queue=w2697:i32)  [unwired: 2 in, 6 out]
        n941 = Get Notifier Status(notifier=w2694) -> (current notification=w2693:bool)  [unwired: 1 in, 4 out]
        n942 = Greater Than 0?(x=w2697) -> (x > 0?=w2696:bool)
        n943 = case shown="True" w2696 {
          tunnel: w2703 -> [_ w2735]
          tunnel: w2702 -> [w2705 w2736]
          tunnel: [w2705 w2734] -> w2701
          tunnel: w2700 -> [_ w2731]
          tunnel: w2699 -> [_ w2730]
          tunnel: w2698 -> [_ w2720]
          tunnel: w2695 -> [_ w2729]
          tunnel: w2692 -> [w2704 w2726]
          tunnel: [w2704 w2725] -> w2691
          tunnel: w2690 -> [_ w2724]
          tunnel: w2689 -> [_ w2723]
          tunnel: w2688 -> [_ w2718]
          tunnel: w2686 -> [_ w2716]
          tunnel: w2685 -> [_ w2714]
          tunnel: w2684 -> [_ _]
          tunnel: w2683 -> [_ _]
          tunnel: w2682 -> [_ _]
          frame False {
          }
          frame True {
            # "True: Last Frame of frame accum"
            # "Current Line in Frame Accum"
            # "Current Line In Frame"
            n944 = Increment(x=w2726) -> (x+1=w2719:u32)
            n945 = Dequeue Element(queue=w2729) -> (element=w2742:u64[])  [unwired: 2 in, 3 out]
            n946 = Equal?(x=w2719, y=w2723) -> (x = y?=w2728:bool)
            n947 = Greater?(x=w2719, y=w2724) -> (0:w2721:bool)
            n948 = Greater?(x=w2719, y=w2718) -> (0:w2717:bool)
            n949 = Split Number(x=w2742) -> (hi(x)=w2743:u32[], lo(x)=w2741:u32[])
            n950 = Split Number(x=w2743) -> (hi(x)=w2713:u16[], lo(x)=w2712:u16[])
            n951 = Split Number(x=w2741) -> (lo(x)=w2707:u16[])  [unwired: 1 out]
            n952 = Select(t=u32 0, s=w2728, f=w2719) -> (s? t:f=w2725:u32)
            n953 = Increment(x=w2736) -> (x+1=w2738:i32)
            n954 = Equal?(x=w2735, y=w2736) -> (x = y?=w2737:bool)
            n955 = To Single Precision Float(number=w2713) -> (single precision float=w2711:sgl[])
            n956 = To Single Precision Float(number=w2712) -> (single precision float=w2709:sgl[])
            n957 = To Single Precision Float(number=w2707) -> (single precision float=w2710:sgl[])
            n958 = Select(t=0, s=w2737, f=w2738) -> (s? t:f=w2734:i32)
            n959 = Compound Arithmetic op=ADD(w2711, w2709, w2710) -> (w2708:sgl[])
            n960 = Build Array(0, w2736, w2735, w2736) -> (w2733:i32[])
            n961 = case shown="False" w2717 {
              tunnel: [w2751 w2757] -> w2732
              tunnel: w2733 -> [_ w2755]
              tunnel: w2730 -> [w2750 w2754]
              tunnel: w2716 -> [w2749 w2753]
              tunnel: [w2749 w2753] -> w2715
              tunnel: w2708 -> [w2748 w2752]
              frame False {
                n962 = Divide(x=w2748, y=w2750) -> (x/y=w2751:sgl[])
              }
              frame True {
                n963 = call "IMAQ GetPixelLine"("Line Coordinates"=w2755, "Image"=w2753) -> ("Pixels Line (Float)"=w2756:sgl[])  [unwired: 2 in, 4 out]
                n964 = Divide(x=w2752, y=w2754) -> (x/y=w2758:sgl[])
                n965 = Add(x=w2756, y=w2758) -> (x+y=w2757:sgl[])
              }
            }
            n966 = call "IMAQ SetPixelLine"("Pixels Line (Float)"=w2732, "Line Coordinates"=w2733, "Image"=w2715) -> ()  [unwired: 7 in, 2 out]
            n967 = To Unsigned Word Integer(number=w2732) -> (unsigned 16bit integer=w2706:u16[])
            n968 = And(x=w2721, y=w2720) -> (x .and. y?=w2722:bool)
            n969 = case shown="True" w2722 {
              tunnel: w2706 -> [_ w2747]
              tunnel: w2731 -> [_ w2745]
              tunnel: w2714 -> [_ w2744]
              frame False {
              }
              frame True {
                n970 = Write to Binary File(file (use dialog)=w2744, data=w2747, 5:FALSE ("prepend array or string size? (T)"), 9:w2745) -> ()  [unwired: 2 in, 3 out]
              }
            }
          }
        }
      }
    }
    frame 28 {
      n971 = while {
        shift-right: [w2794] -> _
        shift-left: 0 -> [w2795]
        tunnel: w2773 -> [w2796]
        tunnel: w2772 -> [w2793]
        tunnel: w2771 -> [w2792]
        tunnel: w2770 -> [w2791]
        tunnel: w2769 -> [w2787]
        shift-right: [w2784] -> _
        shift-left: u32 0 -> [w2785]
        tunnel: w2767 -> [w2783]
        tunnel: w2766 -> [w2782]
        tunnel: w2765 -> [w2781]
        tunnel: w2764 -> [w2780]
        tunnel: w2759 -> [w2779]
        tunnel: w2763 -> [w2778]
        tunnel: w2762 -> [w2777]
        tunnel: w2761 -> [w2776]
        tunnel: w2760 -> [w2775]
        stop <- w2786 stop-if-true
        n972 = Get Queue Status(queue=w2780) -> (queue out=w2788:refnum<queue>, # elements in queue=w2790:i32)  [unwired: 2 in, 6 out]
        n973 = Get Notifier Status(notifier=w2787) -> (current notification=w2786:bool)  [unwired: 1 in, 4 out]
        n974 = Greater Than 0?(x=w2790) -> (x > 0?=w2789:bool)
        n975 = case shown="True" w2789 {
          tunnel: w2796 -> [_ w2826]
          tunnel: w2795 -> [w2798 w2827]
          tunnel: [w2798 w2825] -> w2794
          tunnel: w2793 -> [_ w2822]
          tunnel: w2792 -> [_ w2821]
          tunnel: w2791 -> [_ w2811]
          tunnel: w2788 -> [_ w2820]
          tunnel: w2785 -> [w2797 w2817]
          tunnel: [w2797 w2816] -> w2784
          tunnel: w2783 -> [_ w2815]
          tunnel: w2782 -> [_ w2814]
          tunnel: w2781 -> [_ w2809]
          tunnel: w2779 -> [_ w2807]
          tunnel: w2778 -> [_ w2805]
          tunnel: w2777 -> [_ _]
          tunnel: w2776 -> [_ _]
          tunnel: w2775 -> [_ _]
          frame False {
          }
          frame True {
            # "True: Last Frame of frame accum"
            # "Current Line in Frame Accum"
            # "Current Line In Frame"
            n976 = Increment(x=w2817) -> (x+1=w2810:u32)
            n977 = Dequeue Element(queue=w2820) -> (element=w2833:u64[])  [unwired: 2 in, 3 out]
            n978 = Equal?(x=w2810, y=w2814) -> (x = y?=w2819:bool)
            n979 = Greater?(x=w2810, y=w2815) -> (0:w2812:bool)
            n980 = Greater?(x=w2810, y=w2809) -> (0:w2808:bool)
            n981 = Split Number(x=w2833) -> (lo(x)=w2832:u32[])  [unwired: 1 out]
            n982 = Split Number(x=w2832) -> (hi(x)=w2800:u16[], lo(x)=w2801:u16[])
            n983 = Select(t=u32 0, s=w2819, f=w2810) -> (s? t:f=w2816:u32)
            n984 = Increment(x=w2827) -> (x+1=w2829:i32)
            n985 = Equal?(x=w2826, y=w2827) -> (x = y?=w2828:bool)
            n986 = To Single Precision Float(number=w2800) -> (single precision float=w2804:sgl[])
            n987 = To Single Precision Float(number=w2801) -> (single precision float=w2803:sgl[])
            n988 = Select(t=0, s=w2828, f=w2829) -> (s? t:f=w2825:i32)
            n989 = Add(x=w2804, y=w2803) -> (x+y=w2802:sgl[])
            n990 = Build Array(0, w2827, w2826, w2827) -> (w2824:i32[])
            n991 = case shown="False" w2808 {
              tunnel: [w2841 w2847] -> w2823
              tunnel: w2824 -> [_ w2845]
              tunnel: w2821 -> [w2840 w2844]
              tunnel: w2807 -> [w2839 w2843]
              tunnel: [w2839 w2843] -> w2806
              tunnel: w2802 -> [w2838 w2842]
              frame False {
                n992 = Divide(x=w2838, y=w2840) -> (x/y=w2841:sgl[])
              }
              frame True {
                n993 = call "IMAQ GetPixelLine"("Line Coordinates"=w2845, "Image"=w2843) -> ("Pixels Line (Float)"=w2846:sgl[])  [unwired: 2 in, 4 out]
                n994 = Divide(x=w2842, y=w2844) -> (x/y=w2848:sgl[])
                n995 = Add(x=w2846, y=w2848) -> (x+y=w2847:sgl[])
              }
            }
            n996 = call "IMAQ SetPixelLine"("Pixels Line (Float)"=w2823, "Line Coordinates"=w2824, "Image"=w2806) -> ()  [unwired: 7 in, 2 out]
            n997 = To Unsigned Word Integer(number=w2823) -> (unsigned 16bit integer=w2799:u16[])
            n998 = And(x=w2812, y=w2811) -> (x .and. y?=w2813:bool)
            n999 = case shown="True" w2813 {
              tunnel: w2799 -> [_ w2837]
              tunnel: w2822 -> [_ w2835]
              tunnel: w2805 -> [_ w2834]
              frame False {
              }
              frame True {
                n1000 = Write to Binary File(file (use dialog)=w2834, data=w2837, 5:FALSE ("prepend array or string size? (T)"), 9:w2835) -> ()  [unwired: 2 in, 3 out]
              }
            }
          }
        }
      }
    }
    frame 29 {
      n1001 = while {
        shift-right: [w2884] -> _
        shift-left: 0 -> [w2885]
        tunnel: w2863 -> [w2886]
        tunnel: w2862 -> [w2883]
        tunnel: w2861 -> [w2882]
        tunnel: w2860 -> [w2881]
        tunnel: w2859 -> [w2877]
        shift-right: [w2874] -> _
        shift-left: u32 0 -> [w2875]
        tunnel: w2857 -> [w2873]
        tunnel: w2856 -> [w2872]
        tunnel: w2855 -> [w2871]
        tunnel: w2854 -> [w2870]
        tunnel: w2849 -> [w2869]
        tunnel: w2853 -> [w2868]
        tunnel: w2852 -> [w2867]
        tunnel: w2851 -> [w2866]
        tunnel: w2850 -> [w2865]
        stop <- w2876 stop-if-true
        n1002 = Get Queue Status(queue=w2870) -> (queue out=w2878:refnum<queue>, # elements in queue=w2880:i32)  [unwired: 2 in, 6 out]
        n1003 = Get Notifier Status(notifier=w2877) -> (current notification=w2876:bool)  [unwired: 1 in, 4 out]
        n1004 = Greater Than 0?(x=w2880) -> (x > 0?=w2879:bool)
        n1005 = case shown="True" w2879 {
          tunnel: w2886 -> [_ w2918]
          tunnel: w2885 -> [w2888 w2919]
          tunnel: [w2888 w2917] -> w2884
          tunnel: w2883 -> [_ w2914]
          tunnel: w2882 -> [_ w2913]
          tunnel: w2881 -> [_ w2903]
          tunnel: w2878 -> [_ w2912]
          tunnel: w2875 -> [w2887 w2909]
          tunnel: [w2887 w2908] -> w2874
          tunnel: w2873 -> [_ w2907]
          tunnel: w2872 -> [_ w2906]
          tunnel: w2871 -> [_ w2901]
          tunnel: w2869 -> [_ w2899]
          tunnel: w2868 -> [_ w2897]
          tunnel: w2867 -> [_ _]
          tunnel: w2866 -> [_ _]
          tunnel: w2865 -> [_ _]
          frame False {
          }
          frame True {
            # "True: Last Frame of frame accum"
            # "Current Line in Frame Accum"
            # "Current Line In Frame"
            n1006 = Increment(x=w2909) -> (x+1=w2902:u32)
            n1007 = Dequeue Element(queue=w2912) -> (element=w2925:u64[])  [unwired: 2 in, 3 out]
            n1008 = Equal?(x=w2902, y=w2906) -> (x = y?=w2911:bool)
            n1009 = Greater?(x=w2902, y=w2907) -> (0:w2904:bool)
            n1010 = Greater?(x=w2902, y=w2901) -> (0:w2900:bool)
            n1011 = Split Number(x=w2925) -> (hi(x)=w2926:u32[], lo(x)=w2924:u32[])
            n1012 = Split Number(x=w2926) -> (hi(x)=w2896:u16[])  [unwired: 1 out]
            n1013 = Split Number(x=w2924) -> (hi(x)=w2891:u16[], lo(x)=w2890:u16[])
            n1014 = Select(t=u32 0, s=w2911, f=w2902) -> (s? t:f=w2908:u32)
            n1015 = Increment(x=w2919) -> (x+1=w2921:i32)
            n1016 = Equal?(x=w2918, y=w2919) -> (x = y?=w2920:bool)
            n1017 = To Single Precision Float(number=w2896) -> (single precision float=w2895:sgl[])
            n1018 = To Single Precision Float(number=w2891) -> (single precision float=w2893:sgl[])
            n1019 = To Single Precision Float(number=w2890) -> (single precision float=w2894:sgl[])
            n1020 = Select(t=0, s=w2920, f=w2921) -> (s? t:f=w2917:i32)
            n1021 = Compound Arithmetic op=ADD(w2895, w2893, w2894) -> (w2892:sgl[])
            n1022 = Build Array(0, w2919, w2918, w2919) -> (w2916:i32[])
            n1023 = case shown="False" w2900 {
              tunnel: [w2934 w2940] -> w2915
              tunnel: w2916 -> [_ w2938]
              tunnel: w2913 -> [w2933 w2937]
              tunnel: w2899 -> [w2932 w2936]
              tunnel: [w2932 w2936] -> w2898
              tunnel: w2892 -> [w2931 w2935]
              frame False {
                n1024 = Divide(x=w2931, y=w2933) -> (x/y=w2934:sgl[])
              }
              frame True {
                n1025 = call "IMAQ GetPixelLine"("Line Coordinates"=w2938, "Image"=w2936) -> ("Pixels Line (Float)"=w2939:sgl[])  [unwired: 2 in, 4 out]
                n1026 = Divide(x=w2935, y=w2937) -> (x/y=w2941:sgl[])
                n1027 = Add(x=w2939, y=w2941) -> (x+y=w2940:sgl[])
              }
            }
            n1028 = call "IMAQ SetPixelLine"("Pixels Line (Float)"=w2915, "Line Coordinates"=w2916, "Image"=w2898) -> ()  [unwired: 7 in, 2 out]
            n1029 = To Unsigned Word Integer(number=w2915) -> (unsigned 16bit integer=w2889:u16[])
            n1030 = And(x=w2904, y=w2903) -> (x .and. y?=w2905:bool)
            n1031 = case shown="True" w2905 {
              tunnel: w2889 -> [_ w2930]
              tunnel: w2914 -> [_ w2928]
              tunnel: w2897 -> [_ w2927]
              frame False {
              }
              frame True {
                n1032 = Write to Binary File(file (use dialog)=w2927, data=w2930, 5:FALSE ("prepend array or string size? (T)"), 9:w2928) -> ()  [unwired: 2 in, 3 out]
              }
            }
          }
        }
      }
    }
    frame 30 {
      n1033 = while {
        shift-right: [w2977] -> _
        shift-left: 0 -> [w2978]
        tunnel: w2956 -> [w2979]
        tunnel: w2955 -> [w2976]
        tunnel: w2954 -> [w2975]
        tunnel: w2953 -> [w2974]
        tunnel: w2952 -> [w2970]
        shift-right: [w2967] -> _
        shift-left: u32 0 -> [w2968]
        tunnel: w2950 -> [w2966]
        tunnel: w2949 -> [w2965]
        tunnel: w2948 -> [w2964]
        tunnel: w2947 -> [w2963]
        tunnel: w2942 -> [w2962]
        tunnel: w2946 -> [w2961]
        tunnel: w2945 -> [w2960]
        tunnel: w2944 -> [w2959]
        tunnel: w2943 -> [w2958]
        stop <- w2969 stop-if-true
        n1034 = Get Queue Status(queue=w2963) -> (queue out=w2971:refnum<queue>, # elements in queue=w2973:i32)  [unwired: 2 in, 6 out]
        n1035 = Get Notifier Status(notifier=w2970) -> (current notification=w2969:bool)  [unwired: 1 in, 4 out]
        n1036 = Greater Than 0?(x=w2973) -> (x > 0?=w2972:bool)
        n1037 = case shown="True" w2972 {
          tunnel: w2979 -> [_ w3011]
          tunnel: w2978 -> [w2981 w3012]
          tunnel: [w2981 w3010] -> w2977
          tunnel: w2976 -> [_ w3007]
          tunnel: w2975 -> [_ w3006]
          tunnel: w2974 -> [_ w2996]
          tunnel: w2971 -> [_ w3005]
          tunnel: w2968 -> [w2980 w3002]
          tunnel: [w2980 w3001] -> w2967
          tunnel: w2966 -> [_ w3000]
          tunnel: w2965 -> [_ w2999]
          tunnel: w2964 -> [_ w2994]
          tunnel: w2962 -> [_ w2992]
          tunnel: w2961 -> [_ w2990]
          tunnel: w2960 -> [_ _]
          tunnel: w2959 -> [_ _]
          tunnel: w2958 -> [_ _]
          frame False {
          }
          frame True {
            # "True: Last Frame of frame accum"
            # "Current Line in Frame Accum"
            # "Current Line In Frame"
            n1038 = Increment(x=w3002) -> (x+1=w2995:u32)
            n1039 = Dequeue Element(queue=w3005) -> (element=w3018:u64[])  [unwired: 2 in, 3 out]
            n1040 = Equal?(x=w2995, y=w2999) -> (x = y?=w3004:bool)
            n1041 = Greater?(x=w2995, y=w3000) -> (0:w2997:bool)
            n1042 = Greater?(x=w2995, y=w2994) -> (0:w2993:bool)
            n1043 = Split Number(x=w3018) -> (hi(x)=w3019:u32[], lo(x)=w3017:u32[])
            n1044 = Split Number(x=w3019) -> (lo(x)=w2983:u16[])  [unwired: 1 out]
            n1045 = Split Number(x=w3017) -> (hi(x)=w2985:u16[], lo(x)=w2984:u16[])
            n1046 = Select(t=u32 0, s=w3004, f=w2995) -> (s? t:f=w3001:u32)
            n1047 = Increment(x=w3012) -> (x+1=w3014:i32)
            n1048 = Equal?(x=w3011, y=w3012) -> (x = y?=w3013:bool)
            n1049 = To Single Precision Float(number=w2983) -> (single precision float=w2989:sgl[])
            n1050 = To Single Precision Float(number=w2985) -> (single precision float=w2987:sgl[])
            n1051 = To Single Precision Float(number=w2984) -> (single precision float=w2988:sgl[])
            n1052 = Select(t=0, s=w3013, f=w3014) -> (s? t:f=w3010:i32)
            n1053 = Compound Arithmetic op=ADD(w2989, w2987, w2988) -> (w2986:sgl[])
            n1054 = Build Array(0, w3012, w3011, w3012) -> (w3009:i32[])
            n1055 = case shown="False" w2993 {
              tunnel: [w3027 w3033] -> w3008
              tunnel: w3009 -> [_ w3031]
              tunnel: w3006 -> [w3026 w3030]
              tunnel: w2992 -> [w3025 w3029]
              tunnel: [w3025 w3029] -> w2991
              tunnel: w2986 -> [w3024 w3028]
              frame False {
                n1056 = Divide(x=w3024, y=w3026) -> (x/y=w3027:sgl[])
              }
              frame True {
                n1057 = call "IMAQ GetPixelLine"("Line Coordinates"=w3031, "Image"=w3029) -> ("Pixels Line (Float)"=w3032:sgl[])  [unwired: 2 in, 4 out]
                n1058 = Divide(x=w3028, y=w3030) -> (x/y=w3034:sgl[])
                n1059 = Add(x=w3032, y=w3034) -> (x+y=w3033:sgl[])
              }
            }
            n1060 = call "IMAQ SetPixelLine"("Pixels Line (Float)"=w3008, "Line Coordinates"=w3009, "Image"=w2991) -> ()  [unwired: 7 in, 2 out]
            n1061 = To Unsigned Word Integer(number=w3008) -> (unsigned 16bit integer=w2982:u16[])
            n1062 = And(x=w2997, y=w2996) -> (x .and. y?=w2998:bool)
            n1063 = case shown="True" w2998 {
              tunnel: w2982 -> [_ w3023]
              tunnel: w3007 -> [_ w3021]
              tunnel: w2990 -> [_ w3020]
              frame False {
              }
              frame True {
                n1064 = Write to Binary File(file (use dialog)=w3020, data=w3023, 5:FALSE ("prepend array or string size? (T)"), 9:w3021) -> ()  [unwired: 2 in, 3 out]
              }
            }
          }
        }
      }
    }
    frame 31 {
      n1065 = while {
        shift-right: [w3070] -> _
        shift-left: 0 -> [w3071]
        tunnel: w3049 -> [w3072]
        tunnel: w3048 -> [w3069]
        tunnel: w3047 -> [w3068]
        tunnel: w3046 -> [w3067]
        tunnel: w3045 -> [w3063]
        shift-right: [w3060] -> _
        shift-left: u32 0 -> [w3061]
        tunnel: w3043 -> [w3059]
        tunnel: w3042 -> [w3058]
        tunnel: w3041 -> [w3057]
        tunnel: w3040 -> [w3056]
        tunnel: w3035 -> [w3055]
        tunnel: w3039 -> [w3054]
        tunnel: w3038 -> [w3053]
        tunnel: w3037 -> [w3052]
        tunnel: w3036 -> [w3051]
        stop <- w3062 stop-if-true
        n1066 = Get Queue Status(queue=w3056) -> (queue out=w3064:refnum<queue>, # elements in queue=w3066:i32)  [unwired: 2 in, 6 out]
        n1067 = Get Notifier Status(notifier=w3063) -> (current notification=w3062:bool)  [unwired: 1 in, 4 out]
        n1068 = Greater Than 0?(x=w3066) -> (x > 0?=w3065:bool)
        n1069 = case shown="True" w3065 {
          tunnel: w3072 -> [_ w3106]
          tunnel: w3071 -> [w3074 w3107]
          tunnel: [w3074 w3105] -> w3070
          tunnel: w3069 -> [_ w3102]
          tunnel: w3068 -> [_ w3101]
          tunnel: w3067 -> [_ w3091]
          tunnel: w3064 -> [_ w3100]
          tunnel: w3061 -> [w3073 w3097]
          tunnel: [w3073 w3096] -> w3060
          tunnel: w3059 -> [_ w3095]
          tunnel: w3058 -> [_ w3094]
          tunnel: w3057 -> [_ w3089]
          tunnel: w3055 -> [_ w3087]
          tunnel: w3054 -> [_ w3085]
          tunnel: w3053 -> [_ _]
          tunnel: w3052 -> [_ _]
          tunnel: w3051 -> [_ _]
          frame False {
          }
          frame True {
            # "True: Last Frame of frame accum"
            # "Current Line in Frame Accum"
            # "Current Line In Frame"
            n1070 = Increment(x=w3097) -> (x+1=w3090:u32)
            n1071 = Dequeue Element(queue=w3100) -> (element=w3113:u64[])  [unwired: 2 in, 3 out]
            n1072 = Equal?(x=w3090, y=w3094) -> (x = y?=w3099:bool)
            n1073 = Greater?(x=w3090, y=w3095) -> (0:w3092:bool)
            n1074 = Greater?(x=w3090, y=w3089) -> (0:w3088:bool)
            n1075 = Split Number(x=w3113) -> (hi(x)=w3114:u32[], lo(x)=w3112:u32[])
            n1076 = Split Number(x=w3114) -> (hi(x)=w3079:u16[], lo(x)=w3078:u16[])
            n1077 = Split Number(x=w3112) -> (hi(x)=w3077:u16[], lo(x)=w3076:u16[])
            n1078 = Select(t=u32 0, s=w3099, f=w3090) -> (s? t:f=w3096:u32)
            n1079 = Increment(x=w3107) -> (x+1=w3109:i32)
            n1080 = Equal?(x=w3106, y=w3107) -> (x = y?=w3108:bool)
            n1081 = To Single Precision Float(number=w3079) -> (single precision float=w3084:sgl[])
            n1082 = To Single Precision Float(number=w3078) -> (single precision float=w3082:sgl[])
            n1083 = To Single Precision Float(number=w3077) -> (single precision float=w3083:sgl[])
            n1084 = To Single Precision Float(number=w3076) -> (single precision float=w3080:sgl[])
            n1085 = Select(t=0, s=w3108, f=w3109) -> (s? t:f=w3105:i32)
            n1086 = Compound Arithmetic op=ADD(w3084, w3082, w3083, w3080) -> (w3081:sgl[])
            n1087 = Build Array(0, w3107, w3106, w3107) -> (w3104:i32[])
            n1088 = case shown="False" w3088 {
              tunnel: [w3122 w3128] -> w3103
              tunnel: w3104 -> [_ w3126]
              tunnel: w3101 -> [w3121 w3125]
              tunnel: w3087 -> [w3120 w3124]
              tunnel: [w3120 w3124] -> w3086
              tunnel: w3081 -> [w3119 w3123]
              frame False {
                n1089 = Divide(x=w3119, y=w3121) -> (x/y=w3122:sgl[])
              }
              frame True {
                n1090 = call "IMAQ GetPixelLine"("Line Coordinates"=w3126, "Image"=w3124) -> ("Pixels Line (Float)"=w3127:sgl[])  [unwired: 2 in, 4 out]
                n1091 = Divide(x=w3123, y=w3125) -> (x/y=w3129:sgl[])
                n1092 = Add(x=w3127, y=w3129) -> (x+y=w3128:sgl[])
              }
            }
            n1093 = call "IMAQ SetPixelLine"("Pixels Line (Float)"=w3103, "Line Coordinates"=w3104, "Image"=w3086) -> ()  [unwired: 7 in, 2 out]
            n1094 = To Unsigned Word Integer(number=w3103) -> (unsigned 16bit integer=w3075:u16[])
            n1095 = And(x=w3092, y=w3091) -> (x .and. y?=w3093:bool)
            n1096 = case shown="True" w3093 {
              tunnel: w3075 -> [_ w3118]
              tunnel: w3102 -> [_ w3116]
              tunnel: w3085 -> [_ w3115]
              frame False {
              }
              frame True {
                n1097 = Write to Binary File(file (use dialog)=w3115, data=w3118, 5:FALSE ("prepend array or string size? (T)"), 9:w3116) -> ()  [unwired: 2 in, 3 out]
              }
            }
          }
        }
      }
    }
  }
  n1098 = Flush Queue(queue=w23) -> (queue out=w67:refnum<queue>)  [unwired: 1 in, 2 out]
  n1099 = Release Queue(queue=w67) -> ()  [unwired: 2 in, 3 out]
  n1100 = while {
    tunnel: w81 -> [w3150]
    shift-right: [w3132] -> _
    shift-left: u32 0 -> [w3131]
    tunnel: w107 -> [w3130]
    shift-right: [w3146] -> _
    shift-left: FALSE -> [w3145]
    tunnel: w24 -> [w3144]
    shift-right: [w3142] -> _
    shift-left: u32 0 -> [w3143]
    tunnel: w102 -> [w3138]
    tunnel: w20 -> [w3135]
    tunnel: [w3133] -> w82
    shift-right: [w3134] -> w96
    shift-left: w42 -> [w3151]
    stop <- w3141 stop-if-true
    # "Total Lines Counter"
    n1101 = xnode "Invoke Method"("FPGA VI Reference In"=w3150, "Number of Elements"=w3131, "Timeout (ms)"=0) -> ("FPGA VI Reference Out"=w3133:refnum<k20>, "Data"=w3139:u64[], "Elements Remaining"=w3148:u32)  [unwired: 1 in, 1 out]
    n1102 = Get Notifier Status(notifier=w3151) -> (notifier out=w3134:refnum<notifier>, current notification=w3140:bool)  [unwired: 1 in, 3 out]
    n1103 = case shown="True" w3145 {
      tunnel: w3139 -> [_ w3155]
      tunnel: w3144 -> [_ w3160]
      tunnel: w3143 -> [w3153 w3158]
      tunnel: [w3153 w3154] -> w3142
      tunnel: [w3152 w3157] -> w3137
      tunnel: w3140 -> [w3152 _]
      tunnel: w3138 -> [_ w3156]
      frame False {
      }
      frame True {
        n1104 = Increment(x=w3158) -> (x+1=w3154:u32)
        n1105 = Enqueue Element(queue=w3160, element=w3155, timeout in ms (-1)=0) -> ()  [unwired: 1 in, 3 out]
        n1106 = Equal?(x=w3154, y=w3156) -> (x = y?=w3157:bool)
      }
    }
    n1107 = Greater Or Equal?(x=w3148, y=w3130) -> (x >= y?=w3146:bool)
    n1108 = Select(t=w3130, s=w3146, f=u32 0) -> (s? t:f=w3132:u32)
    n1109 = And(x=w3135, y=w3137) -> (x .and. y?=w3136:bool)
    n1110 = Or(x=w3136, y=w3140) -> (x .or. y?=w3141:bool)
  }
  n1111 = xnode "Close FPGA VI Reference"("FPGA VI Reference In"=w82) -> ()  [unwired: 1 in, 1 out]
  n1112 = Send Notification(notification=TRUE, notifier=w96) -> ()  [unwired: 1 in, 2 out]
